vi "mainHRScan.vi"() -> ()   [LabVIEW 2024]
doc: "Main VI for FLS imaging system."
uses:
  <userlib>/_OpenG.lib/file/file.llb/openg_file.lvlib
  <vilib>/event_ctls.llb/usereventprio.ctl
  <instrlib>/niScope/Acquire/Fetch/niScope Multi Fetch Binary 16.vi
  <instrlib>/niScope/Controls/niScope trigger source.ctl
  <userlib>/_OpenG.lib/time/time.llb/openg_time.lvlib
  LaguerreDeconLib/DeconEngineClass/LaguerreDeconEngineClass.lvclass
  SubVI/GlobalVariables.vi
  SubVI/LabJack/LJ Pin Setting.ctl
  <vilib>/Utility/error.llb/DialogType.ctl
  <vilib>/Analysis/NI_AALBase.lvlib
  <vilib>/Utility/miscctls.llb/LVMinMaxIncTypeDef.ctl
  <vilib>/Analysis/baseanly.llb/Mean (DBL).vi
  <vilib>/Utility/miscctls.llb/LVPointTypeDef.ctl
  SubVI/APD/APDClass.lvclass
  ConfigFiles/AimingBeamVideoConfig.ctl
  <instrlib>/niScope/Controls/niScope vertical coupling.ctl
  <vilib>/Instr/_visa.llb/VISA Configure Serial Port (Instr).vi
  <instrlib>/niScope/Configure/Trigger/niScope Configure Trigger Software.vi
  <instrlib>/niScope/Acquire/Fetch/niScope Fetch Binary 8.vi
  SubVI/DigitizerConfiguration/FLImDAQ.ctl
panel:
  out "WF saved":i32
  out "EncoderGraph":dbl[](graph)
  out "error out 3":errorcluster
  out "error out 2":errorcluster
  out "error out":errorcluster
  out "Record Backlog 2":i32
  out "RunStartTime":u32
  out "Dig1 Temp":dbl
  out "Dig2 Temp":dbl
  out "Visualization PC video source":T1
  out "SNR3":dbl format="%#_3g"
  out "SNR2":dbl format="%#_3g"
  out "SNR1":dbl format="%#_3g"
  in  "Show BG removed?":bool=TRUE
  out "IntR3":dbl format="%#_2g"
  out "IntR2":dbl format="%#_2g"
  out "IntR1":dbl format="%#_2g"
  out "Gain3":dbl
  out "Gain2":dbl
  out "Gain1":dbl
  in  "Skip Data Save?":bool=TRUE
  out "Aq Loop?":bool
  out "ML?":bool
  out "aquisition loop Error Out":errorcluster
  out "Record Backlog 1":i32 caption="Record Backlog"
  out "Fetch Record #":i32
  out "Disclamer":picture
  out "Calibration #":i8
  out "BG #":i8
  out "Help":string
  in  "355nm Laser toggle":bool caption="355nm 2500Hz"
  in  "Cali&iRF alignment":bool
  in  "Background":bool
  in  "Aiming beam toggle":bool caption="445nm 15Hz 15mA"
  out "Run #":i8
  in  "StopButton":bool caption="Stop"
  out "Aquisition Status:":bool
  in  "StartButton":bool caption="Start"
  in  "V 3":dbl=1.0 caption="Gain 3" min=0.0 max=4.6494 step=0.1
  in  "V 2":dbl=1.0 caption="Gain 2" min=0.0 max=4.61 step=0.1
  in  "V 1":dbl=1.0 caption="Gain 1" min=0.0 max=4.6492 step=0.1 format="%#_4g"
  out "Case #":string
  out "System Hardware Connection Status":T2
  out "Channel 3":dbl[][](graph)
  out "Channel 2":dbl[][](graph)
  out "Channel 1":dbl[][](graph)
  in  "Tab Control":T3(tab)
  out "display loop timing(ms)":u32
  out "Aquisition loop timing(ms)":u32 format="%.2f"
  out "DisplayLoopIdx":i32 caption="DisplayLoop"
  out "laser EM lamp V":dbl format="%0.6f"
  out "Auisition Loop idx":i32
  out "DataTransferTime":u32
  in  "EncoderDAQ name":refnum<k15>="PXI1Slot2"
  in  "channels":string="0"
  in  "input impedance":u32(ring) items=["1 mega ohm"=0, "50 ohms"=2]
  in  "vertical range":dbl=10.0 format="%.2f"
  in  "min sample rate":dbl=50000.0 format="%^.2e"
  in  "EncoderSampleInterval(s)":dbl=1.0
  out "EncoderDataLength":u32
  in  "Show BG":bool
  out "iRF length":i32
  out "BG length":i32
  out "data length":i32
  out "SysConfigCluster":T4
  out "LJ Pinout":T5={"Ch1 Bias"="DAC0", "Ch2 Bias"="DAC1", "Ch3 Bias"="DAC2", "Ch4 Bias"="DAC0", "355 PWM"="FIO0", "AimingBeam PWM"="FIO2", "Laser Ready"="FIO3", "Interlock"="FIO1", "Laser Start/Stop"="FIO1", "Red LED"="FIO1", "Green LED"="DIO3", "Foot Pedal"="DIO15"}
  out "FLImDAQ":T6={"Digitizer 1"="", "Digitizer 2"="", "Channel"=enum."Channel 0", "trigger source"="VAL_EXTERNAL", "trigger level"=0.5, "trigger delay"=1.35e-07, "min sample rate"=12500000000.0, "min record length"=2500, "vertical range"=1.0, "vertical offset"=-0.25, "Waveform to Avg"=2000} caption="FLIm DAQ Configuration" {"trigger delay" format="%^#.4e"; "trigger level" min=0.0 max=3.5 step=0.5 format="%.2f"; "vertical offset" format="%.4f"; "vertical range" format="%.2f"; "min sample rate" format="%#.2p"}
  in  "Sys Reconfig":bool
  out "Vertical Range 1":dbl
  out "Vertical Offset 1":dbl
  out "Vertical Range 2":dbl
  out "Vertical Offset 2":dbl
  out "Laser Rep Rate":dbl
  in  "Data Class":enum16{"Data", "BG", "Cali"}(ring)
  out "V1 Size":i32
  out "V2 Size":i32
  out "V3 Size":i32
  out "data Size":i32[](array[numeric])
  out "State log":string
  in  "Quit":bool
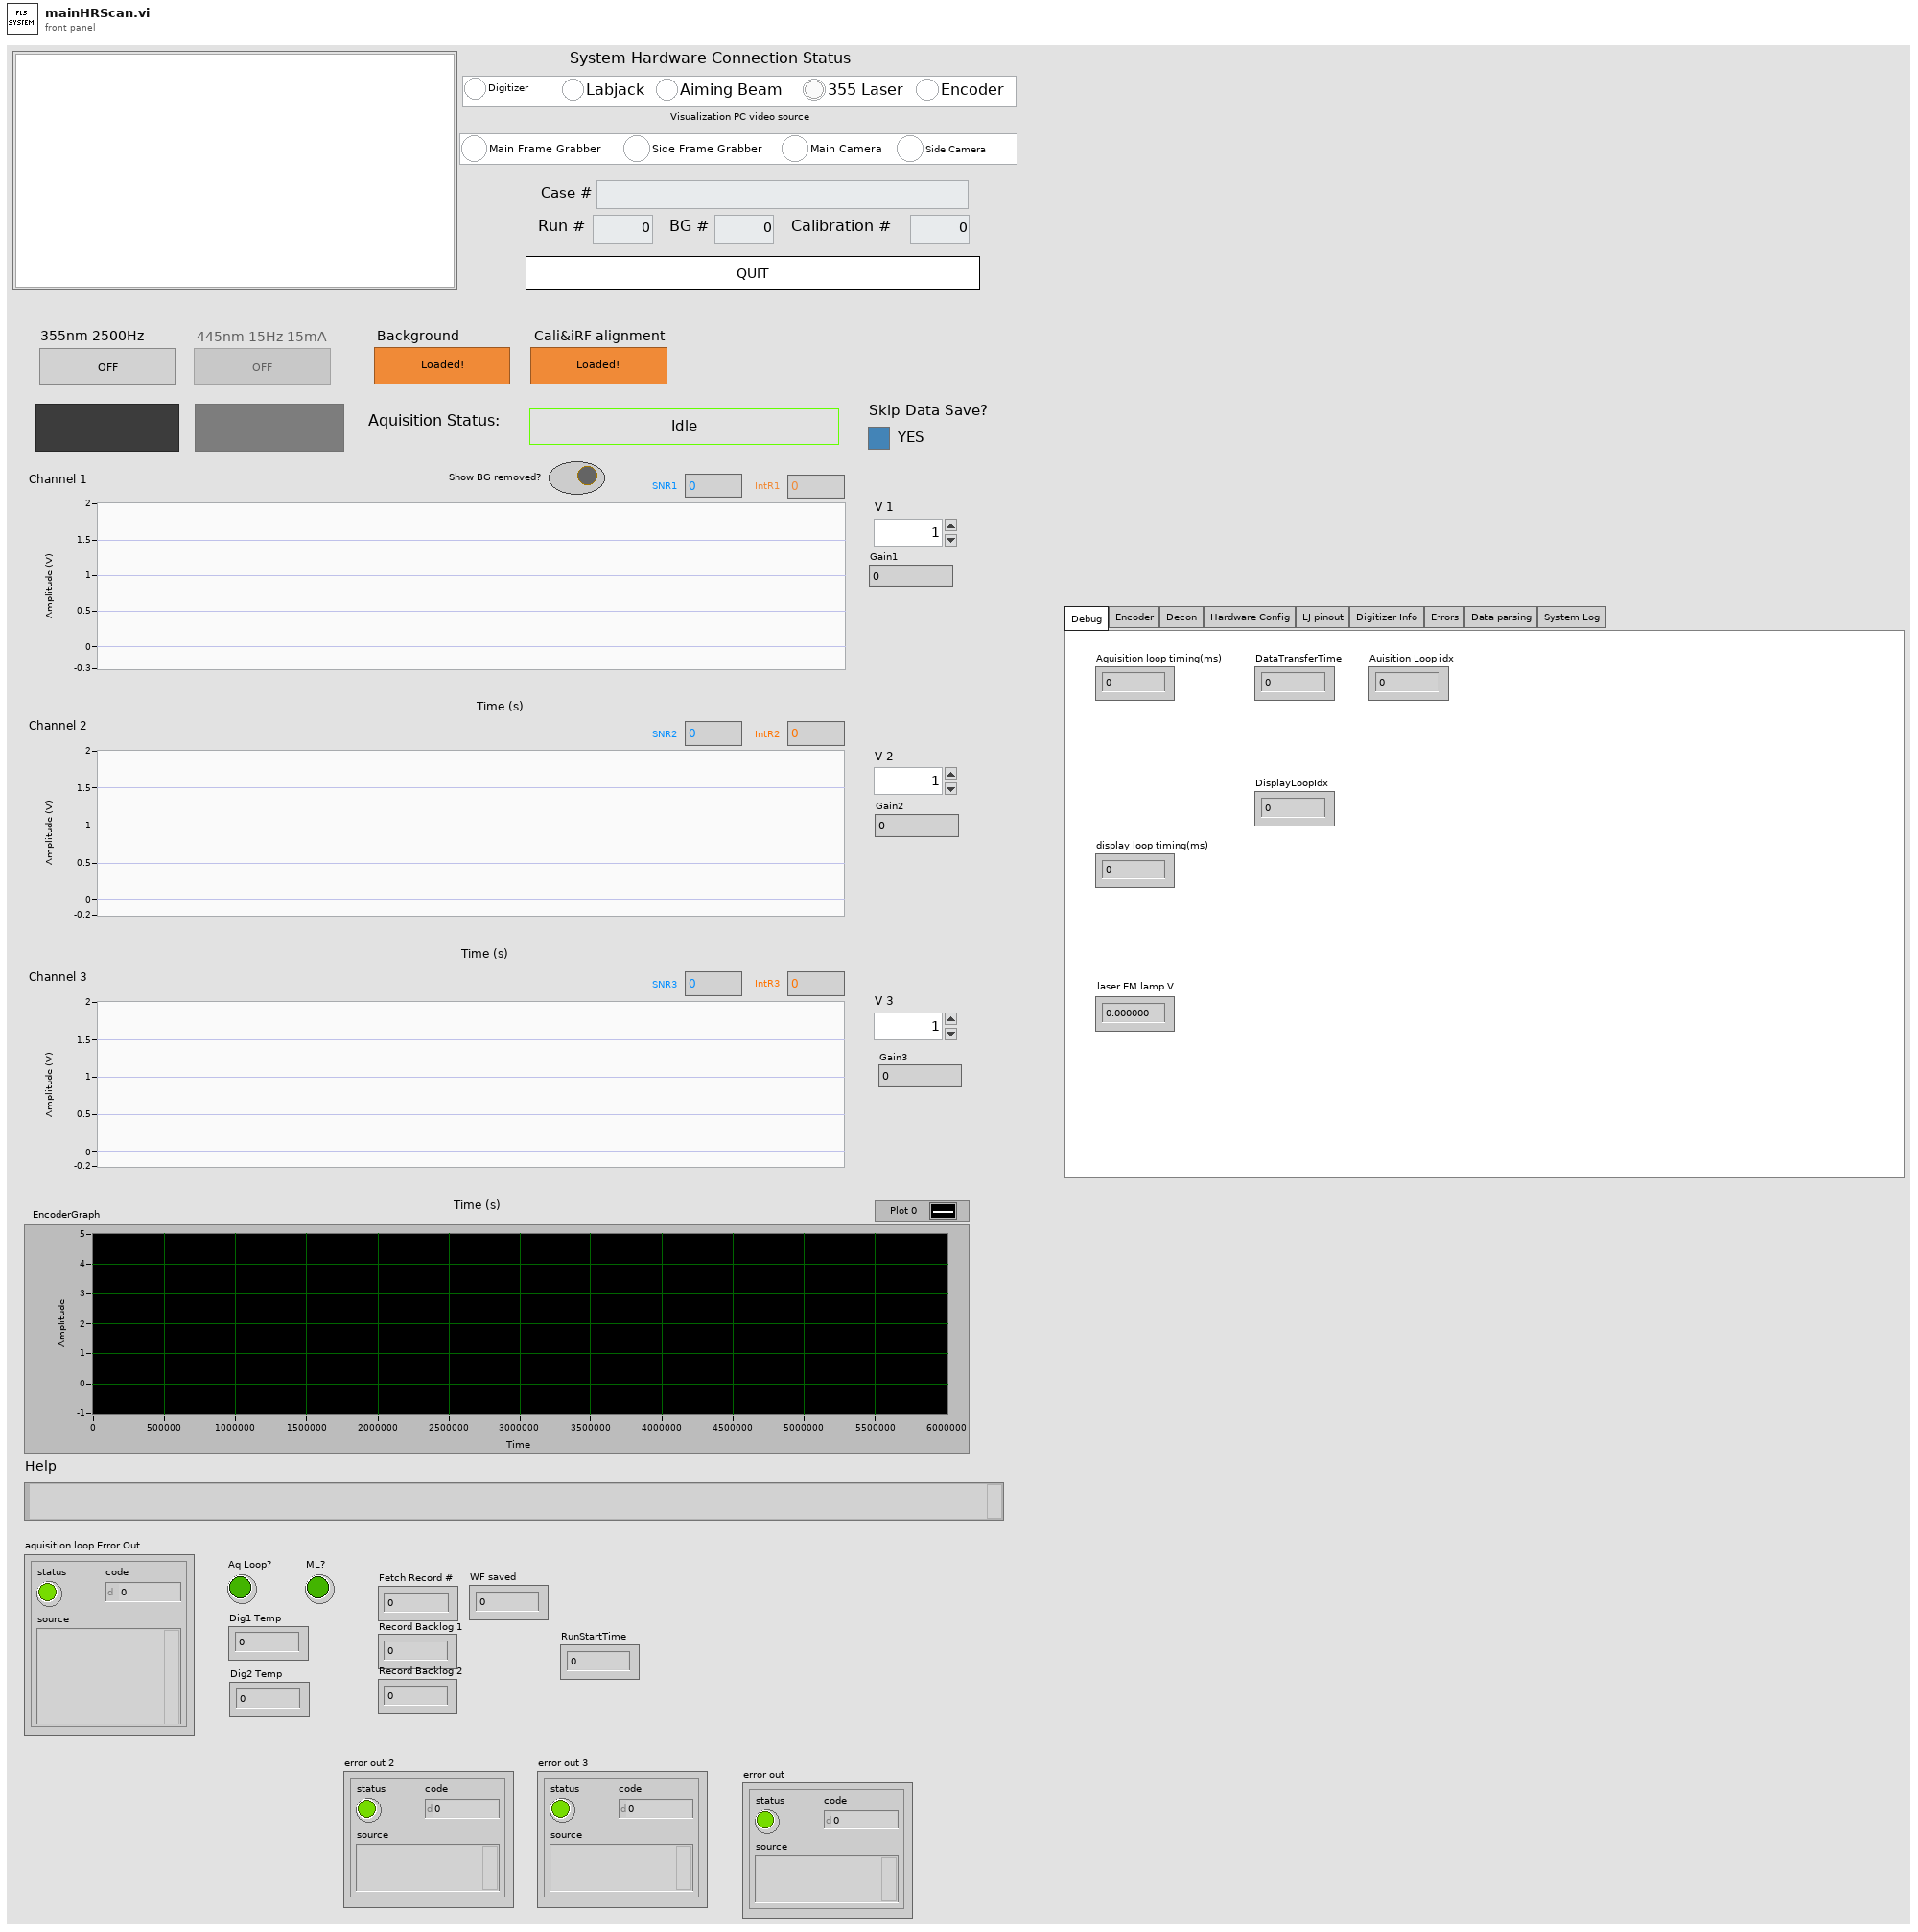
[diagram p1: front panel]
types:
  T1 = cluster{"Main Frame Grabber":bool, "Side Frame Grabber":bool, "Main Camera":bool, "Side Camera":bool}
  T2 = cluster{"Digitizer":bool, "Labjack":bool, "Aiming Beam":bool, "355 Laser":bool, "Encoder":bool}
  T3 = enum32{"Debug", "Encoder", "Decon", "Hardware Config", "LJ pinout", "Digitizer Info", "Errors", "Data parsing", "System Log"}
  T4 = cluster{"Ch1Enable?":bool, "Ch2Enable?":bool, "Ch3Enable?":bool, "Ch1AutoGain?":bool, "Ch2AutoGain?":bool, "Ch3AutoGain?":bool, "AimingBeamEnable?":bool}
  T5 = typedef "LJ Pin Setting.ctl" = cluster{"Ch1 Bias":string, "Ch2 Bias":string, "Ch3 Bias":string, "Ch4 Bias":string, "355 PWM":string, "AimingBeam PWM":string, "Laser Ready":string, "Interlock":string, "Laser Start/Stop":string, "Red LED":string, "Green LED":string, "Foot Pedal":string}
  T6 = typedef "FLImDAQ.ctl" = cluster{"Digitizer 1":refnum<k15>, "Digitizer 2":refnum<k15>, "Channel":enum16{"Channel 0", "Channel 1", "Channel 0&1"}, "trigger source":T7, "trigger level":dbl, "trigger delay":dbl, "min sample rate":dbl, "min record length":i32, "vertical range":dbl, "vertical offset":dbl, "Waveform to Avg":i16}
  T7 = typedef "niScope trigger source.ctl" = string
  T8 = cluster{"remote start event":refnum<user-event>, "remote stop  event":refnum<user-event>}
  T9 = enum16{"open", "replace", "create", "open or create", "replace or create", "replace or create with confirmation"}
  T10 = cluster{"idx":i32, "CH1&2":i16[][], "CH3":i16[][], "V cluster":cluster{"V1":dbl, "V2":dbl, "V3":dbl}}
  T11 = cluster{"Ch1 WF":dbl[], "Ch2 WF":dbl[], "Ch3 WF":dbl[], "V1":dbl, "V2":dbl, "V3":dbl}
  T12 = enum16{"open", "open or create", "create or replace", "create", "open (read-only)"}
  T13 = enum32{"Invalid", "Standard", "Closed", "Hidden", "Minimized", "Maximized"}
  T14 = enum32{"invalid app kind", "Development System", "Run Time System", "Student Edition", "Embedded LabVIEW", "Evaluation", "Custom"}
  T15 = typedef "usereventprio.ctl" = enum32{"high priority", "normal priority"}
  T16 = enum32{"Bad", "Idle", "Run top level", "Running"}
  T17 = enum8{"Enabled", "Disabled", "Disabled and Grayed Out"}
  T18 = typedef "AimingBeamVideoConfig.ctl" = cluster{"DeCon Channel":enum16{"1", "2", "3"}, "Scale Bar":bool, "Scale Low":dbl, "Scale High":dbl, "ANSI":dbl, "Radius":dbl, "3D?":bool, "Firefly?":bool, "Pentero?":bool}
  T19 = cluster{"Core":cluster{"Current VI Reference":refnum<vi>, "Close Panel on Exit?":bool}, "SysConfigCluster":cluster{"Ch1Enable?":bool, "Ch2Enable?":bool, "Ch3Enable?":bool, "Ch1AutoGain?":bool, "Ch2AutoGain?":bool, "Ch3AutoGain?":bool, "AimingBeamEnable?":bool}, "System Status":cluster{"Digitizer":bool, "Labjack":bool, "Aiming Beam":bool, "355 Laser":bool, "Encoder":bool}, "IDs":cluster{"RunID":i8, "BG ID":i8, "Cali ID":i8}, "CaseID":string, "DefaultPath":path, "Pathes":cluster{"DataPath":path, "BG Path":path, "iRFPath":path, "CaliPath":path}, "FLImDAQ":cluster{"resource name":refnum<k15>, "resource name 2":refnum<k15>, "Channel":enum16{"Channel 0", "Channel 1", "Channel 0&1"}, "trigger source":T7, "trigger level":dbl, "trigger delay":dbl, "min sample rate":dbl, "min record length":i32, "vertical range":dbl, "vertical offset":dbl, "Waveform to Avg":i32}, "SysRunning?":bool, "AB Cluster":cluster{"Aiming Beam COM Port":refnum<visa-resource-name>, "Min Current":dbl, "Max Current":dbl, "Default Current":dbl, "Freq":i32}, "LJ Pinout":T5, "355 PWM setting":cluster{"DIO_EF_CLOCK1_DIVISOR":i16, "DIO_EF_CLOCK1_ROLL_VALUE":i32, "DIO#_EF_INDEX":i16, "DIO#_EF_OPTIONS":i16, "DIO#_EF_CONFIG_A":i32}, "AB PWM setting":cluster{"DIO_EF_CLOCK1_DIVISOR":i16, "DIO_EF_CLOCK1_ROLL_VALUE":i32, "DIO#_EF_INDEX":i16, "DIO#_EF_OPTIONS":i16, "DIO#_EF_CONFIG_A":i32}, "Last Trigger":u32, "niTClk sessions":refnum<k20>[], "Laser start tic":u32, "TCP attempt count":i32, "Ch1Data":dbl[][], "Ch2Data":dbl[][], "Ch3Data":dbl[][], "V1":dbl[], "V2":dbl[], "V3":dbl[], "SlowTimer":u32, "FastTimer":u32, "listener ID":refnum<k5>, "TempPath":path, "LED vi reference":refnum<vi>, "Aquisition Timer":u32, "APDSerialNum":cluster{"Ch1APDSerial#":string, "Ch2APDSerial#":string, "Ch3APDSerial#":string}, "VideoConfig":T18, "CaliPath":path, "LED vi ref open?":bool, "video source":cluster{"Main Frame Grabber":bool, "Side Frame Grabber":bool, "Main Camera":bool, "Side Camera":bool}, "bothVidSourceAvail":bool, "EncoderDAQ":refnum<k15>, "TDMS group name":string}
  T20 = typedef "LVCursorListTypeDef.ctl" = cluster{"Name":string, "Color":u32, "Style":u8, "Point Style":u8, "Name Visible":bool, "Allow Drag":bool, "Cursor Mode":u32, "Plot":i32, "Index":i32, "Position":cluster{"X":dbl, "Y":dbl}, "X Scale":u32, "Y Scale":u32, "Watch Plots":i32[], "Watch All Plots":bool, "Plot Area":i32, "Label Offset":cluster{"X":dbl, "Y":dbl}}[]
  T21 = cluster{"Name":string, "Color":u32, "Style":u8, "Point Style":u8, "Name Visible":bool, "Allow Drag":bool, "Cursor Mode":u32, "Plot":i32, "Index":i32, "Position":cluster{"X":dbl, "Y":dbl}, "X Scale":u32, "Y Scale":u32, "Watch Plots":i32[], "Watch All Plots":bool, "Plot Area":i32, "Label Offset":cluster{"X":dbl, "Y":dbl}}
  T22 = cluster{"Ch1APDSerial#":string, "Ch2APDSerial#":string, "Ch3APDSerial#":string}
  T23 = cluster{"DataPath":path, "BG Path":path, "iRFPath":path, "CaliPath":path}
  T24 = cluster{"DIO_EF_CLOCK1_DIVISOR":i16, "DIO_EF_CLOCK1_ROLL_VALUE":i32, "DIO#_EF_INDEX":i16, "DIO#_EF_OPTIONS":i16, "DIO#_EF_CONFIG_A":i32}
  T25 = cluster{"Aiming Beam COM Port":refnum<visa-resource-name>, "Min Current":dbl, "Max Current":dbl, "Default Current":dbl, "Freq":i32}
  T26 = cluster{"resource name":refnum<k15>, "resource name 2":refnum<k15>, "Channel":enum16{"Channel 0", "Channel 1", "Channel 0&1"}, "trigger source":T7, "trigger level":dbl, "trigger delay":dbl, "min sample rate":dbl, "min record length":i32, "vertical range":dbl, "vertical offset":dbl, "Waveform to Avg":i32}
  T27 = cluster{"Current VI Reference":refnum<vi>, "Close Panel on Exit?":bool}
  T28 = typedef "iRFData.ctl" = cluster{"dt":dbl, "NumOfWFs":i32, "WFLength":i32, "iRFCtrlV":dbl[], "iRFWFsAvg":dbl[][], "iRFRaw":dbl[][]}
  T29 = cluster{"iRFWFsAvg":dbl[], "iRFWFsAvg":dbl[], "iRFWFsAvg":dbl[]}
  T30 = cluster{"V 1":dbl[], "V 2":dbl[], "V 3":dbl[], "V 4":dbl[]}
  T31 = cluster{"Channel 1":dbl[], "Channel 2":dbl[], "Channel 3":dbl[], "Channel 4":dbl[]}
  T32 = cluster{"DataPath":path, "CaseID":string, "RunID":i8, "Ch1Data":dbl[][], "Ch2Data":dbl[][], "Ch3Data":dbl[][], "V1":dbl[], "V2":dbl[], "V3":dbl[], "LaserRepRate":u32, "WFAverage":i16, "RunStartTime":u32}
  T33 = typedef "DialogType.ctl" = u16
  T34 = cluster{"Ch1 iRF":dbl[], "Ch2 iRF":dbl[], "Ch3 iRF":dbl[], "Ch4 iRF":dbl[]}
  T35 = cluster{"Ch1APDSerial#":string, "Ch2APDSerial#":string, "Ch3APDSerial#":string, "Ch4APDSerial#":string}
  T36 = typedef "LJ PWM Setting.ctl" = cluster{"DIO_EF_CLOCK1_DIVISOR":i16, "DIO_EF_CLOCK1_ROLL_VALUE":i32, "DIO#_EF_INDEX":i16, "DIO#_EF_OPTIONS":i16, "DIO#_EF_CONFIG_A":i32}
  T37 = typedef "AimingBeam.ctl" = cluster{"Aiming Beam COM Port":refnum<visa-resource-name>, "Min Current":dbl, "Max Current":dbl, "Default Current":dbl, "Frequency(Hz)":u32}
  T38 = cluster{"DC1":i32, "DC2":i32, "BG1":i32, "BG2":i32}
  T39 = typedef "LVMinMaxIncTypeDef.ctl" = cluster{"Minimum":dbl, "Maximum":dbl, "Increment":dbl}
  T40 = typedef "LVBoundsTypeDef.ctl" = cluster{"Width":u32, "Height":u32}
  T41 = typedef "imagedata.ctl" = cluster{"image type":i32, "image depth":i32, "image":u8[], "mask":u8[], "colors":u32[], "Rectangle":cluster{"left":i16, "top":i16, "right":i16, "bottom":i16}}
  T42 = cluster{"DC Idx1":i32, "DC Idx2":i32, "BG Idx1":i32, "BG Idx2":i32}
  T43 = typedef "niScope vertical coupling.ctl" = i32
  T44 = cluster{"actualSamples":i32, "absoluteInitialX":dbl, "relativeInitialX":dbl, "xIncrement":dbl, "offset":dbl, "gain":dbl, "reserved1":dbl, "reserved2":dbl}
  T45 = typedef "LVPointTypeDef.ctl" = cluster{"Horizontal":i16, "Vertical":i16}
  T46 = cluster{"V1 out":dbl, "V2 out":dbl, "V3 out":dbl}
  T47 = cluster{i32, i16[][], i16[][], cluster{"V1 out":dbl, "V2 out":dbl, "V3 out":dbl}}
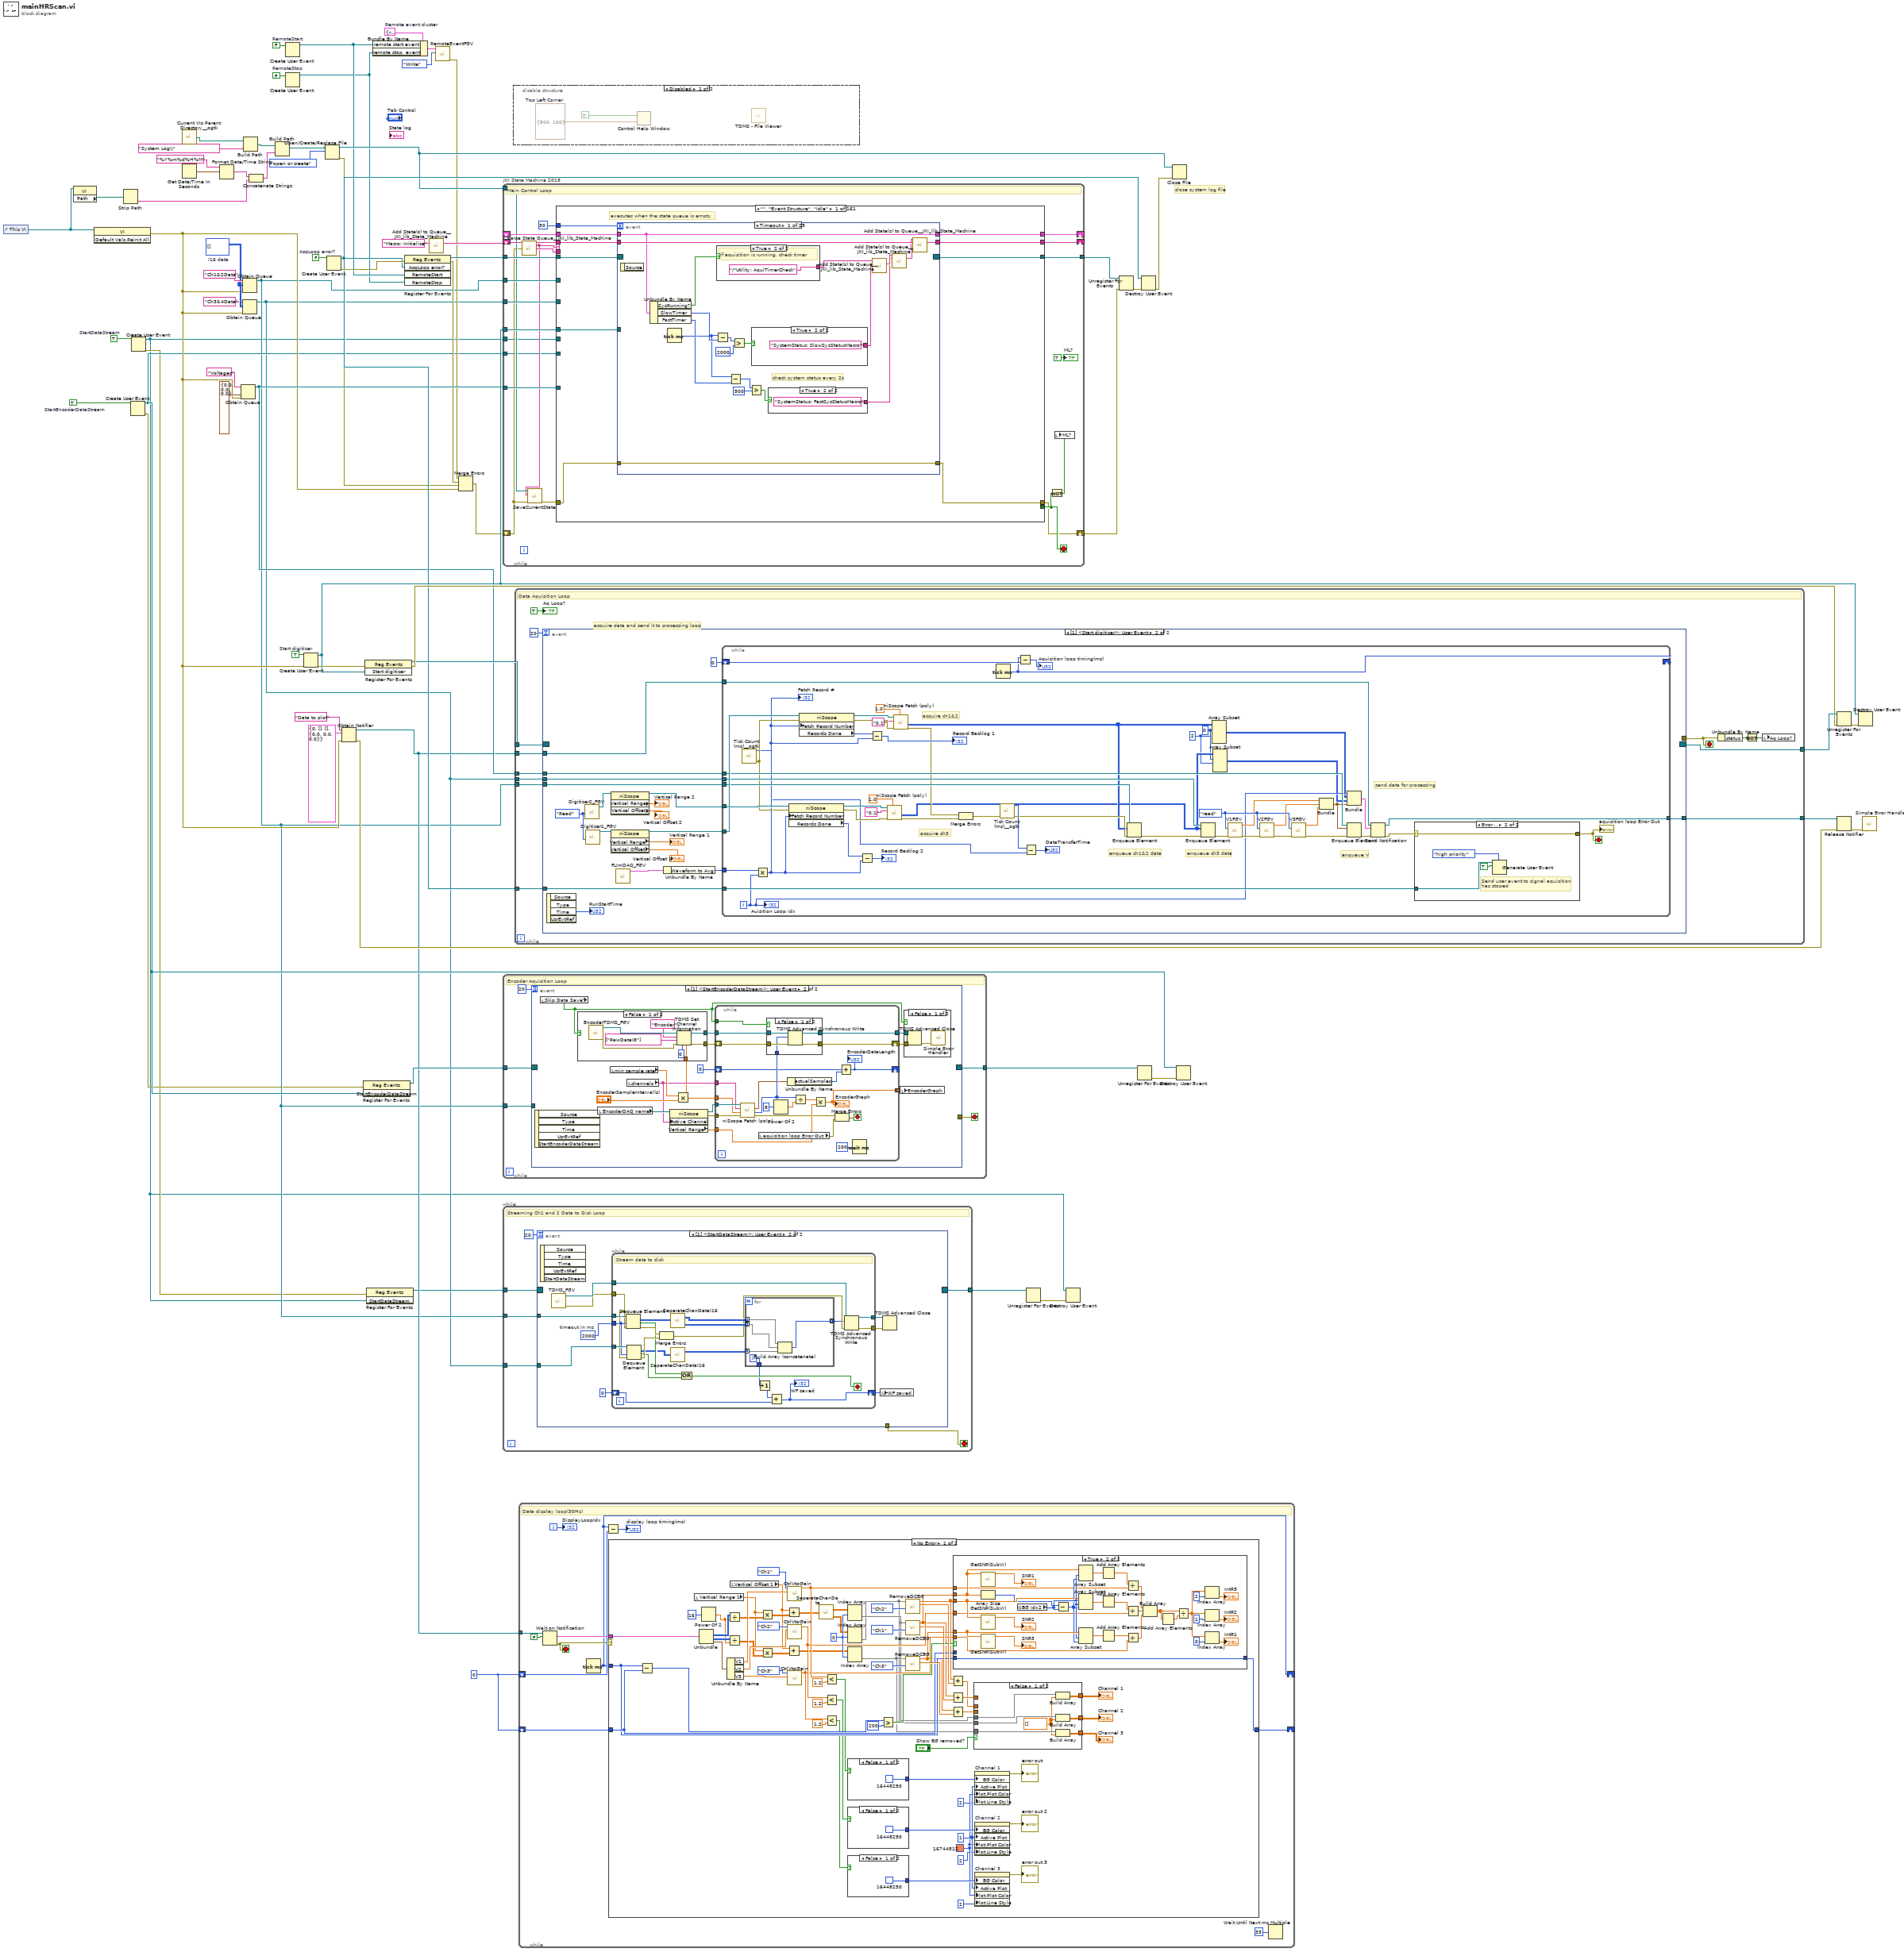
[diagram p0: block diagram]
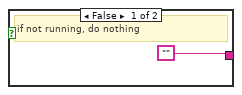
[diagram p2: hidden frame]
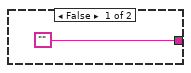
[diagram p3: hidden frame]
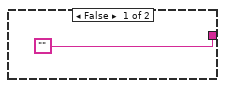
[diagram p4: hidden frame]
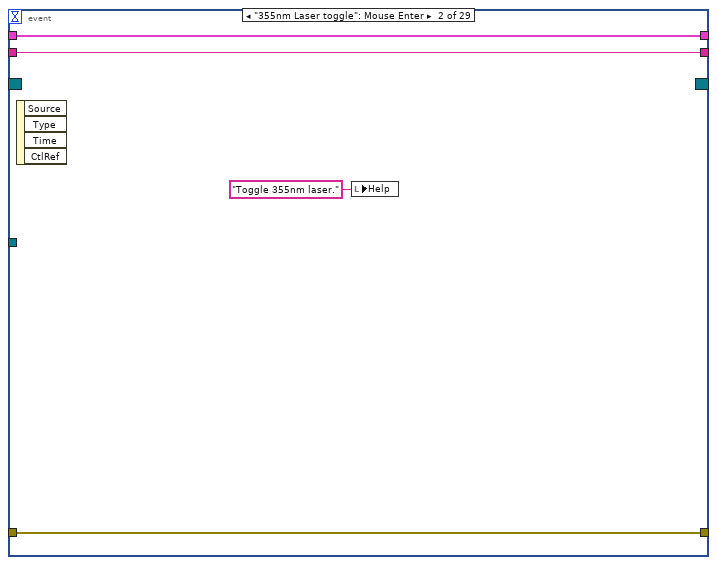
[diagram p5: hidden frame]
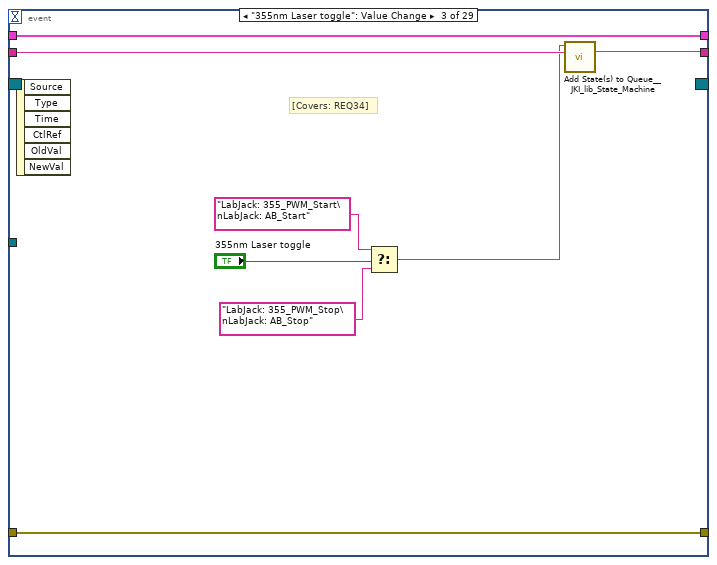
[diagram p6: hidden frame]
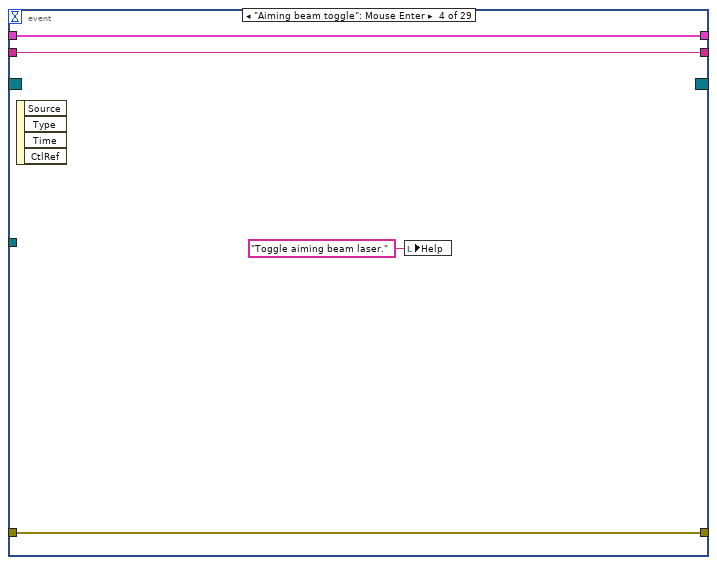
[diagram p7: hidden frame]
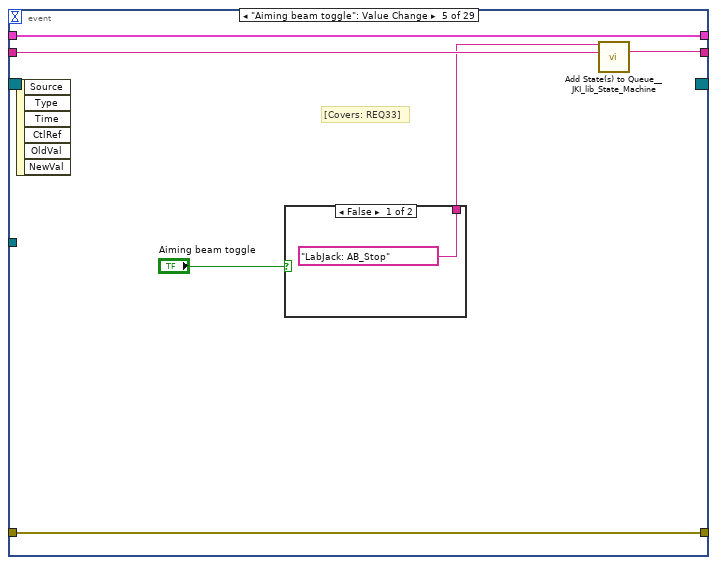
[diagram p8: hidden frame]
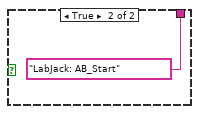
[diagram p9: hidden frame]
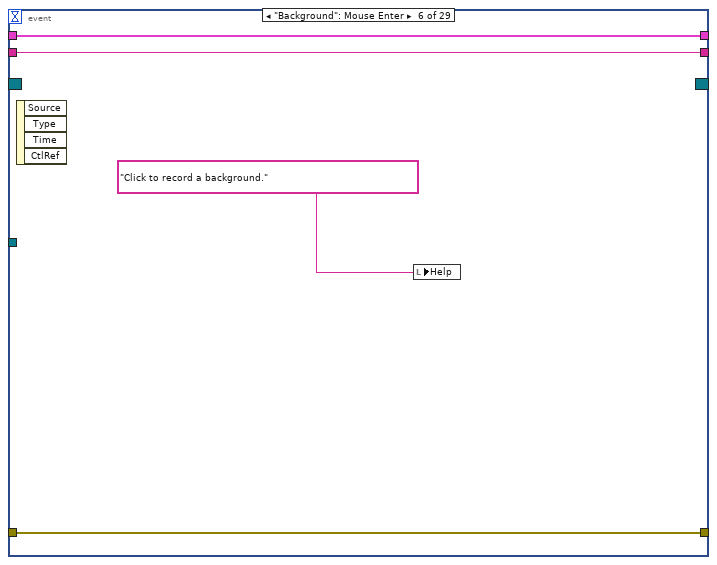
[diagram p10: hidden frame]
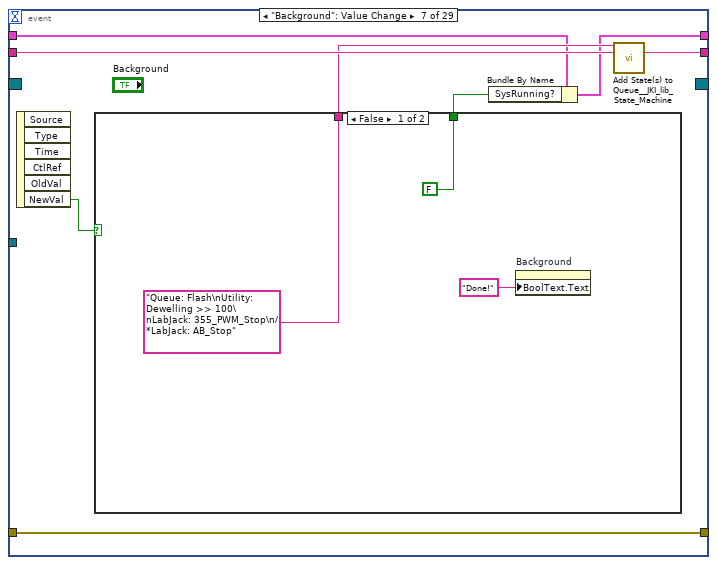
[diagram p11: hidden frame]
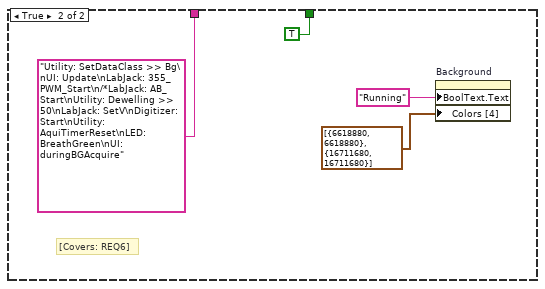
[diagram p12: hidden frame]
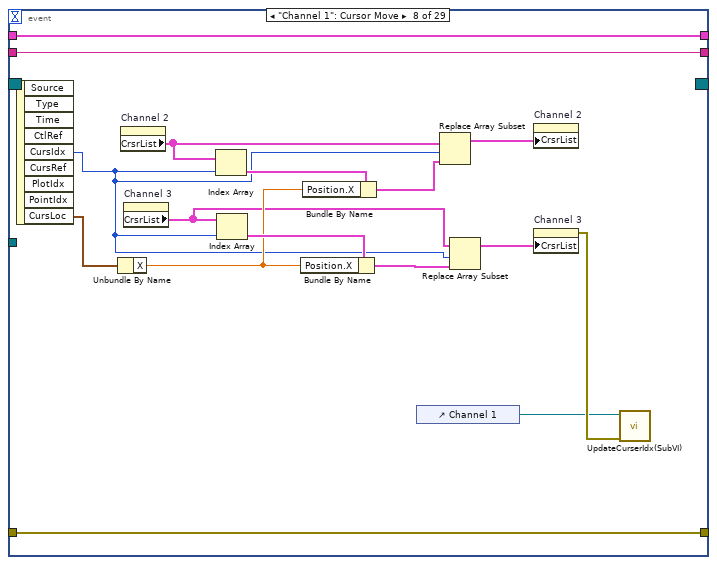
[diagram p13: hidden frame]
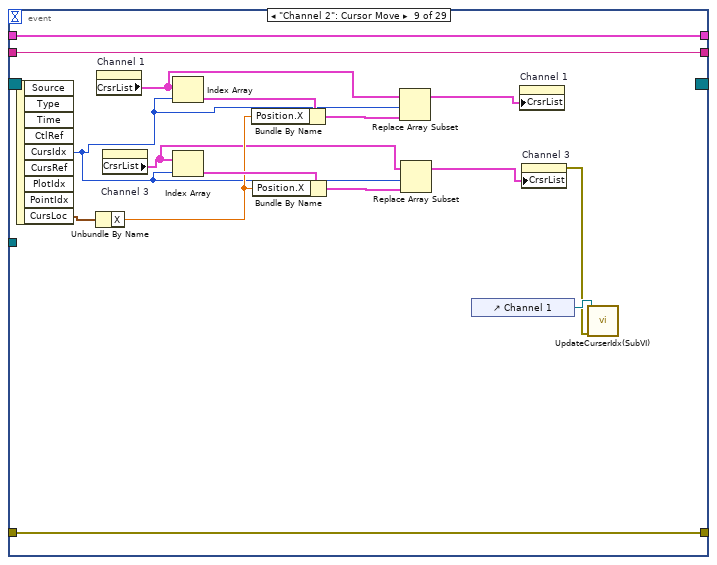
[diagram p14: hidden frame]
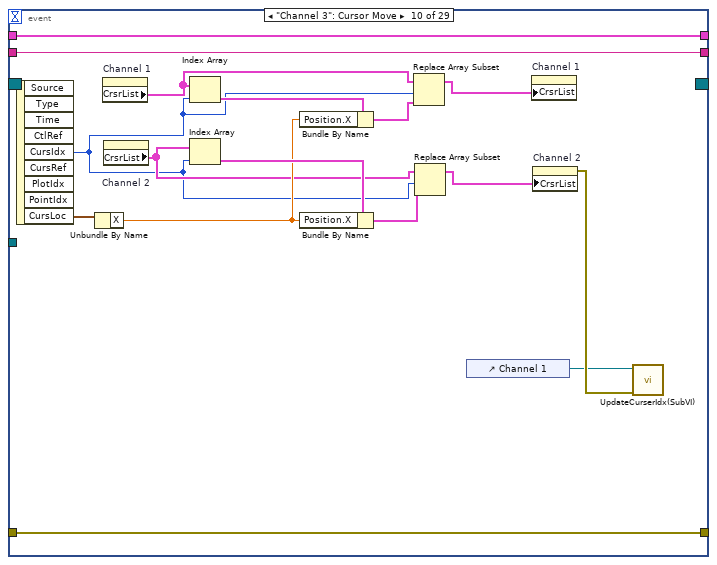
[diagram p15: hidden frame]
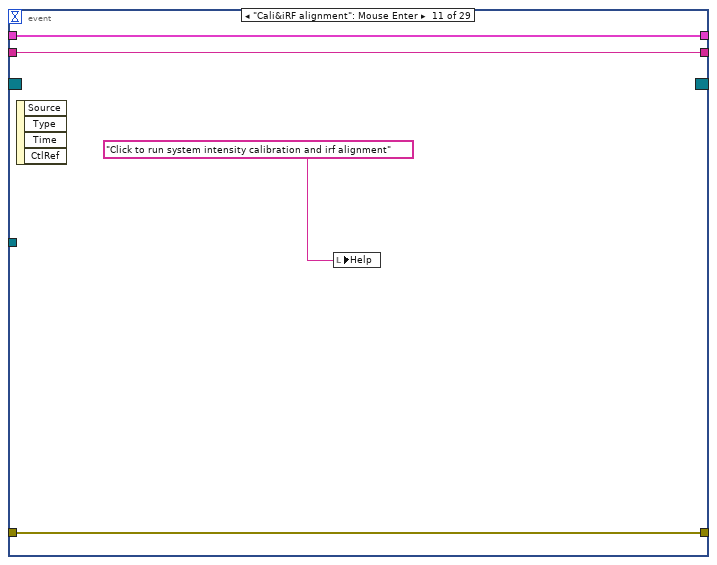
[diagram p16: hidden frame]
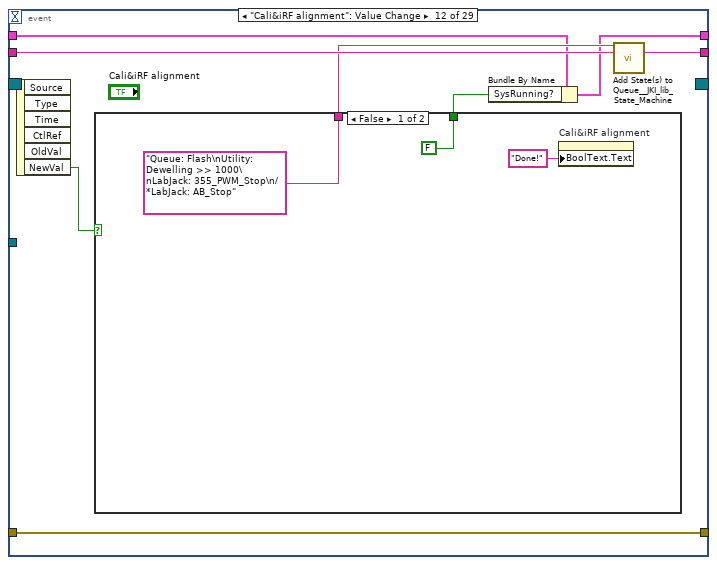
[diagram p17: hidden frame]
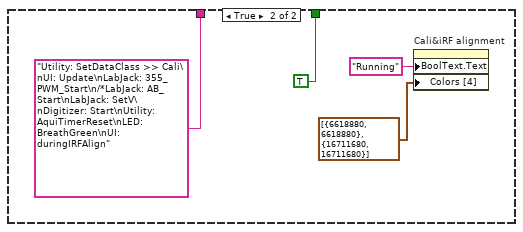
[diagram p18: hidden frame]
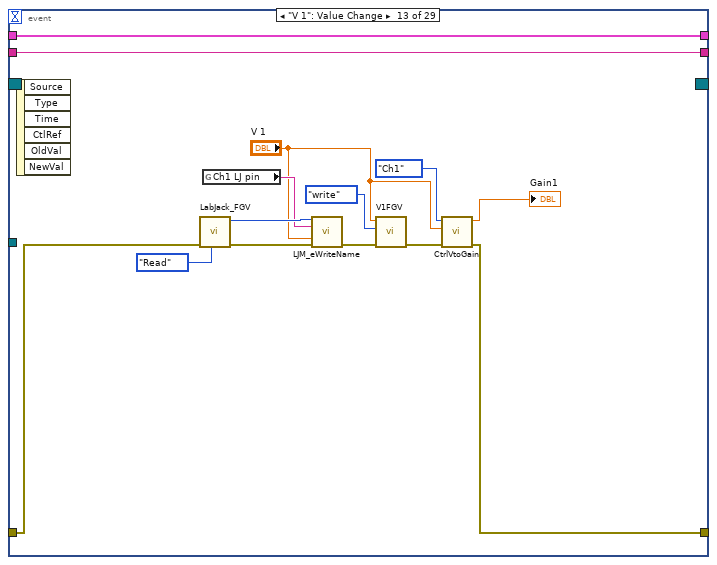
[diagram p19: hidden frame]
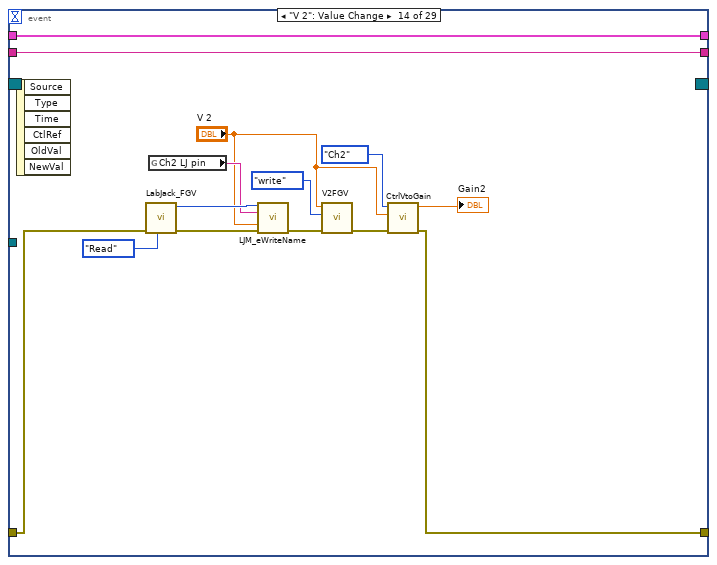
[diagram p20: hidden frame]
diagram:
  w11 = TRUE  # StartDataStream
  w18 = TRUE  # StartEncoderDataStream
  w25 = T8 {"remote start event"=refnum, "remote stop  event"=refnum}  # Remote event cluster
  w28 = FALSE  # RemoteStop
  w29 = FALSE  # RemoteStart
  w30 = u32 0 ("millisecond timer value")
  w54 = FALSE  # AcqLoop error?
  w64 = TRUE  # Start digitizer
  w66 = i16[][] []  # I16 data
  # "close system log file"
  n1 = control-ref of="This VI"() -> (w3:refnum<vi>)
  n2 = property class="VI"(reference=w3) -> ("Path"=w2:path)  [unwired: 1 in, 2 out]
  n3 = invoke on="Invoke Node" class="VI" method="Default Vals.Reinit All"(reference=w3) -> (error out=w33:errorcluster)  [unwired: 2 in, 2 out]
  n4 = Strip Path(path=w2) -> (name=w1:string)  [unwired: 1 out]
  n5 = Create User Event(user event datatype=w18) -> (user event=w14:refnum<user-event>, error out=w10:errorcluster)  [unwired: 1 in]
  n6 = Create User Event(user event datatype=w11) -> (user event=w4:refnum<user-event>, error out=w9:errorcluster)  [unwired: 1 in]
  n7 = call <userlib>:"Current VIs Parent Directory__ogtk.vi"() -> ("Parent Directory (+ Relative)"=w43:path)  [unwired: 5 in]
  n8 = Get Date/Time In Seconds() -> (seconds since 1Jan1904=w41:timestamp)
  n9 = Format Date/Time String(time format string (%c)="%Y%m%d%H%M", seconds (now)=w41) -> (date/time string=w38:string)  [unwired: 1 in]
  n10 = Obtain Queue(name (unnamed)="Voltages", element data type=cluster{"V1":dbl, "V2":dbl, "V3":dbl} {"V1"=0.0, "V2"=0.0, "V3"=0.0}, error in (no error)=w33) -> (queue out=w44:refnum<queue>)  [unwired: 2 in, 2 out]
  n11 = Obtain Queue(name (unnamed)="Ch3&4Data", element data type=w66, error in (no error)=w33) -> (queue out=w5:refnum<queue>)  [unwired: 2 in, 2 out]
  n12 = Obtain Queue(name (unnamed)="Ch1&2Data", element data type=w66, error in (no error)=w33) -> (queue out=w12:refnum<queue>)  [unwired: 2 in, 2 out]
  n13 = Build Path(base path=w43, name or relative path="System Log\\") -> (appended path=w35:path)
  n14 = Concatenate Strings(w38, w1) -> (w37:string)
  n15 = Build Path(base path=w35, name or relative path=w37) -> (appended path=w39:path)
  n16 = Create User Event(user event datatype=w29) -> (user event=w27:refnum<user-event>)  [unwired: 1 in, 1 out]
  n17 = Create User Event(user event datatype=w28) -> (user event=w26:refnum<user-event>)  [unwired: 1 in, 1 out]
  n18 = Create User Event(user event datatype=w64, error in=w33) -> (user event=w53:refnum<user-event>, error out=w48:errorcluster)
  n19 = Open/Create/Replace File(file path (use dialog)=w39, operation (0:open)=T9."open or create") -> (refnum out=w31:refnum<file>, error out=w32:errorcluster)  [unwired: 4 in, 1 out]
  n20 = Create User Event(user event datatype=w54) -> (user event=w47:refnum<user-event>, error out=w49:errorcluster)  [unwired: 1 in]
  n21 = Obtain Notifier(name (unnamed)="Data to plot", notification data type=T10 {"idx"=0, "CH1&2"=[], "CH3"=[], "V cluster"={"V1"=0.0, "V2"=0.0, "V3"=0.0}}, error in (no error)=w33) -> (notifier out=w13:refnum<notifier>, error out=w58:errorcluster)  [unwired: 1 in, 1 out]
  n22 = register-events(error in=w10, w14) -> (reference out=w17:refnum<event-registration>)  [unwired: 1 in, 1 out]
  n23 = register-events(error in=w48, w53) -> (reference out=w55:refnum<event-registration>, error out=w61:errorcluster)  [unwired: 1 in]
  n24 = register-events(error in=w9, w4) -> (reference out=w8:refnum<event-registration>)  [unwired: 1 in, 1 out]
  n25 = Bundle By Name(cluster=w25, "remote start event"=w27, "remote stop  event"=w26) -> (w23:T8)
  n26 = register-events(error in=w49, w47, w27, w26) -> (reference out=w51:refnum<event-registration>, error out=w22:errorcluster)  [unwired: 1 in]
  n27 = call <vilib>:"Add State(s) to Queue__JKI_lib_State_Machine.vi"("State(s) in (\"\")"="Macro: Initialize") -> ("States Out"=w69:string)  [unwired: 14 in]
  n28 = call "RemoteEventFGV.vi"("Operation (Read)"=enum16{"Read", "Write"}."Write", "Remote Event in"=w23) -> ("Error Out"=w19:errorcluster)  [unwired: 8 in, 1 out]
  n29 = Merge Errors(w19, w22, w32, w33) -> (w34:errorcluster)
  n30 = while "JKI State Machine 2018" {
    shift-right: [w88] -> _
    shift-left: _ -> [w87]
    shift-right: [w72] -> w21
    shift-left: w34 -> [w74]
    shift-right: [w89] -> _
    shift-left: w69 -> [w90]
    tunnel: w12 -> [w85]
    tunnel: w5 -> [w84]
    tunnel: w53 -> [w83]
    tunnel: w51 -> [w82]
    tunnel: [w81] -> w50
    tunnel: w44 -> [w77]
    tunnel: w31 -> [w76]
    tunnel: w14 -> [w71]
    tunnel: w4 -> [w70]
    stop <- w80 stop-if-true
    # "Main Control Loop"
    n31 = call <vilib>:"Parse State Queue__JKI_lib_State_Machine.vi"("State Queue"=w90, "Error In (no error)"=w74) -> ("Remaining States"=w92:string, "Current State"=w75:string, "Arguments"=w91:string)  [unwired: 11 in]
    n32 = call "SaveCurrentState.vi"("error in (no error)"=w74, "Current State"=w75, "Byte Stream File in"=w76) -> ("error out"=w73:errorcluster)  [unwired: 8 in]
    n33 = case shown="\"\", \"Event Structure\", \"Idle\"" w75 {
      selector: w75 -> [_ _ _ _ _ _ _ _ _ _ _ _ _ _ _ _ _ _ _ _ _ _ _ _ _ w900 _ _ _ _ _ _ _ _ _ _ _ _ _ _ _ _ _ _ _ _ _ _ _ _ _ _ _ _ _ _ _ _ _ _ _ _ _ _ _ _ _ _ _ _ _ _ _ _ _ _ _ _ _ _ _ _ _ _ _ _ _ _ _ _ _ _ _ _ _ _ _ _ _ _ _ _ _ _ _ _ _ _ _ _ _ _ _ _ _ _ _ _ _ _ _ _ _ _ _ _ _ _ _ _ _ _ _ _ _ _ _ _ _ _ _ _ _ _ _ _ _ _ _ _ _ _ _ _ _ _ _ _ _ _ _]
      tunnel: w92 -> [w102 w374 w382 w401 w410 w416 w422 w445 w460 w502 w536 w551 w580 w618 w630 w654 w682 w694 w720 w733 w799 w837 w880 w893 w898 w904 w931 w939 w962 w967 w980 w999 w1027 w1055 w1093 w1098 w1104 w1130 w1156 w1182 w1187 w1204 w1251 w1274 w1290 w1305 w1315 w1331 w1336 w1348 w1377 w1401 w1413 w1451 w1462 w1468 w1479 w1491 w1522 w1535 w1549 w1564 w1583 w1618 w1623 w1637 w1647 w1663 w1675 w1687 w1715 w1730 w1735 w1746 w1758 w1763 w1771 w1779 w1788 w1797 w1802 w1810 w1819 w1837 w1853 w1873 w1884 w1906 w1920 w1937 w1942 w1950 w1958 w1963 w1971 w1978 w1986 w1993 w2003 w2031 w2039 w2046 w2054 w2059 w2067 w2074 w2080 w2087 w2101 w2106 w2113 w2125 w2195 w2207 w2216 w2233 w2242 w2265 w2282 w2293 w2306 w2331 w2354 w2360 w2376 w2398 w2406 w2412 w2417 w2424 w2434 w2446 w2455 w2460 w2474 w2479 w2484 w2489 w2499 w2521 w2540 w2545 w2556 w2577 w2599 w2618 w2623 w2653 w2665 w2672 w2681 w2686 w2704 w2719 w2747 w2775 w2784 w2789 w2812 w2829 w2834]
      tunnel: w91 -> [_ _ _ _ _ _ _ _ _ _ _ _ _ _ _ _ _ _ _ _ _ _ _ _ _ _ _ _ _ _ _ _ _ _ _ _ _ _ _ _ _ _ _ _ _ _ _ _ _ _ _ _ _ _ _ _ _ w1489 _ _ _ _ _ _ _ _ _ _ _ _ _ _ _ _ _ _ _ _ _ _ _ _ _ _ _ _ _ _ _ _ _ _ _ _ _ _ _ _ w1994 _ _ _ _ _ _ _ _ _ _ _ w2108 w2119 _ _ _ _ w2239 _ _ _ _ _ w2350 _ _ _ _ _ _ w2419 _ _ _ _ w2470 _ _ _ _ _ _ _ _ _ _ _ _ _ _ _ _ _ _ _ _ _ _ _ _ _ _]
      tunnel: w87 -> [w100 w371 w376 w390 w406 w413 w419 w442 w457 _ w533 w541 w576 w614 w626 w646 w672 w691 w717 w730 w758 w829 w867 w888 w895 w902 w924 w936 w960 w964 w968 w989 w1019 w1047 w1089 w1095 w1101 w1108 w1135 w1161 w1184 w1197 w1241 w1271 w1275 w1302 w1312 w1328 w1333 w1337 w1366 w1391 w1406 w1430 w1460 w1465 w1472 w1487 w1505 w1530 w1541 w1559 w1576 w1601 w1620 w1633 w1641 w1660 w1672 w1684 w1703 w1719 w1732 w1744 w1756 w1760 w1765 w1772 w1784 w1793 w1799 w1806 w1816 w1824 w1840 w1868 w1874 w1903 w1913 w1935 w1939 w1943 w1951 w1960 w1969 w1975 w1983 w1990 w2000 w2028 w2036 w2043 w2051 w2056 w2062 w2072 w2077 w2082 w2098 w2103 w2111 w2121 w2192 w2197 w2210 w2231 w2240 w2255 w2279 w2290 w2300 w2324 w2351 w2357 w2369 w2394 w2403 w2409 w2414 w2421 w2428 w2442 w2452 w2457 w2467 w2476 w2481 w2486 w2496 w2519 w2538 w2542 w2554 w2575 w2597 w2616 w2620 w2628 w2662 w2667 w2673 w2683 w2699 w2706 w2742 w2769 w2782 w2786 w2802 w2826 w2831]
      tunnel: [w99 w372 w380 w399 w408 w414 w420 w443 w458 w500 w531 w549 w572 w610 w628 w634 w659 w683 w708 w731 w793 w826 w866 w889 w896 w906 w928 errorcluster {"status"=FALSE, "code"=0, "source"=""} ("error out") w959 w965 w978 w997 w1011 w1034 w1091 w1096 w1102 w1109 w1136 w1162 w1185 w1188 w1233 w1265 w1279 w1303 w1313 w1319 w1334 w1340 w1364 w1387 w1405 w1418 w1454 w1466 w1477 w1481 w1496 w1525 w1537 w1555 w1575 w1592 w1621 w1625 w1643 w1658 w1670 w1682 w1705 w1720 w1733 w1736 w1753 w1761 w1769 w1777 w1781 w1790 w1800 w1803 w1812 w1827 w1848 w1867 w1878 w1896 w1917 w1933 w1940 w1948 w1956 w1961 w1968 w1976 w1984 w1991 w2001 w2029 w2037 w2044 w2052 w2057 w2065 w2071 w2078 w2084 w2099 w2104 w2109 w2122 w2193 w2201 w2213 w2223 w2236 w2256 w2280 w2289 w2302 w2326 w2352 w2358 w2366 w2388 w2404 w2410 w2415 w2422 w2432 w2444 w2453 w2458 w2472 w2477 w2482 w2487 w2497 w2509 w2531 w2543 w2547 w2561 w2587 w2608 w2621 w2627 w2655 w2669 w2676 w2684 w2690 w2708 w2721 w2748 w2778 w2787 w2790 w2820 w2832] -> w72
      tunnel: w73 -> [w98 w372 w380 w399 w408 w414 w420 w443 w458 w500 w531 w549 w570 w611 w628 w635 w668 w683 w698 w731 w793 w827 w869 w890 w896 w905 w928 w932 w959 w965 w978 w997 w1010 w1046 w1091 w1096 w1102 w1113 w1140 w1166 w1185 w1195 w1236 w1264 w1278 w1303 w1313 w1321 w1334 w1339 w1365 w1390 w1411 w1423 w1453 w1466 w1474 w1484 w1495 w1524 w1540 w1554 w1574 w1591 w1621 w1631 w1644 w1657 w1669 w1681 w1704 w1721 w1733 w1740 w1748 w1761 w1769 w1777 w1780 w1789 w1800 w1804 w1813 w1832 w1847 w1866 w1877 w1902 w1916 w1932 w1940 w1948 w1956 w1961 w1968 w1976 w1984 w1991 w2001 w2029 w2037 w2044 w2052 w2057 w2065 w2071 w2078 w2084 w2099 w2104 w2110 w2123 w2193 w2202 w2212 w2219 w2235 w2257 w2280 w2289 w2297 w2329 w2352 w2358 w2371 w2387 w2404 w2410 w2415 w2422 w2432 w2444 w2453 w2458 w2472 w2477 w2482 w2487 w2497 w2508 w2530 w2543 w2546 w2560 w2592 w2613 w2621 w2630 w2658 w2668 w2677 w2684 w2689 w2707 w2720 w2751 w2777 w2787 w2799 w2819 w2832]
      tunnel: [w101 w373 w381 w400 w409 w415 w421 w444 w459 w501 w535 w550 w579 w617 w629 w653 w681 w693 w719 w732 w798 w836 w879 w892 w897 w903 w930 w938 w961 w966 w979 w998 w1026 w1054 w1092 w1097 w1103 w1129 w1155 w1181 w1186 w1203 w1250 w1273 w1289 w1304 w1314 w1330 w1335 w1347 w1376 w1400 w1412 w1450 w1461 w1467 w1478 w1490 w1521 w1534 w1548 w1563 w1582 w1617 w1622 w1636 w1646 w1662 w1674 w1686 w1714 w1729 w1734 w1745 w1757 w1762 w1770 w1778 w1787 w1796 w1801 w1809 w1818 w1836 w1852 w1872 w1883 w1905 w1919 w1936 w1941 w1949 w1957 w1962 w1970 w1977 w1985 w1992 w2002 w2030 w2038 w2045 w2053 w2058 w2066 w2073 w2079 w2086 w2100 w2105 w2112 w2124 w2194 w2206 w2215 w2232 w2241 w2264 w2281 w2292 w2305 w2330 w2353 w2359 w2375 w2397 w2405 w2411 w2416 w2423 w2433 w2445 w2454 w2459 w2473 w2478 w2483 w2488 w2498 w2520 w2539 w2544 w2555 w2576 w2598 w2617 w2622 w2652 w2664 w2671 w2680 w2685 w2703 w2718 w2746 w2774 w2783 w2788 w2811 w2828 w2833] -> w89
      tunnel: [_ _ _ _ _ _ _ _ _ _ _ _ _ _ _ _ _ _ _ _ _ _ _ _ _ _ _ _ TRUE _ _ _ _ _ _ _ _ _ _ _ _ _ _ _ _ _ _ _ _ _ _ _ _ _ _ _ _ _ _ _ _ _ _ _ _ _ _ _ _ _ _ _ _ _ _ _ _ _ _ _ _ _ _ _ _ _ _ _ _ _ _ _ _ _ _ _ _ _ _ _ _ _ _ _ _ _ _ _ _ _ _ _ _ _ _ _ _ _ _ _ _ _ _ _ _ _ _ _ _ _ _ _ _ _ _ _ _ _ _ _ _ _ _ _ _ _ _ _ _ _ _ _ _ _ _ _ _ _ _ _ _] -> w80
      tunnel: [w97 w371 w377 w391 w406 w413 w419 w442 w457 w475 w533 w541 w576 w614 w626 w646 w672 w691 w717 w730 w758 w830 w868 w888 w895 w902 w929 w936 w960 w964 w969 w990 w1020 w1048 w1090 w1095 w1101 w1108 w1135 w1161 w1184 w1197 w1242 w1271 w1276 w1302 w1312 w1329 w1333 w1338 w1366 w1391 w1410 w1430 w1460 w1465 w1475 w1487 w1505 w1530 w1541 w1559 w1576 w1601 w1620 w1634 w1641 w1660 w1672 w1684 w1703 w1719 w1732 w1744 w1756 w1760 w1766 w1773 w1785 w1794 w1799 w1807 w1817 w1825 w1846 w1855 w1879 w1904 w1914 w1935 w1939 w1944 w1952 w1960 w1969 w1975 w1983 w1990 w2000 w2028 w2036 w2043 w2051 w2056 w2062 w2072 w2077 w2082 w2098 w2103 w2111 w2121 w2192 w2198 w2211 w2231 w2240 w2255 w2279 w2290 w2301 w2325 w2351 w2357 w2370 w2394 w2403 w2409 w2414 w2421 w2429 w2442 w2452 w2457 w2467 w2476 w2481 w2486 w2496 w2519 w2538 w2542 w2554 w2575 w2597 w2616 w2620 w2629 w2662 w2667 w2674 w2683 w2699 w2706 w2742 w2769 w2782 w2786 w2802 w2826 w2831] -> w88
      tunnel: 30 ("Timeout") -> [w96 _ _ _ _ _ _ _ _ _ _ _ _ _ _ _ _ _ _ _ _ _ _ _ _ _ _ _ _ _ _ _ _ _ _ _ _ _ _ _ _ _ _ _ _ _ _ _ _ _ _ _ _ _ _ _ _ _ _ _ _ _ _ _ _ _ _ _ _ _ _ _ _ _ _ _ _ _ _ _ _ _ _ _ _ _ _ _ _ _ _ _ _ _ _ _ _ _ _ _ _ _ _ _ _ _ _ _ _ _ _ _ _ _ _ _ _ _ _ _ _ _ _ _ _ _ _ _ _ _ _ _ _ _ _ _ _ _ _ _ _ _ _ _ _ _ _ _ _ _ _ _ _ _ _ _ _ _ _ _ _]
      tunnel: w85 -> [_ _ _ _ _ _ _ _ _ _ _ _ _ _ _ _ _ _ _ _ _ w834 _ _ _ _ _ _ _ _ _ _ _ _ _ _ _ _ _ _ _ _ _ _ _ _ _ _ _ _ _ _ _ _ _ _ _ _ _ _ _ _ _ _ _ _ _ _ _ _ _ _ _ w1741 w1752 _ _ _ _ _ _ _ _ _ _ _ _ _ _ _ _ _ _ _ _ _ _ _ _ _ _ _ _ _ _ _ _ _ _ _ _ _ _ _ _ _ _ _ _ _ _ _ _ _ _ _ _ _ _ _ _ _ _ _ _ _ _ _ _ _ _ _ _ _ _ _ _ _ _ _ _ _ _ _ _ _ _ _ _ _ _]
      tunnel: w84 -> [_ _ _ _ _ _ _ _ _ _ _ _ _ _ _ _ _ _ _ _ _ w833 _ _ _ _ _ _ _ _ _ _ _ _ _ _ _ _ _ _ _ _ _ _ _ _ _ _ _ _ _ _ _ _ _ _ _ _ _ _ _ _ _ _ _ _ _ _ _ _ _ _ _ w1742 w1751 _ _ _ _ _ _ _ _ _ _ _ _ _ _ _ _ _ _ _ _ _ _ _ _ _ _ _ _ _ _ _ _ _ _ _ _ _ _ _ _ _ _ _ _ _ _ _ _ _ _ _ _ _ _ _ _ _ _ _ _ _ _ _ _ _ _ _ _ _ _ _ _ _ _ _ _ _ _ _ _ _ _ _ _ _ _]
      tunnel: w83 -> [w95 _ _ _ _ _ _ _ _ _ _ _ _ _ _ _ _ _ _ _ _ _ _ _ _ _ _ _ _ _ _ _ _ _ _ _ _ _ _ _ _ _ _ w1267 _ _ _ _ _ _ _ _ _ _ _ _ _ _ _ _ _ _ _ _ _ _ _ _ _ _ _ _ _ _ _ _ _ _ _ _ _ _ _ _ _ _ _ _ _ _ _ _ _ _ _ _ _ _ _ _ _ _ _ _ _ _ _ _ _ _ _ _ _ _ _ _ _ _ _ _ _ _ _ _ _ _ _ _ _ _ _ _ _ _ _ _ _ _ _ _ _ _ _ _ _ _ _ _ _ _ _ _ _ _ _ _ _ _ _ _ _]
      tunnel: w82 -> [w94 w370 w379 w398 w407 w412 w418 w434 w456 w485 w534 w548 w578 w616 w627 w652 w680 w692 w718 w729 w797 w835 w878 w887 w894 w899 w916 w935 w958 w963 w977 w996 w1025 w1045 w1088 w1094 w1100 w1107 w1134 w1160 w1183 w1192 w1216 w1272 w1288 w1301 w1311 w1316 w1332 w1346 w1375 w1399 w1404 w1449 w1452 w1464 w1471 w1480 w1492 w1523 w1539 w1553 w1573 w1588 w1619 w1635 w1645 w1661 w1673 w1685 w1713 w1716 w1731 w1743 w1750 w1759 w1768 w1776 w1783 w1792 w1798 w1808 w1811 w1823 w1841 w1856 w1875 w1901 w1918 w1934 w1938 w1946 w1954 w1959 w1967 w1974 w1982 w1989 w1999 w2027 w2035 w2042 w2047 w2055 w2064 w2070 w2076 w2083 w2093 w2102 w2107 w2118 w2191 w2196 w2208 w2218 w2234 w2263 w2278 w2291 w2303 w2327 w2347 w2355 w2368 w2396 w2401 w2407 w2413 w2420 w2431 w2443 w2451 w2456 w2471 w2475 w2480 w2485 w2495 w2518 w2537 w2541 w2553 w2574 w2596 w2615 w2619 w2651 w2663 w2670 w2679 w2682 w2702 w2717 w2745 w2773 w2781 w2785 w2810 w2827 w2830]
      tunnel: [w93 w370 w379 w398 w407 w412 w418 w434 w456 w485 w534 w548 w578 w616 w627 w652 w680 w692 w718 w729 w797 w835 w878 w887 w894 w899 w916 w935 w958 w963 w977 w996 w1025 w1045 w1088 w1094 w1100 w1107 w1134 w1160 w1183 w1192 w1216 w1272 w1288 w1301 w1311 w1316 w1332 w1346 w1375 w1399 w1404 w1449 w1452 w1464 w1471 w1480 w1492 w1523 w1539 w1553 w1573 w1588 w1619 w1635 w1645 w1661 w1673 w1685 w1713 w1716 w1731 w1743 w1750 w1759 w1768 w1776 w1783 w1792 w1798 w1808 w1811 w1823 w1841 w1856 w1875 w1901 w1918 w1934 w1938 w1946 w1954 w1959 w1967 w1974 w1982 w1989 w1999 w2027 w2035 w2042 w2047 w2055 w2064 w2070 w2076 w2083 w2093 w2102 w2107 w2118 w2191 w2196 w2208 w2218 w2234 w2263 w2278 w2291 w2303 w2327 w2347 w2355 w2368 w2396 w2401 w2407 w2413 w2420 w2431 w2443 w2451 w2456 w2471 w2475 w2480 w2485 w2495 w2518 w2537 w2541 w2553 w2574 w2596 w2615 w2619 w2651 w2663 w2670 w2679 w2682 w2702 w2717 w2745 w2773 w2781 w2785 w2810 w2827 w2830] -> w81
      tunnel: w77 -> [_ _ _ _ _ _ _ _ _ _ _ _ _ _ _ _ _ _ _ _ _ w828 _ _ _ _ _ _ _ _ _ _ _ _ _ _ _ _ _ _ _ _ _ _ _ _ _ _ _ _ _ _ _ _ _ _ _ _ _ _ _ _ _ _ _ _ _ _ _ _ _ _ _ w1738 w1749 _ _ _ _ _ _ _ _ _ _ _ _ _ _ _ _ _ _ _ _ _ _ _ _ _ _ _ _ _ _ _ _ _ _ _ _ _ _ _ _ _ _ _ _ _ _ _ _ _ _ _ _ _ _ _ _ _ _ _ _ _ _ _ _ _ _ _ _ _ _ _ _ _ _ _ _ _ _ _ _ _ _ _ _ _ _]
      tunnel: w71 -> [_ _ _ _ _ _ _ _ _ _ _ _ _ _ _ _ _ _ _ _ _ _ _ _ _ _ _ _ _ _ _ _ _ _ _ _ _ _ _ _ _ _ _ _ _ _ _ _ _ _ _ _ _ _ _ _ _ _ _ _ _ _ _ _ _ _ _ _ _ _ _ _ _ _ _ _ _ _ _ _ _ _ _ _ _ _ _ _ _ _ _ _ _ _ _ _ _ _ _ _ _ _ _ _ _ _ _ _ _ _ _ _ _ _ _ _ _ _ _ _ _ _ _ _ _ _ _ _ _ _ _ _ _ _ _ _ _ _ _ _ _ _ _ _ _ _ _ _ w2660 _ _ _ _ _ _ _ _ _ _ _ _]
      tunnel: w70 -> [_ _ _ _ _ _ _ _ _ _ _ _ _ _ _ _ _ _ _ _ _ _ _ _ _ _ _ _ _ _ _ _ _ _ _ _ _ _ _ _ _ _ _ _ _ _ _ _ _ _ _ _ _ _ _ _ _ _ _ _ _ _ _ _ _ _ _ _ _ _ _ _ _ _ _ _ _ _ _ _ _ _ _ _ _ _ _ _ _ _ _ _ _ _ _ _ _ _ _ _ _ _ _ _ _ _ _ _ _ _ _ _ _ _ _ _ _ _ _ _ _ _ _ _ _ _ _ _ _ _ _ _ _ _ _ _ _ _ _ _ _ _ _ _ _ _ _ _ _ _ _ _ _ _ _ _ w2780 _ _ _ _]
      frame "", "Event Structure", "Idle" {
        # "executes when the state queue is empty"
        n34 = event shown="[0] Timeout" {
          selector: w94 -> [_ _ _ _ _ _ _ _ _ _ _ _ _ _ _ _ _ _ _ _ _ _ _ _ _ _ _ _ _]
          dyn-events: [_ _ _ _ _ _ _ _ _ _ _ _ _ _ _ _ _ _ _ _ _ _ _ _ _ _ _ _ _] -> w93
          timeout: w96 -> [_ _ _ _ _ _ _ _ _ _ _ _ _ _ _ _ _ _ _ _ _ _ _ _ _ _ _ _ _]
          tunnel: w102 -> [w120 w131 w139 w143 w147 w155 w162 w186 w202 w218 w222 w229 w251 w265 w279 w284 w287 w293 w298 w303 w308 w313 w318 w323 w335 w342 w346 w358 w369]
          tunnel: [w121 w131 w138 w143 w146 w155 w161 w186 w202 w218 w222 w228 w251 w265 w279 w283 w286 w293 w299 w303 w309 w314 w319 w323 w336 w342 w346 w359 w368] -> w101
          tunnel: w100 -> [w105 w129 w133 w141 w148 w153 w157 w184 w200 w216 w220 w224 w250 w264 w278 w280 w288 w291 w295 w301 w305 w311 w316 w321 w331 w340 w344 w356 w366]
          tunnel: [w119 w130 w134 w142 w149 w154 w163 w185 w201 w217 w221 w230 w248 w253 w275 w282 w289 w292 w297 w302 w307 w312 w317 w322 w332 w341 w345 w360 w367] -> w99
          tunnel: w98 -> [w119 w130 w134 w142 w149 w154 w163 w185 w201 w217 w221 w230 w246 w254 w267 w282 w289 w292 w297 w302 w307 w312 w317 w322 w334 w341 w345 w360 w367]
          tunnel: [w105 w129 w133 w141 w148 w153 w158 w184 w200 w216 w220 w225 w250 w264 w278 w280 w288 w291 w295 w301 w305 w311 w316 w321 w337 w340 w344 w357 w366] -> w97
          tunnel: w95 -> [_ _ _ _ _ _ _ _ _ _ _ _ _ _ _ _ _ _ _ _ _ _ _ _ _ _ _ _ _]
          event Timeout {
            # "check system status every 2s"
            n35 = event-data() -> ()  [unwired: 1 in, 1 out]
            n36 = Unbundle By Name(w105) -> ("SysRunning?"=w103:bool, "SlowTimer"=w118:u32, "FastTimer"=w112:u32)
            n37 = Tick Count (ms)() -> (millisecond timer value=w106:u32)
            n38 = Subtract(x=w106, y=w118) -> (x-y=w115:u32)
            n39 = case shown="True" w103 {
              tunnel: ["" "/*Utility: AquiTimerCheck" ("State(s) in Front (\"\")")] -> w110
              frame False {
                # "if not running, do nothing"
              }
              frame True {
                # "if aquisition is running, check timer"
              }
            }
            n40 = Subtract(x=w106, y=w112) -> (x-y=w113:u32)
            n41 = Greater?(x=w115, y=u32 2000) -> (0:w116:bool)
            n42 = Greater?(x=w113, y=u32 500) -> (0:w104:bool)
            n43 = case shown="True" w116 {
              tunnel: ["" ("Empty String Constant") "SystemStatus: SlowSysStatusMacro" ("State(s) in Front (\"\")")] -> w109
              frame False {
              }
              frame True {
              }
            }
            n44 = case shown="True" w104 {
              tunnel: ["" ("Empty String Constant") "SystemStatus: FastSysStatusMacro" ("State(s) in Front (\"\")")] -> w107
              frame False {
              }
              frame True {
              }
            }
            n45 = call <vilib>:"Add State(s) to Queue__JKI_lib_State_Machine.vi"("State(s) in Front (\"\")"=w110, "State(s) at Back (\"\")"=w109) -> ("States Out"=w108:string)  [unwired: 13 in]
            n46 = call <vilib>:"Add State(s) to Queue__JKI_lib_State_Machine.vi"("State(s) in Front (\"\")"=w108, "State(s) in (\"\")"=w107) -> ("States Out"=w111:string)  [unwired: 13 in]
            n47 = call <vilib>:"Add State(s) to Queue__JKI_lib_State_Machine.vi"("State(s) in Front (\"\")"=w111, "State(s) in (\"\")"=w120) -> ("States Out"=w121:string)  [unwired: 13 in]
          }
          event "355nm Laser toggle": Mouse Enter {
            n48 = event-data() -> ()  [unwired: 1 in, 4 out]
            n49 = local write "Help"("Toggle 355nm laser." ("Help")) -> ()
          }
          event "355nm Laser toggle": Value Change {
            # "[Covers: REQ34]"
            n50 = event-data() -> ()  [unwired: 1 in, 6 out]
            n51 = Select(t="LabJack: 355_PWM_Start\nLabJack: AB_Start", s="355nm Laser toggle", f="LabJack: 355_PWM_Stop\nLabJack: AB_Stop") -> (s? t:f=w136:string)
            n52 = call <vilib>:"Add State(s) to Queue__JKI_lib_State_Machine.vi"("State(s) in Front (\"\")"=w136, "State(s) in (\"\")"=w139) -> ("States Out"=w138:string)  [unwired: 13 in]
          }
          event "Aiming beam toggle": Mouse Enter {
            n53 = event-data() -> ()  [unwired: 1 in, 4 out]
            n54 = local write "Help"("Toggle aiming beam laser." ("Help")) -> ()
          }
          event "Aiming beam toggle": Value Change {
            # "[Covers: REQ33]"
            n55 = event-data() -> ()  [unwired: 1 in, 6 out]
            n56 = case shown="False" "Aiming beam toggle" {
              tunnel: ["LabJack: AB_Stop" ("State(s) in Front (\"\")") "LabJack: AB_Start" ("State(s) in Front (\"\")")] -> w145
              frame False {
              }
              frame True {
              }
            }
            n57 = call <vilib>:"Add State(s) to Queue__JKI_lib_State_Machine.vi"("State(s) in Front (\"\")"=w145, "State(s) in (\"\")"=w147) -> ("States Out"=w146:string)  [unwired: 13 in]
          }
          event "Background": Mouse Enter {
            n58 = event-data() -> ()  [unwired: 1 in, 4 out]
            n59 = local write "Help"("Click to record a background." ("Help")) -> ()
          }
          event "Background": Value Change {
            n60 = event-data() -> ("NewVal"=w159:bool)  [unwired: 1 in, 5 out]
            n61 = case shown="False" w159 {
              tunnel: ["Queue: Flash\nUtility: Dewelling >> 100\nLabJack: 355_PWM_Stop\n/*LabJack: AB_Stop" "Utility: SetDataClass >> Bg\nUI: Update\nLabJack: 355_PWM_Start\n/*LabJack: AB_Start\nUtility: Dewelling >> 50\nLabJack: SetV\nDigitizer: Start\nUtility: AquiTimerReset\nLED: BreathGreen\nUI: duringBGAcquire"] -> w160
              tunnel: [FALSE TRUE] -> w156
              frame False {
                n62 = property on="Background" class="Bool (strict)"("BoolText.Text"="Done!" ("Boolean Text.Text")) -> ()  [unwired: 2 in, 2 out]
              }
              frame True {
                # "[Covers: REQ6]"
                n63 = property on="Background" class="Bool (strict)"("BoolText.Text"="Running" ("Boolean Text.Text"), "Colors [4]"=cluster{u32, u32}[] [{6618880, 6618880}, {16711680, 16711680}]) -> ()  [unwired: 2 in, 2 out]
              }
            }
            n64 = Bundle By Name(cluster=w157, "SysRunning?"=w156) -> (w158:T19)
            n65 = call <vilib>:"Add State(s) to Queue__JKI_lib_State_Machine.vi"("State(s) in Front (\"\")"=w160, "State(s) in (\"\")"=w162) -> ("States Out"=w161:string)  [unwired: 13 in]
          }
          event "Channel 1": Cursor Move {
            n66 = event-data() -> ("CursIdx"=w175:i32, "CursLoc"=w182:cluster{"X":dbl, "Y":dbl})  [unwired: 1 in, 7 out]
            n67 = Unbundle By Name(w182) -> ("X"=w180:dbl)
            n68 = property on="Channel 2" class="WFGraph (strict)"() -> ("CrsrList"=w179:T20)  [unwired: 2 in, 2 out]
            n69 = property on="Channel 3" class="WFGraph (strict)"() -> ("CrsrList"=w176:T20)  [unwired: 2 in, 2 out]
            n70 = Index Array(array=w179, index=w175) -> (element=w183:T21)
            n71 = Index Array(array=w176, index=w175) -> (element=w181:T21)
            n72 = Bundle By Name(cluster=w181, "Position.X"=w180) -> (w174:T21)
            n73 = Bundle By Name(cluster=w183, "Position.X"=w180) -> (w178:T21)
            n74 = control-ref of="Channel 1"() -> (w171:refnum<vi>)
            n75 = Replace Array Subset(array=w179, new element=w178, index=w175) -> (w177:T20)
            n76 = Replace Array Subset(array=w176, new element=w174, index=w175) -> (w173:T20)
            n77 = property on="Channel 2" class="WFGraph (strict)"("CrsrList"=w177) -> ()  [unwired: 2 in, 2 out]
            n78 = property on="Channel 3" class="WFGraph (strict)"("CrsrList"=w173) -> (error out=w172:errorcluster)  [unwired: 2 in, 1 out]
            n79 = call "UpdateCurserIdx(SubVI).vi"("error in (no error)"=w172, "WaveformGraph in"=w171) -> ()  [unwired: 9 in, 1 out]
          }
          event "Channel 2": Cursor Move {
            n80 = event-data() -> ("CursIdx"=w193:i32, "CursLoc"=w199:cluster{"X":dbl, "Y":dbl})  [unwired: 1 in, 7 out]
            n81 = Unbundle By Name(w199) -> ("X"=w196:dbl)
            n82 = property on="Channel 1" class="WFGraph (strict)"() -> ("CrsrList"=w191:T20)  [unwired: 2 in, 2 out]
            n83 = property on="Channel 3" class="WFGraph (strict)"() -> ("CrsrList"=w194:T20)  [unwired: 2 in, 2 out]
            n84 = Index Array(array=w191, index=w193) -> (element=w198:T21)
            n85 = Index Array(array=w194, index=w193) -> (element=w197:T21)
            n86 = Bundle By Name(cluster=w198, "Position.X"=w196) -> (w195:T21)
            n87 = Bundle By Name(cluster=w197, "Position.X"=w196) -> (w192:T21)
            n88 = Replace Array Subset(array=w191, new element=w195, index=w193) -> (w190:T20)
            n89 = Replace Array Subset(array=w194, new element=w192, index=w193) -> (w189:T20)
            n90 = control-ref of="Channel 1"() -> (w188:refnum<vi>)
            n91 = property on="Channel 1" class="WFGraph (strict)"("CrsrList"=w190) -> ()  [unwired: 2 in, 2 out]
            n92 = property on="Channel 3" class="WFGraph (strict)"("CrsrList"=w189) -> (error out=w187:errorcluster)  [unwired: 2 in, 1 out]
            n93 = call "UpdateCurserIdx(SubVI).vi"("error in (no error)"=w187, "WaveformGraph in"=w188) -> ()  [unwired: 9 in, 1 out]
          }
          event "Channel 3": Cursor Move {
            n94 = event-data() -> ("CursIdx"=w208:i32, "CursLoc"=w215:cluster{"X":dbl, "Y":dbl})  [unwired: 1 in, 7 out]
            n95 = Unbundle By Name(w215) -> ("X"=w212:dbl)
            n96 = property on="Channel 1" class="WFGraph (strict)"() -> ("CrsrList"=w211:T20)  [unwired: 2 in, 2 out]
            n97 = property on="Channel 2" class="WFGraph (strict)"() -> ("CrsrList"=w209:T20)  [unwired: 2 in, 2 out]
            n98 = Index Array(array=w211, index=w208) -> (element=w214:T21)
            n99 = Index Array(array=w209, index=w208) -> (element=w213:T21)
            n100 = Bundle By Name(cluster=w214, "Position.X"=w212) -> (w210:T21)
            n101 = Bundle By Name(cluster=w213, "Position.X"=w212) -> (w207:T21)
            n102 = Replace Array Subset(array=w211, new element=w210, index=w208) -> (w206:T20)
            n103 = Replace Array Subset(array=w209, new element=w207, index=w208) -> (w205:T20)
            n104 = control-ref of="Channel 1"() -> (w203:refnum<vi>)
            n105 = property on="Channel 1" class="WFGraph (strict)"("CrsrList"=w206) -> ()  [unwired: 2 in, 2 out]
            n106 = property on="Channel 2" class="WFGraph (strict)"("CrsrList"=w205) -> (error out=w204:errorcluster)  [unwired: 2 in, 1 out]
            n107 = call "UpdateCurserIdx(SubVI).vi"("error in (no error)"=w204, "WaveformGraph in"=w203) -> ()  [unwired: 9 in, 1 out]
          }
          event "Cali&iRF alignment": Mouse Enter {
            n108 = event-data() -> ()  [unwired: 1 in, 4 out]
            n109 = local write "Help"("Click to run system intensity calibration and irf alignment" ("Help")) -> ()
          }
          event "Cali&iRF alignment": Value Change {
            n110 = event-data() -> ("NewVal"=w226:bool)  [unwired: 1 in, 5 out]
            n111 = case shown="False" w226 {
              tunnel: ["Queue: Flash\nUtility: Dewelling >> 1000\nLabJack: 355_PWM_Stop\n/*LabJack: AB_Stop" "Utility: SetDataClass >> Cali\nUI: Update\nLabJack: 355_PWM_Start\n/*LabJack: AB_Start\nLabJack: SetV\nDigitizer: Start\nUtility: AquiTimerReset\nLED: BreathGreen\nUI: duringIRFAlign"] -> w227
              tunnel: [FALSE TRUE] -> w223
              frame False {
                n112 = property on="Cali&iRF alignment" class="Bool (strict)"("BoolText.Text"="Done!" ("Boolean Text.Text")) -> ()  [unwired: 2 in, 2 out]
              }
              frame True {
                n113 = property on="Cali&iRF alignment" class="Bool (strict)"("BoolText.Text"="Running" ("Boolean Text.Text"), "Colors [4]"=cluster{u32, u32}[] [{6618880, 6618880}, {16711680, 16711680}]) -> ()  [unwired: 2 in, 2 out]
              }
            }
            n114 = Bundle By Name(cluster=w224, "SysRunning?"=w223) -> (w225:T19)
            n115 = call <vilib>:"Add State(s) to Queue__JKI_lib_State_Machine.vi"("State(s) in Front (\"\")"=w227, "State(s) in (\"\")"=w229) -> ("States Out"=w228:string)  [unwired: 13 in]
          }
          event "V 1": Value Change {
            n116 = event-data() -> ()  [unwired: 1 in, 6 out]
            n117 = call "LabJack_FGV.vi"("Operation(Read)"=enum16{"Write", "Read"}."Read" ("Operation"), "error in (no error)"=w246) -> ("error out"=w243:errorcluster, "Read data"=w244:i32)  [unwired: 8 in]
            n118 = global read "GlobalVariables.vi" "Ch1 LJ pin"() -> (w242:string)
            n119 = call "LJM_eWriteName.vi"("Handle In"=w244, "Name"=w242, "Value"="V 1", "error in"=w243) -> ("error out"=w240:errorcluster)  [unwired: 10 in, 1 out]
            n120 = call "V1FGV.vi"("Error In"=w240, "action (write)"=enum16{"write", "read"}."write" ("action"), "V1 in"="V 1") -> ("Error Out"=w239:errorcluster)  [unwired: 7 in, 1 out]
            n121 = call "CtrlVtoGain.vi"("error in (no error)"=w239, "CtrlV(V)"="V 1", "Channel"=enum16{"Ch1", "Ch2", "Ch3"}."Ch1" ("Enum")) -> ("error out"=w248:errorcluster, "Gain"=→"Gain1":dbl)  [unwired: 7 in]
          }
          event "V 2": Value Change {
            n122 = event-data() -> ()  [unwired: 1 in, 6 out]
            n123 = call "LabJack_FGV.vi"("Operation(Read)"=enum16{"Write", "Read"}."Read" ("Operation"), "error in (no error)"=w254) -> ("error out"=w259:errorcluster, "Read data"=w260:i32)  [unwired: 8 in]
            n124 = global read "GlobalVariables.vi" "Ch2 LJ pin"() -> (w258:string)
            n125 = call "LJM_eWriteName.vi"("Handle In"=w260, "Name"=w258, "Value"="V 2", "error in"=w259) -> ("error out"=w257:errorcluster)  [unwired: 10 in, 1 out]
            n126 = call "V2FGV.vi"("Error In"=w257, "action(write)"=enum16{"write", "read"}."write" ("action"), "V2 in"="V 2") -> ("Error Out"=w256:errorcluster)  [unwired: 7 in, 1 out]
            n127 = call "CtrlVtoGain.vi"("error in (no error)"=w256, "CtrlV(V)"="V 2", "Channel"=enum16{"Ch1", "Ch2", "Ch3"}."Ch2" ("Enum")) -> ("error out"=w253:errorcluster, "Gain"=→"Gain2":dbl)  [unwired: 7 in]
          }
          event "V 3": Value Change {
            n128 = event-data() -> ()  [unwired: 1 in, 6 out]
            n129 = call "LabJack_FGV.vi"("Operation(Read)"=enum16{"Write", "Read"}."Read" ("Operation"), "error in (no error)"=w267) -> ("error out"=w272:errorcluster, "Read data"=w273:i32)  [unwired: 8 in]
            n130 = global read "GlobalVariables.vi" "Ch3 LJ pin"() -> (w271:string)
            n131 = call "LJM_eWriteName.vi"("Handle In"=w273, "Name"=w271, "Value"="V 3", "error in"=w272) -> ("error out"=w269:errorcluster)  [unwired: 10 in, 1 out]
            n132 = call "V3FGV.vi"("Error In"=w269, "action(write)"=enum16{"write", "read"}."write" ("action"), "V3 in"="V 3") -> ("Error Out"=w268:errorcluster)  [unwired: 7 in, 1 out]
            n133 = call "CtrlVtoGain.vi"("error in (no error)"=w268, "CtrlV(V)"="V 3", "Channel"=enum16{"Ch1", "Ch2", "Ch3"}."Ch3" ("Enum")) -> ("error out"=w275:errorcluster, "Gain"=→"Gain3":dbl)  [unwired: 7 in]
          }
          event "Quit": Value Change {
            # "Exit Button Value Change (pressed) Event\n(when pressed.  quite)"
            n134 = event-data() -> ()  [unwired: 1 in, 1 out]
            n135 = call <vilib>:"Add State(s) to Queue__JKI_lib_State_Machine.vi"("State(s) in Front (\"\")"="LED: Off\nMacro: Exit", "State(s) in (\"\")"=w284) -> ("States Out"=w283:string)  [unwired: 13 in]
          }
          event "Show BG": Value Change {
            n136 = event-data() -> ()  [unwired: 1 in, 6 out]
            n137 = call <vilib>:"Add State(s) to Queue__JKI_lib_State_Machine.vi"("State(s) in Front (\"\")"="Data: showBG" ("State(s) in Front (\"\")"), "State(s) in (\"\")"=w287) -> ("States Out"=w286:string)  [unwired: 13 in]
          }
          event "StartButton": Mouse Enter {
            n138 = event-data() -> ()  [unwired: 1 in, 4 out]
            n139 = local write "Help"("Press to start aquisition." ("Help")) -> ()
          }
          event "StartButton": Value Change {
            n140 = event-data() -> ()  [unwired: 1 in, 6 out]
            n141 = local write "StartButton"(FALSE ("StartButton")) -> ()
            n142 = call <vilib>:"Add State(s) to Queue__JKI_lib_State_Machine.vi"("State(s) in Front (\"\")"="Macro: startAquisition", "State(s) in (\"\")"=w298) -> ("States Out"=w299:string)  [unwired: 13 in]
          }
          event "StopButton": Mouse Enter {
            n143 = event-data() -> ()  [unwired: 1 in, 4 out]
            n144 = local write "Help"("Press to stop data aquisition." ("Help")) -> ()
          }
          event "StopButton": Value Change {
            n145 = event-data() -> ()  [unwired: 1 in, 6 out]
            n146 = local write "StopButton"(FALSE ("StopButton")) -> ()
            n147 = call <vilib>:"Add State(s) to Queue__JKI_lib_State_Machine.vi"("State(s) in Front (\"\")"="Macro: stopAquisition" ("State(s) in Front (\"\")"), "State(s) in (\"\")"=w308) -> ("States Out"=w309:string)  [unwired: 13 in]
          }
          event User Event {
            n148 = event-data() -> ()  [unwired: 1 in, 5 out]
            n149 = call <vilib>:"Add State(s) to Queue__JKI_lib_State_Machine.vi"("State(s) in Front (\"\")"="Macro: startAquisition" ("State(s) in Front (\"\")"), "State(s) in (\"\")"=w313) -> ("States Out"=w314:string)  [unwired: 13 in]
          }
          event User Event {
            n150 = event-data() -> ()  [unwired: 1 in, 5 out]
            n151 = call <vilib>:"Add State(s) to Queue__JKI_lib_State_Machine.vi"("State(s) in Front (\"\")"="Macro: stopAquisition" ("State(s) in Front (\"\")"), "State(s) in (\"\")"=w318) -> ("States Out"=w319:string)  [unwired: 13 in]
          }
          event "Sys Reconfig": Mouse Enter {
            n152 = event-data() -> ()  [unwired: 1 in, 4 out]
            n153 = local write "Help"("Click to reconfig digitizer settings." ("Help")) -> ()
          }
          event "Sys Reconfig": Value Change {
            # "everytime the user change data aquisition setting, need to reinitilize decon engine and realign iRF.\ncheck whether data length has changed, if changed, reinitialize Decon engine\nreset BG ready, need a new BG"
            # "update DAQ FGV"
            n154 = event-data() -> ()  [unwired: 1 in, 6 out]
            n155 = call "SystemConfigEditorV6.vi"("error in"=w334) -> ("error out"=w333:errorcluster, "FLImDAQ out"=w328:T6)  [unwired: 1 in]
            n156 = Unbundle By Name(w331) -> ("FLImDAQ.min record length"=w330:i32)
            n157 = Unbundle By Name(w328) -> ("min record length"=w329:i32)
            n158 = call "FLImDAQ_FGV.vi"("error in (no error)"=w333, "Operation (Read)"=enum16{"Write", "Read"}."Write" ("Operation"), "Write data"=w328) -> ("error out"=w332:errorcluster, "Read data"=w327:T6)  [unwired: 7 in]
            n159 = Equal?(x=w330, y=w329) -> (x = y?=w326:bool)
            n160 = case shown="False" w326 {
              tunnel: ["UI: Cursor Set >> Busy\nDigitizer: Config\nUI: CaliAndiRFNotReady\n/*UI iRF not ready\nUI: Update\nUI: Cursor Set >> Idle" "UI: Cursor Set >> Busy\nDigitizer: Config\nUI: Update\nUI: Cursor Set >> Idle"] -> w325
              frame False {
              }
              frame True {
              }
            }
            n161 = Bundle By Name(cluster=w331, "FLImDAQ"=w327) -> (w337:T19)
            n162 = call <vilib>:"Add State(s) to Queue__JKI_lib_State_Machine.vi"("State(s) in Front (\"\")"=w325, "State(s) in (\"\")"=w335) -> ("States Out"=w336:string)  [unwired: 13 in]
          }
          event "System Hardware Connection Status", "StartButton", "StopButton", "355nm Laser toggle", "Aiming beam toggle", "Cali&iRF alignment", "Background", "Sys Reconfig": Mouse Leave {
            n163 = event-data() -> ()  [unwired: 1 in, 4 out]
            n164 = invoke on="Help" class="Str" method="Reinit To Default"() -> ()  [unwired: 3 in, 3 out]
          }
          event "System Hardware Connection Status.Digitizer": Mouse Enter {
            n165 = event-data() -> ()  [unwired: 1 in, 4 out]
            n166 = local write "Help"("Status of hardware connections. TCP/IP is optional." ("Help")) -> ()
          }
          event User Event {
            # "if aquisition loop is error out. Stop digitizer, update front panel indicator, stop both laser and \nOption 1: parse and save data\nOption 2: Flash queue if scout run. [Covers: REQ23]"
            n167 = event-data() -> ()  [unwired: 1 in, 5 out]
            n168 = case shown="\"Data\", Default" "Data Class" {
              tunnel: ["UI: Cursor Set >> Busy\n/*Data: parseRunData\n/*Data: saveRunData\nRun: Increment\nUI: Update\nUI: Cursor Set>>Idle" ("State(s) in Front (\"\")") "UI: Cursor Set >> Busy\nUI: Cursor Set >> Idle\nData: parseRunData\nData: irfAlignment" "UI: Cursor Set >> Busy\nUI: Cursor Set >> Idle\nData: parseRunData\nData: saveBGtoFGV\nData: saveBGtoFile\nData: showBG\nRun: BGIncrement"] -> w354
              frame "Data", Default {
              }
              frame "Cali" {
              }
              frame "BG" {
              }
            }
            n169 = Bundle By Name(cluster=w356, "SysRunning?"=FALSE) -> (w357:T19)
            n170 = Select(t="" ("State(s) in Front (\"\")"), s="Skip Data Save?", f=w354) -> (s? t:f=w351:string)
            n171 = call <vilib>:"Add State(s) to Queue__JKI_lib_State_Machine.vi"("State(s) in Front (\"\")"="UI: Update\n/*LabJack: AB_Stop\nLabJack: 355_PWM_Stop\nDigitizer: Abort\nEncoderDAQ: Abort\nLabJack: ZeroV\nUtility: EndBeep\nLED: BreathOff" ("State(s) in Front (\"\")"), "State(s) in (\"\")"=w351, "State(s) at Back (\"\")"="Macro: SysReadyForAq\nUI: Update" ("State(s) in Front (\"\")")) -> ("States Out"=w349:string)  [unwired: 12 in]
            n172 = call <vilib>:"Add State(s) to Queue__JKI_lib_State_Machine.vi"("State(s) in Front (\"\")"=w349, "State(s) in (\"\")"=w358) -> ("States Out"=w359:string)  [unwired: 13 in]
          }
          event Panel Close? {
            # "Discard the event because we'll close the front panel ourselves in Macro: Exit"
            # "Close Panel button (pressed) Event\n(this executes Macro: Exit to terminate the VI)"
            n173 = event-data() -> ()  [unwired: 1 in, 1 out]
            n174 = event-data ("Event Filter Node")("Discard?"=TRUE) -> ()  [unwired: 1 in, 1 out]
            n175 = call <vilib>:"Add State(s) to Queue__JKI_lib_State_Machine.vi"("State(s) in Front (\"\")"="Macro: Exit", "State(s) in (\"\")"=w369) -> ("States Out"=w368:string)  [unwired: 13 in]
          }
        }
      }
      frame "---------- Macro ----------" {
        # "Do not put any code in this frame.\n(It is a separator no-op. You can make a copy of this frame to create a new Macro frame)"
        n176 = call <vilib>:"Add State(s) to Queue__JKI_lib_State_Machine.vi"("State(s) in (\"\")"=w374) -> ("States Out"=w373:string)  [unwired: 14 in]
      }
      frame "Macro: stopAquisition" {
        # "if system is running, send stop command, if not do nothing."
        # "stop aquisition\nupdate UI"
        # "Stop Aquisition Macro, used by both local and remote start.\n(It is a separator no-op. You can make a copy of this frame to create a new Macro frame)"
        n177 = Unbundle By Name(w376) -> ("SysRunning?"=w378:bool)
        n178 = case shown="True" w378 {
          tunnel: ["" ("Empty String Constant") "LabJack: 355_PWM_Stop"] -> w375
          tunnel: w376 -> [w383 w387]
          tunnel: [w383 w386] -> w377
          frame False {
          }
          frame True {
            n179 = Bundle By Name(cluster=w387, "SysRunning?"=FALSE) -> (w386:T19)
          }
        }
        n180 = call <vilib>:"Add State(s) to Queue__JKI_lib_State_Machine.vi"("State(s) in Front (\"\")"=w375, "State(s) in (\"\")"=w382) -> ("States Out"=w381:string)  [unwired: 13 in]
      }
      frame "Macro: startAquisition" {
        # "start PWM before acquisition"
        # "Initialize both digitizer aquisition and\n send user event to trigger aquisition loop"
        # "[Covers: REQ32]"
        # "Start Aquisition Macro, used by both local and remote start.\n(It is a separator no-op. You can make a copy of this frame to create a new Macro frame)"
        n181 = local read "Skip Data Save?"() -> (w396:bool)
        n182 = Select(t="", s=w396, f="TDMS: OpenFile\nTDMS: Config\nTDMS: SaveMetaData\nTDMS: saveCtrlV\nEncoderFile: Open\nEncoderFile: SaveMetaData\nTDMS: StartStreaming") -> (s? t:f=w393:string)
        n183 = Bundle By Name(cluster=w390, "SysRunning?"=TRUE) -> (w391:T19)
        n184 = call <vilib>:"Add State(s) to Queue__JKI_lib_State_Machine.vi"("State(s) in Front (\"\")"=w393, "State(s) in (\"\")"="Utility: SetDataClass >> Data\nQueue: Flash\nUI: Update\nUtility: StartBeep\nDigitizer: ClearError\nEncoderDAQ: Start\n/*LabJack: AB_Start\nLabJack: SetV\nDigitizer: Start\nLabJack: 355_PWM_Start\nUtility: AquiTimerReset\nUI: DuringAquisition\nLED: BreathGreen") -> ("States Out"=w389:string)  [unwired: 13 in]
        n185 = call <vilib>:"Add State(s) to Queue__JKI_lib_State_Machine.vi"("State(s) in Front (\"\")"=w389, "State(s) in (\"\")"=w401) -> ("States Out"=w400:string)  [unwired: 13 in]
      }
      frame "Macro: Initialize" {
        # "load Labjack setting 1st as it contaisn laser pin infortmation"
        # "start laser 1st, need 7.5s for laser to get ready"
        # "Initialization Macro\n(This is called once, when the VI starts)"
        n186 = call <vilib>:"Add State(s) to Queue__JKI_lib_State_Machine.vi"("State(s) in Front (\"\")"="UI: showDisclaimer\nUI: Cursor Set >> Busy\nData: Initialize\nInitialize Core Data\nUI: Initialize\nUI: Front Panel State >> Open\nMacro: LoadSysConfig\nUI: Update\nLabJack: Open\nLabJack: SetDefaultSub\nLED: OpenVIRef\nLED: BreathOrange\nUI: Update\n355 Laser: CheckControllerStatus\n355 Laser: Laser enable\n355 Laser: Dewelling>>500\n355 Laser: CheckControllerStatus\nUI: Update\nLabJack: 355_PWM_Config\nLabJack: AB_PWM_Config\nUI: Update\n", "State(s) in (\"\")"="Digitizer: Initialize\nDigitizer: Config\nUI: Update\nEncoderDAQ: Initialize\nUI: Update\n/*AimingBeam: Initialize\n/*AimingBeam: Set Status>>Enable\n/*AimingBeam: Set Current\nUI: Update\n355 Laser: Check Dewelling\nUI: Cursor Set >> Idle\nCase: GetID\nUI: Update\nCase: CreatFileStruct\nUI: Update\nData: loadLastUseMacro\n/*DeconEngine: InitilizeMacro\nGraph: SetXMultiplier\nGraph: AddCursors\nAPD: Initialize\nAPD: LoadFromSerial\nAPD: UpdateCtrlVLimit\nAPD: GetGainLimits\nLED: BreathOff\nMacro: SysReadyForAq") -> ("States Out"=w402:string)  [unwired: 13 in]
        n187 = call <vilib>:"Add State(s) to Queue__JKI_lib_State_Machine.vi"("State(s) in Front (\"\")"=w402, "State(s) in (\"\")"=w410) -> ("States Out"=w409:string)  [unwired: 13 in]
        "Help" <- "Hover over controls to see help!" ("Help")
      }
      frame "Macro: LoadSysConfig" {
        # "System configuration Macro. [Covers: REQ15]\n(Load configurations for different component of the system)"
        n188 = call <vilib>:"Add State(s) to Queue__JKI_lib_State_Machine.vi"("State(s) in Front (\"\")"="SysConfig: Load Sys Config\nSysConfig: Load Digitizer Setting\nSysConfig: Load AB setting\nSysConfig: Load LJ Pinout\nSysConfig: Load 355 PWM\nSysConfig: LoadAPDSerialNumber\nSysConfig: LoadABVideoSetting\nSysConfig: LoadCursorLocation", "State(s) in (\"\")"=w416) -> ("States Out"=w415:string)  [unwired: 13 in]
      }
      frame "Macro: SysReadyForAq" {
        # "Macro for system ready\n(It is a separator no-op. You can make a copy of this frame to create a new Macro frame)"
        n189 = call <vilib>:"Add State(s) to Queue__JKI_lib_State_Machine.vi"("State(s) in Front (\"\")"="UI: ReadyForAquisition\nLED: Green" ("State(s) in Front (\"\")"), "State(s) in (\"\")"=w422) -> ("States Out"=w421:string)  [unwired: 13 in]
      }
      frame "Macro: Exit" {
        # "close LJ last"
        # "check whether hardware is initilized, if so close, if not do nothing"
        # "Exit Macro, close all hardware\n(This is called once, when the VI exits)"
        n190 = Unbundle By Name(w442) -> ("System Status.Encoder"=w423:bool, "System Status.Digitizer"=w438:bool, "System Status.Aiming Beam"=w437:bool, "System Status.355 Laser"=w436:bool, "System Status.Labjack"=w428:bool, "Core.Close Panel on Exit?"=w432:bool)
        n191 = case shown="True" w438 {
          tunnel: ["" ("Empty String Constant") "Digitizer: Close"] -> w433
          frame False {
          }
          frame True {
          }
        }
        n192 = case shown="True" w428 {
          tunnel: ["" ("Empty String Constant") "LabJack: SetDefaultAndClose"] -> w425
          frame False {
          }
          frame True {
          }
        }
        n193 = case shown="True" w437 {
          tunnel: ["" ("Empty String Constant") "AimingBeam: Set Status >> Disable\nAimingBeam: Close"] -> w427
          frame False {
          }
          frame True {
          }
        }
        n194 = case shown="True" w436 {
          tunnel: ["" ("Empty String Constant") "355 Laser: Close\n355 Laser: CheckControllerStatus"] -> w426
          frame False {
          }
          frame True {
          }
        }
        n195 = case shown="True" w423 {
          tunnel: ["" ("State(s) in Front (\"\")") "EncoderDAQ: Close" ("State(s) in Front (\"\")")] -> w424
          frame False {
          }
          frame True {
          }
        }
        n196 = Select(t="UI: Front Panel State >> Close", s=w432, f="" ("Empty String Constant")) -> (s? t:f=w429:string)
        n197 = call <vilib>:"Add State(s) to Queue__JKI_lib_State_Machine.vi"("State(s) in Front (\"\")"=w424, "State(s) in (\"\")"=w433, "State(s) at Back (\"\")"=w427) -> ("States Out"=w435:string)  [unwired: 12 in]
        n198 = call <vilib>:"Add State(s) to Queue__JKI_lib_State_Machine.vi"("State(s) in Front (\"\")"=w435, "State(s) in (\"\")"=w426, "State(s) at Back (\"\")"=w425) -> ("States Out"=w431:string)  [unwired: 12 in]
        n199 = call <vilib>:"Add State(s) to Queue__JKI_lib_State_Machine.vi"("State(s) in Front (\"\")"=w431, "State(s) in (\"\")"="UI: Update\nUI: Reset\nGraph: SaveCursorLoc\nLED: CloseVIRef\nQueue: Destory\nData: Cleanup\nExit", "State(s) at Back (\"\")"=w429) -> ("States Out"=w439:string)  [unwired: 12 in]
        n200 = call <vilib>:"Add State(s) to Queue__JKI_lib_State_Machine.vi"("State(s) in Front (\"\")"=w439, "State(s) in (\"\")"=w445) -> ("States Out"=w444:string)  [unwired: 13 in]
      }
      frame "---------- Data ----------" {
        # "Do not put any code in this frame.\n(It is a separator no-op. You can make a copy of this frame to create a new Data frame)"
        n201 = call <vilib>:"Add State(s) to Queue__JKI_lib_State_Machine.vi"("State(s) in (\"\")"=w460) -> ("States Out"=w459:string)  [unwired: 14 in]
      }
      frame "Data: Initialize" {
        w461 = "FLImData"  # TDMS group name
        w463 = FALSE  # bothVidSourceAvail
        w464 = T1 {"Main Frame Grabber"=FALSE, "Side Frame Grabber"=FALSE, "Main Camera"=FALSE, "Side Camera"=FALSE}  # video source
        w465 = FALSE  # LED vi ref open?
        w467 = path ""  # CaliPath
        w468 = T18 {"DeCon Channel"=enum."1", "Scale Bar"=FALSE, "Scale Low"=3.0, "Scale High"=8.0, "ANSI"=20.0, "Radius"=1.0, "3D?"=FALSE, "Firefly?"=FALSE, "Pentero?"=FALSE}  # VideoConfig
        w469 = T22 {"Ch1APDSerial#"="", "Ch2APDSerial#"="", "Ch3APDSerial#"=""}  # APDSerialNum
        w470 = u32 0  # Aquisition Timer
        w471 = cluster{"RunID":i8, "BG ID":i8, "Cali ID":i8} {"RunID"=1, "BG ID"=1, "Cali ID"=1}  # IDs
        w472 = refnum<vi> refnum  # LED vi reference
        w473 = path ""  # TempPath
        w474 = T23 {"DataPath"=path "", "BG Path"=path "", "iRFPath"=path "", "CaliPath"=path ""}  # Pathes
        w476 = dbl[] []  # V3
        w477 = dbl[] []  # V2
        w478 = dbl[] []  # V1
        w480 = u32 0  # FastTimer
        w481 = u32 0  # SlowTimer
        w482 = dbl[][] []  # Ch3Data
        w483 = dbl[][] []  # Ch2Data
        w466 = dbl[][] []  # Ch1Data
        w486 = T2 {"Digitizer"=FALSE, "Labjack"=FALSE, "Aiming Beam"=FALSE, "355 Laser"=FALSE, "Encoder"=FALSE}  # System Status
        w487 = T24 {"DIO_EF_CLOCK1_DIVISOR"=16, "DIO_EF_CLOCK1_ROLL_VALUE"=25000, "DIO#_EF_INDEX"=0, "DIO#_EF_OPTIONS"=1, "DIO#_EF_CONFIG_A"=6250}  # AB PWM setting
        w488 = T5 {"Ch1 Bias"="TDA11", "Ch2 Bias"="DAC10", "Ch3 Bias"="DAC0", "Ch4 Bias"="DAC0", "355 PWM"="FIO0", "AimingBeam PWM"="FIO2", "Laser Ready"="FIO3", "Interlock"="FIO1", "Laser Start/Stop"="FIO1", "Red LED"="FIO1", "Green LED"="FIO1", "Foot Pedal"="DIO15"}  # LJ Pinout
        w489 = 0  # TCP attempt count
        w490 = u32 0  # Laser start tic
        w491 = refnum<k20>[] []  # niTClk sessions
        w492 = u32 0  # Last Trigger
        w493 = T24 {"DIO_EF_CLOCK1_DIVISOR"=16, "DIO_EF_CLOCK1_ROLL_VALUE"=25000, "DIO#_EF_INDEX"=0, "DIO#_EF_OPTIONS"=1, "DIO#_EF_CONFIG_A"=6250}  # 355 PWM setting
        w494 = T25 {"Aiming Beam COM Port"="COM3", "Min Current"=0.0, "Max Current"=63.0, "Default Current"=20.0, "Freq"=0}  # AB Cluster
        w495 = T26 {"resource name"="", "resource name 2"="", "Channel"=enum."Channel 0", "trigger source"="VAL_EXTERNAL", "trigger level"=0.5, "trigger delay"=1.35e-07, "min sample rate"=12500000000.0, "min record length"=2500, "vertical range"=1.0, "vertical offset"=-0.25, "Waveform to Avg"=2000}  # FLImDAQ
        w496 = FALSE  # SysRunning?
        w484 = path ""  # DefaultPath
        w497 = ""  # CaseID
        w498 = T4 {"Ch1Enable?"=FALSE, "Ch2Enable?"=FALSE, "Ch3Enable?"=FALSE, "Ch1AutoGain?"=FALSE, "Ch2AutoGain?"=FALSE, "Ch3AutoGain?"=FALSE, "AimingBeamEnable?"=FALSE}  # SysConfigCluster
        w499 = T27 {"Current VI Reference"=refnum, "Close Panel on Exit?"=FALSE}  # Core
        # "Initialize the shift-register data, here.\n(data names are defined by what you wire into the bundle function)"
        n202 = Bundle("Core"=w499, "SysConfigCluster"=w498, "System Status"=w486, "IDs"=w471, "CaseID"=w497, "DefaultPath"=w484, "Pathes"=w474, "FLImDAQ"=w495, "SysRunning?"=w496, "AB Cluster"=w494, "LJ Pinout"=w488, "355 PWM setting"=w493, "AB PWM setting"=w487, "Last Trigger"=w492, "niTClk sessions"=w491, "Laser start tic"=w490, "TCP attempt count"=w489, "Ch1Data"=w466, "Ch2Data"=w483, "Ch3Data"=w482, "V1"=w478, "V2"=w477, "V3"=w476, "SlowTimer"=w481, "FastTimer"=w480, "listener ID"=refnum<k5> refnum, "TempPath"=w473, "LED vi reference"=w472, "Aquisition Timer"=w470, "APDSerialNum"=w469, "VideoConfig"=w468, "CaliPath"=w467, "LED vi ref open?"=w465, "video source"=w464, "bothVidSourceAvail"=w463, "EncoderDAQ"=refnum<k15> "PXI1Slot2", "TDMS group name"=w461) -> (w475:T19)  [unwired: 1 in]
        n203 = call <vilib>:"Add State(s) to Queue__JKI_lib_State_Machine.vi"("State(s) in (\"\")"=w502) -> ("States Out"=w501:string)  [unwired: 14 in]
      }
      frame "Data: LoadAPDData" {
        # "only load the last iRF for the moment"
        # "Load APD detector data\n(It is a separator no-op. You can make a copy of this frame to create a new Data frame)"
        n204 = Unbundle By Name(w533) -> ("APDSerialNum.Ch1APDSerial#"=w532:string, "APDSerialNum.Ch2APDSerial#"=w504:string, "APDSerialNum.Ch3APDSerial#"=w503:string)
        n205 = call "CreatFromSerialNumNoRaw.vi"("error in (no error)"=w531, "APD Serial #"=w532) -> ("error out"=w529:errorcluster, "APDClass out"=w530:refnum<class "APDClass.lvclass">)  [unwired: 8 in]
        n206 = call "CreatFromSerialNumNoRaw.vi"("error in (no error)"=w531, "APD Serial #"=w504) -> ("error out"=w518:errorcluster, "APDClass out"=w519:refnum<class "APDClass.lvclass">)  [unwired: 8 in]
        n207 = call "CreatFromSerialNumNoRaw.vi"("error in (no error)"=w531, "APD Serial #"=w503) -> ("error out"=w511:errorcluster, "APDClass out"=w512:refnum<class "APDClass.lvclass">)  [unwired: 8 in]
        n208 = call-dynamic "Read iRFData.vi"("error in (no error)"=w529, "APDClass in"=w530) -> ("iRFData"=w528:T28)  [unwired: 7 in, 2 out]
        n209 = call-dynamic "Read iRFData.vi"("error in (no error)"=w518, "APDClass in"=w519) -> ("iRFData"=w523:T28)  [unwired: 7 in, 2 out]
        n210 = call-dynamic "Read iRFData.vi"("error in (no error)"=w511, "APDClass in"=w512) -> ("iRFData"=w516:T28)  [unwired: 7 in, 2 out]
        n211 = Unbundle By Name(w528) -> ("iRFWFsAvg"=w527:dbl[][])
        n212 = Unbundle By Name(w523) -> ("iRFWFsAvg"=w522:dbl[][])
        n213 = Unbundle By Name(w516) -> ("iRFWFsAvg"=w515:dbl[][])
        n214 = Array Size(array=w527) -> (size(s)=w526:i32[])
        n215 = Array Size(array=w522) -> (size(s)=w517:i32[])
        n216 = Array Size(array=w515) -> (size(s)=w510:i32[])
        n217 = Index Array(array=w526, index=1) -> (element=w524:i32)
        n218 = Index Array(array=w517, index=1) -> (element=w520:i32)
        n219 = Index Array(array=w510, index=1) -> (element=w513:i32)
        n220 = Index Array(array=w527, index (row)=w524) -> (element=w509:dbl[])  [unwired: 1 in]
        n221 = Index Array(array=w522, index (row)=w520) -> (element=w508:dbl[])  [unwired: 1 in]
        n222 = Index Array(array=w515, index (row)=w513) -> (element=w507:dbl[])  [unwired: 1 in]
        n223 = Bundle("iRFWFsAvg"=w509, "iRFWFsAvg"=w508, "iRFWFsAvg"=w507) -> (w506:T29)  [unwired: 1 in]
        n224 = global write "GlobalVariables.vi" "LastUseiRF"(w506) -> ()
        n225 = call <vilib>:"Add State(s) to Queue__JKI_lib_State_Machine.vi"("State(s) in Front (\"\")"="UI: CaliAndiRFLoaded" ("State(s) in Front (\"\")"), "State(s) in (\"\")"=w536) -> ("States Out"=w535:string)  [unwired: 13 in]
      }
      frame "Data: loadLastUseiRF" {
        # "Load last use iRF.\n()"
        n226 = Unbundle By Name(w541) -> ("TempPath"=w540:path)
        n227 = Build Path(base path=w540, name or relative path="iRF.tdms") -> (appended path=w546:path)
        n228 = TDMS Open(11:w546) -> (0:w544:errorcluster, 3:w545:refnum<k34>)  [unwired: 6 in]
        n229 = TDMS Read(0:w545, 11:w544, 12:dbl[][] []) -> (4:w538:refnum<k34>, 10:w542:dbl[][], 15:w537:errorcluster)  [unwired: 5 in, 3 out]
        n230 = TDMS Close(8:w537, 11:w538) -> ()  [unwired: 2 out]
        n231 = case shown="No Error" w537 {
          tunnel: w542 -> [w564 _]
          tunnel: ["UI: CaliAndiRFLoaded" ("State(s) in Front (\"\")") "" ("Empty String Constant")] -> w539
          frame No Error {
            n232 = Index Array(array=w564, index (row)=0) -> (element=w560:dbl[])  [unwired: 1 in]
            n233 = Index Array(array=w564, index (row)=1) -> (element=w557:dbl[])  [unwired: 1 in]
            n234 = Index Array(array=w564, index (row)=2) -> (element=w554:dbl[])  [unwired: 1 in]
            n235 = Add Array Elements(numeric array=w560) -> (sum=w559:dbl)
            n236 = Add Array Elements(numeric array=w557) -> (sum=w556:dbl)
            n237 = Add Array Elements(numeric array=w554) -> (sum=w553:dbl)
            n238 = Divide(x=w560, y=w559) -> (x/y=w558:dbl[])
            n239 = Divide(x=w557, y=w556) -> (x/y=w555:dbl[])
            n240 = Divide(x=w554, y=w553) -> (x/y=w552:dbl[])
            n241 = Bundle(w558, w555, w552) -> (w563:cluster{dbl[], dbl[], dbl[]})  [unwired: 1 in]
            n242 = global write "GlobalVariables.vi" "LastUseiRF"(w563) -> ()
            n243 = Array Size(array=w560) -> (size(s)=→"iRF length":i32)
          }
          frame Error {
          }
        }
        n244 = call <vilib>:"Add State(s) to Queue__JKI_lib_State_Machine.vi"("State(s) in Front (\"\")"=w539, "State(s) in (\"\")"=w551) -> ("States Out"=w550:string)  [unwired: 13 in]
      }
      frame "Data: loadSystemCali" {
        # "Load last use calibration.\n()"
        n245 = Unbundle By Name(w576) -> ("CaliPath"=w575:path)
        n246 = Build Path(base path=w575, name or relative path="Calibration.tdms") -> (appended path=w571:path)
        n247 = call "ReadBGorCali (SubVI).vi"("DataType"=enum16{"BG", "Cali"}."Cali", "error in (no error)"=w570, "file path in"=w571) -> ("error out"=w572:errorcluster, "CtrlVCluster"=w574:T30, "AvgDataCluster"=w573:T31)  [unwired: 6 in]
        n248 = case shown="No Error" w572 {
          tunnel: w574 -> [w591 _]
          tunnel: w573 -> [w590 _]
          frame No Error {
            n249 = Unbundle By Name(w591) -> ("V 1"=w586:dbl[], "V 2"=w585:dbl[], "V 3"=w584:dbl[])
            n250 = Unbundle By Name(w590) -> ("Channel 1"=w589:dbl[], "Channel 2"=w588:dbl[], "Channel 3"=w587:dbl[])
            n251 = Index Array(array=w584) -> (element=w581:dbl)  [unwired: 1 in]
            n252 = Index Array(array=w586) -> (element=w583:dbl)  [unwired: 1 in]
            n253 = Index Array(array=w585) -> (element=w582:dbl)  [unwired: 1 in]
            n254 = Bundle By Name(cluster=T11 {"Ch1 WF"=array[400 elements], "Ch2 WF"=array[400 elements], "Ch3 WF"=array[400 elements], "V1"=0.0, "V2"=0.0, "V3"=0.0} ("LastUseCaliData"), "Ch1 WF"=w589, "Ch2 WF"=w588, "Ch3 WF"=w587, "V1"=w583, "V2"=w582, "V3"=w581) -> (w592:T11)
            n255 = global write "GlobalVariables.vi" "SysCaliData"(w592) -> ()
          }
          frame Error {
          }
        }
        n256 = call <vilib>:"Add State(s) to Queue__JKI_lib_State_Machine.vi"("State(s) in (\"\")"=w580) -> ("States Out"=w579:string)  [unwired: 14 in]
      }
      frame "Data: loadLastUseBG" {
        w600 = enum16{"write", "read"}."write" ("action")
        # "Load last use BG.\n()"
        n257 = Unbundle By Name(w614) -> ("TempPath"=w613:path)
        n258 = Build Path(base path=w613, name or relative path="Background.tdms") -> (appended path=w612:path)
        n259 = call "ReadBGorCali (SubVI).vi"("DataType"=enum16{"BG", "Cali"}."BG", "error in (no error)"=w611, "file path in"=w612) -> ("error out"=w610:errorcluster, "AvgDataCluster"=w605:T31)  [unwired: 6 in, 1 out]
        n260 = Unbundle By Name(w605) -> ("Channel 1"=w596:dbl[], "Channel 2"=w604:dbl[], "Channel 3"=w595:dbl[])
        n261 = call "FLImDAQ_FGV.vi"() -> ("Read data"=w609:T6)  [unwired: 10 in, 1 out]
        n262 = Unbundle By Name(w609) -> ("min record length"=w601:i32)
        n263 = Array Size(array=w595) -> (size(s)=w603:i32)
        "BG length" <- w603
        n264 = Equal?(x=w603, y=w601) -> (x = y?=w602:bool)
        n265 = Select(t="UI: BGLoaded" ("State(s) in Front (\"\")"), s=w602, f="UI: BGSizeError" ("State(s) in Front (\"\")")) -> (s? t:f=w606:string)
        n266 = case shown="True" w602 {
          tunnel: w596 -> [_ w624]
          tunnel: w604 -> [_ w623]
          tunnel: w595 -> [_ w622]
          tunnel: w601 -> [w620 _]
          tunnel: [w619 w624] -> w599
          tunnel: [w619 w623] -> w598
          tunnel: [w619 w622] -> w597
          frame False {
            # "If error set BG all 0, update UI"
            n267 = for {
              N: w620 -> [_]
              tunnel: [0.0] -> w619 mode=indexing
            }
          }
          frame True {
            # "If no error, check size match"
          }
        }
        n268 = call "BG3FGV.vi"("action"=w600, "BG3 in"=w597) -> ()  [unwired: 8 in, 2 out]
        n269 = call "BG1FGV.vi"("action"=w600, "BG1 in"=w599) -> ()  [unwired: 8 in, 2 out]
        n270 = call "BG2FGV.vi"("action"=w600, "BG2 in"=w598) -> ()  [unwired: 8 in, 2 out]
        n271 = call <vilib>:"Add State(s) to Queue__JKI_lib_State_Machine.vi"("State(s) in Front (\"\")"=w606, "State(s) in (\"\")"=w618) -> ("States Out"=w617:string)  [unwired: 13 in]
      }
      frame "Data: loadLastUseMacro" {
        # "Load last use BG and Cali and iRF.\n(It is a separator no-op. You can make a copy of this frame to create a new Data frame)"
        n272 = call <vilib>:"Add State(s) to Queue__JKI_lib_State_Machine.vi"("State(s) in Front (\"\")"="Data: loadLastUseBG\nData: loadSystemCali\nData: loadLastUseiRF\n/*Data: LoadAPDData" ("State(s) in Front (\"\")"), "State(s) in (\"\")"=w630) -> ("States Out"=w629:string)  [unwired: 13 in]
      }
      frame "Data: saveCalibration" {
        # "Average data and save calibration file. [Covers: REQ11]\n(It is a separator no-op. You can make a copy of this frame to create a new Data frame)"
        n273 = Unbundle By Name(w646) -> ("Ch1Data"=w645:dbl[][], "V1"=w644:dbl[], "Ch2Data"=w643:dbl[][], "V2"=w642:dbl[], "Ch3Data"=w641:dbl[][], "V3"=w640:dbl[], "Pathes.CaliPath"=w649:path, "IDs.Cali ID"=w648:i8)
        n274 = Increment(x=w648) -> (x+1=w631:i8)
        n275 = Bundle("Ch1Data"=w645, "V1"=w644) -> (w639:cluster{"Ch1Data":dbl[][], "V1":dbl[]})  [unwired: 1 in]
        n276 = Bundle("Ch2Data"=w643, "V2"=w642) -> (w638:cluster{"Ch2Data":dbl[][], "V2":dbl[]})  [unwired: 1 in]
        n277 = Bundle("Ch3Data"=w641, "V3"=w640) -> (w637:cluster{"Ch3Data":dbl[][], "V3":dbl[]})  [unwired: 1 in]
        n278 = Format Value(string ("")="Calibration" ("default name"), format string="%02d", value (0)=w631) -> (output string=w651:string)
        n279 = Build Path(base path=w649, name or relative path=w651) -> (appended path=w636:path)
        n280 = call "SaveBGorCali (SubVI).vi"("DataType"=enum16{"BG", "Cali"}."Cali", "SytemID"="UCDMC", "BG path"=w636, "error in (no error)"=w635, "Channel 3"=w637, "Channel 2"=w638, "Channel1"=w639) -> ("error out"=w634:errorcluster)  [unwired: 4 in]
        n281 = call <vilib>:"Add State(s) to Queue__JKI_lib_State_Machine.vi"("State(s) in (\"\")"=w654) -> ("States Out"=w653:string)  [unwired: 14 in]
      }
      frame "Data: saveiRF" {
        w679 = enum16{"write", "read"}."read" ("action")
        # "Get iRF from decon stracture and save it on disk.\n(It is a separator no-op. You can make a copy of this frame to create a new Data frame)"
        n282 = Unbundle By Name(w672) -> ("TempPath"=w671:path)
        n283 = call "Ch1DeconEngineFGV.vi"("action(read)"=w679) -> ("Error Out"=w677:errorcluster, "Ch1DeconEngine out"=w678:refnum<class "LaguerreDeconEngineClass.lvclass">)  [unwired: 9 in]
        n284 = call "Ch2DeconEngineFGV.vi"("action(read)"=w679) -> ("Error Out"=w675:errorcluster, "Ch2DeconEngine out"=w676:refnum<class "LaguerreDeconEngineClass.lvclass">)  [unwired: 9 in]
        n285 = call "Ch3DeconEngineFGV.vi"("action(read)"=w679) -> ("Error Out"=w673:errorcluster, "Ch3DeconEngine out"=w674:refnum<class "LaguerreDeconEngineClass.lvclass">)  [unwired: 9 in]
        n286 = Build Path(base path=w671, name or relative path="iRF" ("default name")) -> (appended path=w669:path)
        n287 = call "getIRF.vi"("error in (no error)"=w677, "LaguerreDeconEngineClass in"=w678) -> ("iRF"=w658:dbl[])  [unwired: 7 in, 2 out]
        n288 = call "getIRF.vi"("error in (no error)"=w675, "LaguerreDeconEngineClass in"=w676) -> ("iRF"=w657:dbl[])  [unwired: 7 in, 2 out]
        n289 = call "getIRF.vi"("error in (no error)"=w673, "LaguerreDeconEngineClass in"=w674) -> ("iRF"=w656:dbl[])  [unwired: 7 in, 2 out]
        n290 = Build Array(w658, w657, w656) -> (w664:dbl[][])
        n291 = TDMS Open(8:w668, 10:T12."create or replace" ("operation (0:open)"), 11:w669) -> (0:w665:errorcluster, 3:w666:refnum<k34>)  [unwired: 4 in]
        n292 = Bundle("iRF"=w658, "iRF"=w657, "iRF"=w656) -> (w655:cluster{"iRF":dbl[], "iRF":dbl[], "iRF":dbl[]})  [unwired: 1 in]
        n293 = global write "GlobalVariables.vi" "LastUseiRF"(w655) -> ()
        n294 = TDMS Write(0:w666, 5:"iRF" ("group name in (Untitled)"), 7:string[] ["Ch1", "Ch2", "Ch3"] ("channel name(s) in (Untitled)"), 9:w664, 11:w665) -> (4:w661:refnum<k34>, 15:w660:errorcluster)  [unwired: 1 in, 2 out]
        n295 = TDMS Close(8:w660, 11:w661) -> (0:w659:errorcluster)  [unwired: 1 out]
        n296 = call <vilib>:"Add State(s) to Queue__JKI_lib_State_Machine.vi"("State(s) in (\"\")"=w682) -> ("States Out"=w681:string)  [unwired: 14 in]
      }
      frame "Data: saveBGtoFGV" {
        w688 = enum16{"write", "read"}."write" ("action")
        # "Save BG and pass it to FGV.\n(save BG to disk and set it to FGV)"
        n297 = Unbundle By Name(w691) -> ("Ch1Data"=w690:dbl[][], "Ch2Data"=w689:dbl[][], "Ch3Data"=w687:dbl[][])
        n298 = call "AvgArrayTimeCritical.vi"("2D array"=w690) -> ("1D Avg"=w686:dbl[])  [unwired: 10 in]
        n299 = call "AvgArrayTimeCritical.vi"("2D array"=w689) -> ("1D Avg"=w685:dbl[])  [unwired: 10 in]
        n300 = call "AvgArrayTimeCritical.vi"("2D array"=w687) -> ("1D Avg"=w684:dbl[])  [unwired: 10 in]
        n301 = call "BG1FGV.vi"("action"=w688, "BG1 in"=w686) -> ()  [unwired: 8 in, 2 out]
        n302 = call "BG2FGV.vi"("action"=w688, "BG2 in"=w685) -> ()  [unwired: 8 in, 2 out]
        n303 = call "BG3FGV.vi"("action"=w688, "BG3 in"=w684) -> ()  [unwired: 8 in, 2 out]
        n304 = call <vilib>:"Add State(s) to Queue__JKI_lib_State_Machine.vi"("State(s) in (\"\")"=w694) -> ("States Out"=w693:string)  [unwired: 14 in]
      }
      frame "Data: saveBGtoFile" {
        w713 = "Background" ("name or relative path")
        # "Save BG to file.\n(save BG to disk both data folder and temp folder)"
        n305 = Unbundle By Name(w717) -> ("Pathes.BG Path"=w710:path, "IDs.BG ID"=w709:i8, "Ch1Data"=w707:dbl[][], "V1"=w706:dbl[], "Ch2Data"=w705:dbl[][], "V2"=w704:dbl[], "Ch3Data"=w703:dbl[][], "V3"=w702:dbl[], "TempPath"=w715:path)
        n306 = Increment(x=w709) -> (x+1=w714:i8)
        n307 = Format Value(string ("")=w713, format string="%02d", value (0)=w714) -> (output string=w712:string)
        n308 = Build Path(base path=w715, name or relative path=w713) -> (appended path=w696:path)
        n309 = call "File Dialog2"("start path"=w710, "prompt"="Please select BG name, DO NOT CANCEL!", "default name"=w712) -> ("selected path"=w697:path)  [unwired: 9 in, 3 out]
        n310 = Bundle("Ch1Data"=w707, "V1"=w706) -> (w701:cluster{"Ch1Data":dbl[][], "V1":dbl[]})  [unwired: 1 in]
        n311 = Bundle("Ch2Data"=w705, "V2"=w704) -> (w700:cluster{"Ch2Data":dbl[][], "V2":dbl[]})  [unwired: 1 in]
        n312 = Bundle("Ch3Data"=w703, "V3"=w702) -> (w699:cluster{"Ch3Data":dbl[][], "V3":dbl[]})  [unwired: 1 in]
        n313 = Build Array(w697, w696) -> (w695:path[])
        n314 = for {
          tunnel: w701 -> [w727]
          tunnel: w700 -> [w726]
          tunnel: w699 -> [w725]
          shift-right: [w728] -> w708
          shift-left: w698 -> [w724]
          tunnel: w695 -> [w723] mode=indexing
          n315 = call "SaveBGorCali (SubVI).vi"("DataType"=enum16{"BG", "Cali"}."BG", "SytemID"="UCDMC", "BG path"=w723, "error in (no error)"=w724, "Channel 3"=w725, "Channel 2"=w726, "Channel1"=w727) -> ("error out"=w728:errorcluster)  [unwired: 4 in]
        }
        n316 = call <vilib>:"Add State(s) to Queue__JKI_lib_State_Machine.vi"("State(s) in (\"\")"=w720) -> ("States Out"=w719:string)  [unwired: 14 in]
      }
      frame "Data: showBG" {
        # "Show BG in seperate window.\n()"
        n317 = call "showBG.vi"() -> ()  [unwired: 12 in]
        n318 = call <vilib>:"Add State(s) to Queue__JKI_lib_State_Machine.vi"("State(s) in (\"\")"=w733) -> ("States Out"=w732:string)  [unwired: 14 in]
      }
      frame "Data: irfAlignment" {
        w780 = enum16{"write", "read"}."write" ("action")
        # "do iRF alignment in this state\n(It is a separator no-op. You can make a copy of this frame to create a new Data frame)"
        n319 = Unbundle By Name(w758) -> ("Ch1Data"=w796:dbl[][], "Ch2Data"=w795:dbl[][], "Ch3Data"=w794:dbl[][])
        n320 = call "Ch1DeconEngineFGV.vi"("Error In"=w793) -> ("Error Out"=w791:errorcluster, "Ch1DeconEngine out"=w792:refnum<class "LaguerreDeconEngineClass.lvclass">)  [unwired: 9 in]
        n321 = call "Ch2DeconEngineFGV.vi"("Error In"=w793) -> ("Error Out"=w789:errorcluster, "Ch2DeconEngine out"=w790:refnum<class "LaguerreDeconEngineClass.lvclass">)  [unwired: 9 in]
        n322 = call "Ch3DeconEngineFGV.vi"("Error In"=w793) -> ("Error Out"=w787:errorcluster, "Ch3DeconEngine out"=w788:refnum<class "LaguerreDeconEngineClass.lvclass">)  [unwired: 9 in]
        n323 = call "AvgArray.vi"("2D array in"=w795) -> ("1D Avg out"=w739:dbl[])  [unwired: 10 in]
        n324 = call "AvgArray.vi"("2D array in"=w794) -> ("1D Avg out"=w738:dbl[])  [unwired: 10 in]
        n325 = call "AvgArray.vi"("2D array in"=w796) -> ("1D Avg out"=w740:dbl[])  [unwired: 10 in]
        n326 = call "RemoveDCBG.vi"("WF in"=w740) -> ("DC"=w747:dbl, "WF out"=w737:dbl[])  [unwired: 8 in, 1 out]
        n327 = call "RemoveDCBG.vi"("WF in"=w739) -> ("DC"=w744:dbl, "WF out"=w750:dbl[])  [unwired: 8 in, 1 out]
        n328 = call "RemoveDCBG.vi"("WF in"=w738) -> ("DC"=w742:dbl, "WF out"=w749:dbl[])  [unwired: 8 in, 1 out]
        n329 = call "computeIRFAlignment.vi"("error in (no error)"=w791, "fIRF temp"=w737, "LaguerreDeconEngineClass in"=w792) -> ("error out"=w783:errorcluster, "LaguerreDeconEngineClass out"=w784:refnum<class "LaguerreDeconEngineClass.lvclass">)  [unwired: 6 in, 1 out]
        n330 = call "computeIRFAlignment.vi"("error in (no error)"=w789, "fIRF temp"=w750, "LaguerreDeconEngineClass in"=w790) -> ("error out"=w781:errorcluster, "LaguerreDeconEngineClass out"=w782:refnum<class "LaguerreDeconEngineClass.lvclass">)  [unwired: 6 in, 1 out]
        n331 = call "computeIRFAlignment.vi"("error in (no error)"=w787, "fIRF temp"=w749, "LaguerreDeconEngineClass in"=w788) -> ("error out"=w785:errorcluster, "LaguerreDeconEngineClass out"=w786:refnum<class "LaguerreDeconEngineClass.lvclass">)  [unwired: 6 in, 1 out]
        n332 = call "Ch1DeconEngineFGV.vi"("Error In"=w783, "action(read)"=w780, "Ch1DeconEngine in"=w784) -> ("Error Out"=w778:errorcluster, "Ch1DeconEngine out"=w779:refnum<class "LaguerreDeconEngineClass.lvclass">)  [unwired: 7 in]
        n333 = call "Ch2DeconEngineFGV.vi"("Error In"=w781, "action(read)"=w780, "Ch2DeconEngine in"=w782) -> ("Error Out"=w768:errorcluster, "Ch2DeconEngine out"=w769:refnum<class "LaguerreDeconEngineClass.lvclass">)  [unwired: 7 in]
        n334 = call "Ch3DeconEngineFGV.vi"("Error In"=w785, "action(read)"=w780, "Ch3DeconEngine in"=w786) -> ("Error Out"=w762:errorcluster, "Ch3DeconEngine out"=w763:refnum<class "LaguerreDeconEngineClass.lvclass">)  [unwired: 7 in]
        n335 = call "setfIRF.vi"("error in (no error)"=w762, "fIRF"=w749, "LaguerreDeconEngineClass in"=w763) -> ("error out"=w766:errorcluster, "LaguerreDeconEngineClass out"=w767:refnum<class "LaguerreDeconEngineClass.lvclass">)  [unwired: 7 in]
        n336 = call "setfIRF.vi"("error in (no error)"=w768, "fIRF"=w750, "LaguerreDeconEngineClass in"=w769) -> ("error out"=w772:errorcluster, "LaguerreDeconEngineClass out"=w773:refnum<class "LaguerreDeconEngineClass.lvclass">)  [unwired: 7 in]
        n337 = call "setfIRF.vi"("error in (no error)"=w778, "fIRF"=w737, "LaguerreDeconEngineClass in"=w779) -> ("error out"=w776:errorcluster, "LaguerreDeconEngineClass out"=w777:refnum<class "LaguerreDeconEngineClass.lvclass">)  [unwired: 7 in]
        n338 = Unbundle By Name(w758) -> ("V1"=w735:dbl[], "V2"=w757:dbl[], "V3"=w756:dbl[])
        n339 = call "computeLCs.vi"("error in (no error)"=w776, "LaguerreDeconClass in"=w777) -> ("error out"=w774:errorcluster, "LaguerreDeconClass out"=w775:refnum<class "LaguerreDeconEngineClass.lvclass">)  [unwired: 8 in]
        n340 = call "computeLCs.vi"("error in (no error)"=w772, "LaguerreDeconClass in"=w773) -> ("error out"=w770:errorcluster, "LaguerreDeconClass out"=w771:refnum<class "LaguerreDeconEngineClass.lvclass">)  [unwired: 8 in]
        n341 = call "computeLCs.vi"("error in (no error)"=w766, "LaguerreDeconClass in"=w767) -> ("error out"=w764:errorcluster, "LaguerreDeconClass out"=w765:refnum<class "LaguerreDeconEngineClass.lvclass">)  [unwired: 8 in]
        n342 = call-poly <vilib>:"Mean.vi"("X"=w735) -> ("mean"=w734:dbl)  [unwired: 1 out]
        n343 = call "getFitting.vi"("error in (no error)"=w774, "LaguerreDeconEngineClass in"=w775) -> ("Fitting"=w746:dbl[])  [unwired: 7 in, 2 out]
        n344 = call "getFitting.vi"("error in (no error)"=w770, "LaguerreDeconEngineClass in"=w771) -> ("Fitting"=w743:dbl[])  [unwired: 7 in, 2 out]
        n345 = call "getFitting.vi"("error in (no error)"=w764, "LaguerreDeconEngineClass in"=w765) -> ("Fitting"=w736:dbl[])  [unwired: 7 in, 2 out]
        n346 = call-poly <vilib>:"Mean.vi"("X"=w757) -> ("mean"=w755:dbl)  [unwired: 1 out]
        n347 = Add(x=w747, y=w746) -> (x+y=w748:dbl[])
        n348 = Add(x=w744, y=w743) -> (x+y=w745:dbl[])
        n349 = call-poly <vilib>:"Mean.vi"("X"=w756) -> ("mean"=w754:dbl)  [unwired: 1 out]
        n350 = Add(x=w742, y=w736) -> (x+y=w741:dbl[])
        n351 = Build Array(w740, w748) -> (w761:dbl[][])
        n352 = Build Array(w739, w745) -> (w760:dbl[][])
        n353 = Build Array(w738, w741) -> (w759:dbl[][])
        n354 = Bundle("mean"=w734, "mean"=w755, "mean"=w754) -> (w753:cluster{"mean":dbl, "mean":dbl, "mean":dbl})  [unwired: 1 in]
        n355 = call "Calib_and_iRFAlign_confirm.vi"("Ch4 Data"=w753, "Ch3 Data"=w759, "Ch2 Data"=w760, "Ch1 Data"=w761) -> ("Save?"=w752:bool)  [unwired: 7 in]
        n356 = case shown="True" w752 {
          tunnel: ["" ("Empty String Constant") "Data: saveCalibration\nData: saveiRF\nRun: CaliIncrement"] -> w751
          frame False {
          }
          frame True {
            # "[Covers: REQ2]"
          }
        }
        n357 = call <vilib>:"Add State(s) to Queue__JKI_lib_State_Machine.vi"("State(s) in Front (\"\")"=w751, "State(s) in (\"\")"=w799) -> ("States Out"=w798:string)  [unwired: 13 in]
      }
      frame "Data: parseRunData" {
        # "All APD bias"
        # "flash queue"
        # "Ch3&4"
        # "Ch1&2"
        # "Flash data from queue and save it in structure\n()"
        n358 = local read "Vertical Offset 1"() -> (w803:dbl)
        n359 = local read "Vertical Range 1"() -> (w806:dbl)
        n360 = Power Of 2(x=16.0) -> (2^x=w805:dbl)
        n361 = Divide(x=w806, y=w805) -> (x/y=w804:dbl)
        n362 = Flush Queue(queue=w828, error in (no error)=w827) -> (remaining elements=w822:cluster{"V1":dbl, "V2":dbl, "V3":dbl}[], error out=w823:errorcluster)  [unwired: 1 out]
        n363 = Flush Queue(queue=w834, error in (no error)=w827) -> (remaining elements=w832:cluster{"I16 data":i16[][]}[], error out=w825:errorcluster)  [unwired: 1 out]
        n364 = Flush Queue(queue=w833, error in (no error)=w827) -> (remaining elements=w831:cluster{"I16 data":i16[][]}[], error out=w824:errorcluster)  [unwired: 1 out]
        n365 = for {
          tunnel: w832 -> [w856] mode=indexing
          tunnel: [w855] -> w816 mode=concatenating
          tunnel: [w854] -> w818 mode=concatenating
          tunnel: w804 -> [w852]
          tunnel: w803 -> [w850]
          n366 = Unbundle By Name(w856) -> ("I16 data"=w853:i16[][])
          n367 = Multiply(x=w853, y=w852) -> (x*y=w851:dbl[][])
          n368 = Add(x=w851, y=w850) -> (x+y=w849:dbl[][])
          n369 = call "SeperateChanData.vi"("Input (Ch1&2)"=w849) -> ("Ch1"=w855:dbl[][], "Ch2"=w854:dbl[][])
        }
        n370 = for {
          tunnel: w831 -> [w848] mode=indexing
          tunnel: [w847] -> w817 mode=concatenating
          tunnel: w804 -> [w845]
          tunnel: w803 -> [w843]
          n371 = Unbundle By Name(w848) -> ("I16 data"=w846:i16[][])
          n372 = Multiply(x=w846, y=w845) -> (x*y=w844:dbl[][])
          n373 = Add(x=w844, y=w843) -> (x+y=w842:dbl[][])
          n374 = call "SeperateChanData.vi"("Input (Ch1&2)"=w842) -> ("Ch1"=w847:dbl[][])  [unwired: 1 out]
        }
        n375 = for {
          tunnel: w822 -> [w841] mode=indexing
          tunnel: [w840] -> w813 mode=indexing
          tunnel: [w839] -> w802 mode=indexing
          tunnel: [w838] -> w810 mode=indexing
          n376 = Unbundle By Name(w841) -> ("V1"=w840:dbl, "V2"=w839:dbl, "V3"=w838:dbl)
        }
        n377 = call "FLImDAQ_FGV.vi"() -> ("Read data"=w814:T6)  [unwired: 10 in, 1 out]
        n378 = Unbundle By Name(w814) -> ("Waveform to Avg"=w808:i16)
        n379 = call "DuplicateV(SubVI).vi"("Averaging"=w808, "V in"=w813) -> ("V out"=w812:dbl[])  [unwired: 9 in]
        n380 = call "DuplicateV(SubVI).vi"("Averaging"=w808, "V in"=w802) -> ("V out"=w811:dbl[])  [unwired: 9 in]
        n381 = call "DuplicateV(SubVI).vi"("Averaging"=w808, "V in"=w810) -> ("V out"=w809:dbl[])  [unwired: 9 in]
        n382 = Array Size(array=w817) -> (size(s)=→"data Size":i32[])
        n383 = Array Size(array=w812) -> (size(s)=→"V1 Size":i32)
        n384 = Array Size(array=w811) -> (size(s)=→"V2 Size":i32)
        n385 = Array Size(array=w809) -> (size(s)=→"V3 Size":i32)
        n386 = Bundle By Name(cluster=w829, "Ch1Data"=w816, "Ch2Data"=w818, "Ch3Data"=w817, "V1"=w812, "V2"=w811, "V3"=w809) -> (w830:T19)
        n387 = Merge Errors(w825, w824, w823) -> (w826:errorcluster)
        n388 = call <vilib>:"Add State(s) to Queue__JKI_lib_State_Machine.vi"("State(s) in (\"\")"=w837) -> ("States Out"=w836:string)  [unwired: 14 in]
      }
      frame "Data: saveRunData" {
        w863 = T32 {"DataPath"=path "", "CaseID"="", "RunID"=0, "Ch1Data"=[], "Ch2Data"=[], "Ch3Data"=[], "V1"=[], "V2"=[], "V3"=[], "LaserRepRate"=0, "WFAverage"=0, "RunStartTime"=0}  # Data cluster
        # "Save FLIm data to disk.\n(Save to LV tdms file format)"
        n389 = Unbundle By Name(w867) -> ("Pathes.DataPath"=w862:path, "CaseID"=w876:string, "IDs.RunID"=w865:i8, "Ch1Data"=w875:dbl[][], "Ch2Data"=w874:dbl[][], "Ch3Data"=w861:dbl[][], "V1"=w873:dbl[], "V2"=w872:dbl[], "V3"=w871:dbl[])
        n390 = call "FLImDAQ_FGV.vi"() -> ("Read data"=w859:T6)  [unwired: 10 in, 1 out]
        n391 = Unbundle By Name(w859) -> ("Waveform to Avg"=w858:i16)
        n392 = local read "Laser Rep Rate"() -> (w860:dbl)
        n393 = Increment(x=w865) -> (x+1=w864:i8)
        n394 = local read "RunStartTime"() -> (w857:u32)
        n395 = Bundle By Name(cluster=w863, "DataPath"=w862, "CaseID"=w876, "RunID"=w864, "Ch1Data"=w875, "Ch2Data"=w874, "Ch3Data"=w861, "V1"=w873, "V2"=w872, "V3"=w871, "LaserRepRate"=w860, "WFAverage"=w858, "RunStartTime"=w857) -> (w870:T32)
        n396 = call "SaveRunData(SubVI).vi"("Data cluster"=w870, "error in (no error)"=w869) -> ("error out"=w866:errorcluster)  [unwired: 13 in]
        n397 = flat-sequence {
          tunnel: w867 -> [w884]
          tunnel: [w881] -> w868
          tunnel: w866 -> [_]
          frame #0 {
            w882 = dbl[][] [] ("Ch1Data")
            w883 = dbl[] [] ("V1")
            n398 = Bundle By Name(cluster=w884, "Ch1Data"=w882, "Ch2Data"=w882, "Ch3Data"=w882, "V1"=w883, "V2"=w883, "V3"=w883) -> (w881:T19)
          }
        }
        n399 = case shown="No Error" w866 {
          tunnel: ["Run: Increment" "" ("Empty String Constant")] -> w877
          frame No Error {
          }
          frame Error {
          }
        }
        n400 = call <vilib>:"Add State(s) to Queue__JKI_lib_State_Machine.vi"("State(s) in Front (\"\")"=w877, "State(s) in (\"\")"=w880) -> ("States Out"=w879:string)  [unwired: 13 in]
      }
      frame "Data: Cleanup" {
        # "Cleanup any data and references, here.\n(this is called automatically, by the Macro: Exit)"
        n401 = Unbundle By Name(w888) -> ("Core.Current VI Reference"=w891:refnum<vi>)
        n402 = Close Reference(reference=w891, error in (no error)=w890) -> (error out=w889:errorcluster)
        n403 = call <vilib>:"Add State(s) to Queue__JKI_lib_State_Machine.vi"("State(s) in (\"\")"=w893) -> ("States Out"=w892:string)  [unwired: 14 in]
      }
      frame "---------- Core ----------" {
        # "Do not put any code in this frame.\n(it is a separator no-op)"
        n404 = call <vilib>:"Add State(s) to Queue__JKI_lib_State_Machine.vi"("State(s) in (\"\")"=w898) -> ("States Out"=w897:string)  [unwired: 14 in]
      }
      frame Default {
        w909 = 42 items=["No error", "Argument error", "Memory is full", "Out of zone", "End of file", "File already open", "Generic file I/O error", "File not found", "File permission error", "Disk is full", "Duplicate path", "Too many files open", "System feature not enabled", "Resource file not found", "Cannot add resource", "Resource not found", "Image not found", "Image memory error", "Pen does not exist", "Config type invalid", "Config token not found", "Config parse error", "Config memory error", "Bad external code format", "Bad external code offset", "External code not present", "Null window", "Destroy window error", "Null menu", "Print aborted", "Bad print record", "Print driver error", "Windows error during printing", "Memory error during printing", "Print dialog error", "Generic print error", "Invalid device refnum", "Device not found", "Device parameter error", "Device unit error", "Cannot open device", "Device call aborted", "Generic error", "Cancelled by user", "Object ID too low", "Object ID too high", "Object not in heap", "Unknown heap", "Unknown object (invalid DefProc)", "Unknown object (DefProc not in table)", "Message out of range", "Invalid (null) method", "Unknown message", "Manager call not supported", "Bad address", "Network operation in progress", "Network operation timed out", "Connection is busy", "Network attribute not supported", "Network error", "Address in use", "System out of memory", "Connection aborted", "Connection refused", "Not connected", "Already connected", "Connection closed", "Initialization error (interapplication manager)", "Bad occurrence", "Wait on unbound occurrence handler", "Occurrence queue overflow", "Datalog type conflict", "Unused", "Unrecognized type (interapplication manager)", "Memory corrupt", "Failed to make temporary DLL", "Old CIN version", "Drag socket not found", "Failed to load drop-object", "Failed to register OLE object", "Failed to release OLE object", "Format specifier type mismatch", "Unknown format specifier", "Too few format specifiers", "Too many format specifiers", "Scan failed", "Newer CIN version", "Error converting to variant", "Runtime menu error", "Password tampered", "Variant attribute not found", "Incompatible variant data type", "Event data is not available", "Event Store is not present", "Occurrence is not found", "Event Queue is not created", "Event info is not available", "Refnum passed is NULL", "Error retrieving Class GUID", "Error retrieving CoClass GUID", "Error retrieving TypeLib GUID.", "Bad built application magic bytes.", "Specific driver is different from the specific driver associated with the Logical Name.", "There is no session opened to the class driver.", "Max Error", "MAX - Error with config objects", "MAX - Error loading configuration", "MAX - Group not supported"]
        # "Current State"
        # "Do not delete, rename, or modify this frame.\n(this is used to capture unhandled states and typos)"
        # "Handle mistyped state name (developer tool)"
        n405 = Format Into String(format string="Software Exception: Unhandled State \"%s\"." ("message"), error in=w905, w900) -> (resulting string=w908:string, error out=w907:errorcluster)  [unwired: 1 in]
        n406 = call <vilib>:"Error Cluster From Error Code.vi"("show call chain? (False)"=TRUE, "error in (no error)"=w907, "error message (\"\")"=w908, "error code (0)"=w909) -> ("error out"=w906:errorcluster)  [unwired: 5 in]
        n407 = call <vilib>:"Add State(s) to Queue__JKI_lib_State_Machine.vi"("State(s) in (\"\")"=w904) -> ("States Out"=w903:string)  [unwired: 14 in]
      }
      frame "Initialize Core Data" {
        # "Build default path based on the location of project"
        # "Do not delete, rename, or modify this frame.\n(this is used to determine panel behavior on exit)"
        # "originally closed?"
        # "exe?"
        # "If panel starts closed or is an EXE, then close it when we exit"
        n408 = call <vilib>:"Application Directory.vi"() -> ("Application Directory"=w913:path)
        n409 = property on="Property Node" class="App"() -> ("App.Kind"=w927:T14)  [unwired: 2 in, 2 out]
        n410 = property on="Property Node" class="VI"() -> ("FP.State"=w921:T13)  [unwired: 2 in, 2 out]
        n411 = control-ref of="Current VI Reference"() -> (w922:refnum<vi>)
        n412 = Equal?(x=w921, y=T13."Closed" ("Front Panel Window:State")) -> (x = y?=w919:bool)
        n413 = Equal?(x=w927, y=T14."Run Time System" ("Application:Kind")) -> (x = y?=w925:bool)
        n414 = Build Path(base path=w913, name or relative path="Data") -> (appended path=w917:path)
        n415 = Build Path(base path=w913, name or relative path="SystemTemp") -> (appended path=w914:path)
        n416 = Build Path(base path=w913, name or relative path="SystemCalibrationFile") -> (appended path=w911:path)
        n417 = Or(x=w919, y=w925) -> (x .or. y?=w923:bool)
        n418 = Bundle By Name(cluster=w924, "Core.Current VI Reference"=w922, "Core.Close Panel on Exit?"=w923, "DefaultPath"=w917, "TempPath"=w914, "CaliPath"=w911) -> (w929:T19)
        n419 = call <vilib>:"Add State(s) to Queue__JKI_lib_State_Machine.vi"("State(s) in (\"\")"=w931) -> ("States Out"=w930:string)  [unwired: 14 in]
      }
      frame "Error Handler" {
        # "Unhandled Error -- Display it"
        # "Handle any errors here.\nYou can also output any states to clean-up after errors occur"
        # "Clear error"
        n420 = Unbundle By Name(w932) -> ("code"=w934:i32)
        n421 = case shown="5001" w934 {
          tunnel: ["Macro: Exit" w944 w950] -> w933
          tunnel: w932 -> [w940 _ _]
          frame Default {
            w942 = T33 1 items=["no dialog", "OK message", "continue or stop message", "OK message + warnings", "continue/stop + warnings"] ("type of dialog (OK msg:1)")
            n422 = call <vilib>:"General Error Handler.vi"("type of dialog (OK msg:1)"=w942, "error in (no error)"=w940) -> ()  [unwired: 9 in, 5 out]
          }
          frame 5002 {
            n423 = Two Button Dialog(message="Laser interlock open! Please close interlock and try again! ", 1:"Safely Shutdown" ("F button name (\"Cancel\")"), 2:"OK" ("T button name (\"OK\")")) -> (T button?=w945:bool)
            n424 = case shown="True" w945 {
              tunnel: ["Macro: Exit" "355 Laser: CheckControllerStatus"] -> w944
              frame False {
              }
              frame True {
              }
            }
          }
          frame 5001 {
            n425 = Two Button Dialog(message="Unable to connect to imaging computer, do you want to run data aquisiton alone? ", 1:"No" ("F button name (\"Cancel\")"), 2:"Yes" ("T button name (\"OK\")")) -> (T button?=w951:bool)
            n426 = case shown="False" w951 {
              tunnel: ["Macro: Exit" "" ("Empty String Constant")] -> w950
              frame False {
              }
              frame True {
              }
            }
          }
        }
        n427 = call <vilib>:"Add State(s) to Queue__JKI_lib_State_Machine.vi"("State(s) in Front (\"\")"=w933, "State(s) in (\"\")"=w939) -> ("States Out"=w938:string)  [unwired: 13 in]
      }
      frame "Exit" {
        # "Do not put any code in this frame.\n(No errors that occur here will be handled.)"
        n428 = call <vilib>:"Add State(s) to Queue__JKI_lib_State_Machine.vi"("State(s) in (\"\")"=w962) -> ("States Out"=w961:string)  [unwired: 14 in]
      }
      frame "---------- Case ----------" {
        # "Template Separator\n(You can make a copy of, or modify, this frame)"
        n429 = call <vilib>:"Add State(s) to Queue__JKI_lib_State_Machine.vi"("State(s) in (\"\")"=w967) -> ("States Out"=w966:string)  [unwired: 14 in]
      }
      frame "Case: getCaliID" {
        # "Get Calibration file #\n(You can make a copy of, or modify, this frame)"
        n430 = Unbundle By Name(w968) -> ("Pathes.CaliPath"=w971:path)
        n431 = call <vilib>:"Recursive File List.vi"("pattern"="*.tdms", "Treat LLBs as Folders?"=FALSE, "Folder Path"=w971) -> ("All Files in Dir"=w976:path[])  [unwired: 4 in, 4 out]
        n432 = for {
          tunnel: w976 -> [w986] mode=indexing
          tunnel: [w985] -> w975 mode=indexing
          tunnel: "Calibration" -> [w982]
          n433 = Strip Path(path=w986) -> (name=w983:string)  [unwired: 1 out]
          n434 = Search and Replace String(input string=w983, search string=w982) -> (result string=w981:string)  [unwired: 6 in, 3 out]
          n435 = Scan From String(format string="%d" ("string"), input string=w981) -> (output 1=w985:i32)  [unwired: 3 in, 3 out]
        }
        n436 = Array Max & Min(array=w975) -> (max value=w974:i32)  [unwired: 3 out]
        n437 = Bundle By Name(cluster=w968, "IDs.Cali ID"=w974) -> (w969:T19)
        n438 = call <vilib>:"Add State(s) to Queue__JKI_lib_State_Machine.vi"("State(s) in (\"\")"=w980) -> ("States Out"=w979:string)  [unwired: 14 in]
      }
      frame "Case: getBGID" {
        # "Get background #\n(You can make a copy of, or modify, this frame)"
        n439 = Unbundle By Name(w989) -> ("Pathes.BG Path"=w994:path)
        n440 = call <vilib>:"Recursive File List.vi"("pattern"="*.tdms", "Treat LLBs as Folders?"=FALSE, "Folder Path"=w994) -> ("All Files in Dir"=w992:path[])  [unwired: 4 in, 4 out]
        n441 = for {
          tunnel: w992 -> [w1009] mode=indexing
          tunnel: "Background" ("name or relative path") -> [w1007]
          shift-right: [w1000] -> w987
          shift-left: 0 -> [w1004]
          n442 = Strip Path(path=w1009) -> (name=w1008:string)  [unwired: 1 out]
          n443 = Search and Replace String(input string=w1008, search string=w1007) -> (number of replacements=w1006:i32)  [unwired: 6 in, 3 out]
          n444 = Greater Than 0?(x=w1006) -> (x > 0?=w1005:bool)
          n445 = Select(t=1, s=w1005, f=0) -> (s? t:f=w1003:i32)
          n446 = Add(x=w1003, y=w1004) -> (x+y=w1000:i32)
        }
        n447 = Bundle By Name(cluster=w989, "IDs.BG ID"=w987) -> (w990:T19)
        n448 = call <vilib>:"Add State(s) to Queue__JKI_lib_State_Machine.vi"("State(s) in (\"\")"=w999) -> ("States Out"=w998:string)  [unwired: 14 in]
      }
      frame "Case: getRunID" {
        # "Check folder for run ID\n(You can make a copy of, or modify, this frame)"
        n449 = Unbundle By Name(w1019) -> ("Pathes.DataPath"=w1018:path, "CaseID"=w1014:string)
        n450 = Build Array("Background" ("name or relative path"), "Calibration", "3DScanData" ("element")) -> (w1024:string[])
        n451 = call <vilib>:"Recursive File List.vi"("Folders to Exclude"=w1024, "pattern"="*.tdms", "Treat LLBs as Folders?"=FALSE, "Folder Path"=w1018) -> ("All Files in Dir"=w1015:path[])  [unwired: 3 in, 4 out]
        n452 = for {
          tunnel: w1015 -> [w1033] mode=indexing
          tunnel: [w1032] -> w1021 mode=indexing
          tunnel: w1014 -> [w1029]
          n453 = Strip Path(path=w1033) -> (name=w1030:string)  [unwired: 1 out]
          n454 = Search and Replace String(input string=w1030, search string=w1029) -> (result string=w1028:string)  [unwired: 6 in, 3 out]
          n455 = Scan From String(format string="_%d" ("string"), input string=w1028) -> (output 1=w1032:i32)  [unwired: 3 in, 3 out]
        }
        n456 = Array Max & Min(array=w1021) -> (max value=w1012:i32)  [unwired: 3 out]
        n457 = Bundle By Name(cluster=w1019, "IDs.RunID"=w1012) -> (w1020:T19)
        n458 = call "RunIDFGV.vi"("Error In"=w1010, "RunID in"=w1012) -> ("Error Out"=w1011:errorcluster)  [unwired: 8 in, 1 out]
        n459 = call <vilib>:"Add State(s) to Queue__JKI_lib_State_Machine.vi"("State(s) in (\"\")"=w1027) -> ("States Out"=w1026:string)  [unwired: 14 in]
      }
      frame "Case: CreatFileStruct" {
        # "Creat case file structure"
        n460 = Unbundle By Name(w1047) -> ("DefaultPath"=w1053:path, "CaseID"=w1040:string)
        n461 = Build Path(base path=w1053, name or relative path=w1040) -> (appended path=w1052:path)
        n462 = call <vilib>:"Check if File or Folder Exists.vi"("error in (no error)"=w1046, "path"=w1052) -> ("error out"=w1049:errorcluster, "file or folder exists?"=w1051:bool, "dup path"=w1050:path)  [unwired: 7 in]
        n463 = case shown="True" w1051 {
          tunnel: w1050 -> [w1070 w1078]
          tunnel: w1049 -> [w1068 w1073]
          tunnel: [w1062 w1078] -> w1038
          tunnel: [w1066 w1080] -> w1037
          tunnel: [u32 0 u32 0] -> w1036
          tunnel: [w1064 w1083] -> w1044
          tunnel: "Background" ("name or relative path") -> [w1063 w1075]
          tunnel: "Calibration" -> [w1061 w1074]
          tunnel: [w1057 w1076] -> w1041
          tunnel: w1040 -> [_ _]
          tunnel: ["" ("Empty String Constant") "Case: getRunID\nCase: getBGID\nCase: getCaliID\nUI: Update"] -> w1039
          frame False {
            # "Folder not exist. Creat folders."
            n464 = Create Folder(path (use dialog)=w1070, error in=w1068) -> (created path=w1062:path, error out=w1059:errorcluster)  [unwired: 1 in, 1 out]
            n465 = Build Path(base path=w1062, name or relative path=w1061) -> (appended path=w1060:path)
            n466 = Build Path(base path=w1062, name or relative path=w1063) -> (appended path=w1069:path)
            n467 = Create Folder(path (use dialog)=w1069, error in=w1059) -> (created path=w1064:path, error out=w1065:errorcluster)  [unwired: 1 in, 1 out]
            n468 = Create Folder(path (use dialog)=w1060, error in=w1059) -> (created path=w1057:path, error out=w1058:errorcluster)  [unwired: 1 in, 1 out]
            n469 = Merge Errors(w1065, w1058) -> (w1066:errorcluster)
          }
          frame True {
            # "Folder exsit, check file #"
            n470 = Build Path(base path=w1078, name or relative path=w1074) -> (appended path=w1079:path)
            n471 = Build Path(base path=w1078, name or relative path=w1075) -> (appended path=w1084:path)
            n472 = call <vilib>:"Check if File or Folder Exists.vi"("path"=w1079) -> ("file or folder exists?"=w1077:bool, "dup path"=w1076:path)  [unwired: 8 in, 1 out]
            n473 = call <vilib>:"Check if File or Folder Exists.vi"("path"=w1084) -> ("file or folder exists?"=w1082:bool, "dup path"=w1083:path)  [unwired: 8 in, 1 out]
            n474 = And(x=w1082, y=w1077) -> (x .and. y?=w1081:bool)
            n475 = case shown="False" w1081 {
              tunnel: w1073 -> [_ w1086]
              tunnel: [errorcluster {"status"=TRUE, "code"=5003, "source"="File structure error."} ("error out") w1086] -> w1080
              frame False {
              }
              frame True {
              }
            }
          }
        }
        n476 = Bundle By Name(cluster=w1047, "Pathes.DataPath"=w1038, "Pathes.BG Path"=w1044, "Pathes.CaliPath"=w1041, "IDs.RunID"=w1036, "IDs.BG ID"=w1036, "IDs.Cali ID"=w1036) -> (w1048:T19)
        n477 = call "DataRootPathFGV.vi"("Error In"=w1037, "PathIn"=w1038) -> ("Error Out"=w1035:errorcluster)  [unwired: 8 in, 1 out]
        n478 = call "RunIDFGV.vi"("Error In"=w1035, "RunID in"=w1036) -> ("Error Out"=w1034:errorcluster)  [unwired: 8 in, 1 out]
        n479 = call <vilib>:"Add State(s) to Queue__JKI_lib_State_Machine.vi"("State(s) in Front (\"\")"=w1039, "State(s) in (\"\")"=w1055) -> ("States Out"=w1054:string)  [unwired: 13 in]
      }
      frame "Case: GetID" {
        # "Template Separator\n(You can make a copy of, or modify, this frame)"
        n480 = call "set_subjectID.vi"() -> ("subject_id"=w1087:string)  [unwired: 10 in]
        n481 = Bundle By Name(cluster=w1089, "CaseID"=w1087) -> (w1090:T19)
        n482 = call <vilib>:"Add State(s) to Queue__JKI_lib_State_Machine.vi"("State(s) in (\"\")"=w1093) -> ("States Out"=w1092:string)  [unwired: 14 in]
      }
      frame "---------- DeconEngine ----------" {
        # "start data aquisition and then set irfAligh to ture and decon channel to 1,2 and 3."
        # "Template Separator\n(You can make a copy of, or modify, this frame)"
        n483 = call <vilib>:"Add State(s) to Queue__JKI_lib_State_Machine.vi"("State(s) in (\"\")"=w1098) -> ("States Out"=w1097:string)  [unwired: 14 in]
      }
      frame "DeconEngine: InitilizeMacro" {
        # "start data aquisition and then set irfAligh to ture and decon channel to 1,2 and 3."
        # "Initilize Decon Engine for all channel\n(You can make a copy of, or modify, this frame)"
        n484 = call <vilib>:"Add State(s) to Queue__JKI_lib_State_Machine.vi"("State(s) in Front (\"\")"="DeconEngine: InitializeCh1\nDeconEngine: InitializeCh2\nDeconEngine: InitializeCh3" ("State(s) in Front (\"\")"), "State(s) in (\"\")"=w1104) -> ("States Out"=w1103:string)  [unwired: 13 in]
      }
      frame "DeconEngine: InitializeCh1" {
        w1128 = refnum<class "LaguerreDeconEngineClass.lvclass"> refnum  # Ch1DeconObj
        # "Initilize Laguerre Deconvolution engine Object\n(You can make a copy of, or modify, this frame)"
        n485 = call "FLImDAQ_FGV.vi"("error in (no error)"=w1113) -> ("error out"=w1124:errorcluster, "Read data"=w1123:T6)  [unwired: 9 in]
        n486 = global read "GlobalVariables.vi" "LastUseiRF"() -> (w1106:T34)
        n487 = Unbundle By Name(w1123) -> ("min record length"=w1122:i32)
        n488 = call "setLaguerreOrder.vi"("error in (no error)"=w1124, "LaguerreOrder"=u32 12, "LaguerreDeconClass in"=w1128) -> ("error out"=w1125:errorcluster, "LaguerreDeconClass out"=w1126:refnum<class "LaguerreDeconEngineClass.lvclass">)  [unwired: 7 in]
        n489 = Unbundle By Name(w1106) -> ("Ch1 iRF"=w1105:dbl[])
        n490 = call "setDataLength.vi"("error in (no error)"=w1125, "dataLength"=w1122, "LaguerreDeconClass in"=w1126) -> ("error out"=w1121:errorcluster, "LaguerreDeconClass out"=w1120:refnum<class "LaguerreDeconEngineClass.lvclass">)  [unwired: 7 in]
        n491 = call "setIRF.vi"("error in (no error)"=w1121, "iRF"=w1105, "LaguerreDeconClass in"=w1120) -> ("error out"=w1118:errorcluster, "LaguerreDeconClass out"=w1119:refnum<class "LaguerreDeconEngineClass.lvclass">)  [unwired: 7 in]
        n492 = call "computeAlpha.vi"("error in (no error)"=w1118, "LaguerreDeconClass in"=w1119) -> ("error out"=w1116:errorcluster, "LaguerreDeconClass out"=w1117:refnum<class "LaguerreDeconEngineClass.lvclass">)  [unwired: 8 in]
        n493 = call "dataInitilize.vi"("error in (no error)"=w1116, "LaguerreDeconClass in"=w1117) -> ("error out"=w1114:errorcluster, "LaguerreDeconClass out"=w1115:refnum<class "LaguerreDeconEngineClass.lvclass">)  [unwired: 8 in]
        n494 = call "computeDeconMatrix.vi"("error in (no error)"=w1114, "LaguerreDeconClass in"=w1115) -> ("error out"=w1110:errorcluster, "LaguerreDeconClass out"=w1112:refnum<class "LaguerreDeconEngineClass.lvclass">)  [unwired: 8 in]
        n495 = call "Ch1DeconEngineFGV.vi"("Error In"=w1110, "action(read)"=enum16{"write", "read"}."write" ("action"), "Ch1DeconEngine in"=w1112) -> ("Error Out"=w1109:errorcluster)  [unwired: 7 in, 1 out]
        n496 = call <vilib>:"Add State(s) to Queue__JKI_lib_State_Machine.vi"("State(s) in (\"\")"=w1130) -> ("States Out"=w1129:string)  [unwired: 14 in]
      }
      frame "DeconEngine: InitializeCh2" {
        w1154 = refnum<class "LaguerreDeconEngineClass.lvclass"> refnum  # Ch2DeconObj
        # "Initilize Laguerre Deconvolution engine Object\n(You can make a copy of, or modify, this frame)"
        n497 = global read "GlobalVariables.vi" "LastUseiRF"() -> (w1132:T34)
        n498 = call "FLImDAQ_FGV.vi"("error in (no error)"=w1140) -> ("error out"=w1133:errorcluster, "Read data"=w1150:T6)  [unwired: 9 in]
        n499 = call "setLaguerreOrder.vi"("error in (no error)"=w1133, "LaguerreOrder"=u32 12, "LaguerreDeconClass in"=w1154) -> ("error out"=w1151:errorcluster, "LaguerreDeconClass out"=w1152:refnum<class "LaguerreDeconEngineClass.lvclass">)  [unwired: 7 in]
        n500 = Unbundle By Name(w1150) -> ("min record length"=w1149:i32)
        n501 = Unbundle By Name(w1132) -> ("Ch2 iRF"=w1131:dbl[])
        n502 = call "setDataLength.vi"("error in (no error)"=w1151, "dataLength"=w1149, "LaguerreDeconClass in"=w1152) -> ("error out"=w1148:errorcluster, "LaguerreDeconClass out"=w1147:refnum<class "LaguerreDeconEngineClass.lvclass">)  [unwired: 7 in]
        n503 = call "setIRF.vi"("error in (no error)"=w1148, "iRF"=w1131, "LaguerreDeconClass in"=w1147) -> ("error out"=w1145:errorcluster, "LaguerreDeconClass out"=w1146:refnum<class "LaguerreDeconEngineClass.lvclass">)  [unwired: 7 in]
        n504 = call "computeAlpha.vi"("error in (no error)"=w1145, "LaguerreDeconClass in"=w1146) -> ("error out"=w1143:errorcluster, "LaguerreDeconClass out"=w1144:refnum<class "LaguerreDeconEngineClass.lvclass">)  [unwired: 8 in]
        n505 = call "dataInitilize.vi"("error in (no error)"=w1143, "LaguerreDeconClass in"=w1144) -> ("error out"=w1141:errorcluster, "LaguerreDeconClass out"=w1142:refnum<class "LaguerreDeconEngineClass.lvclass">)  [unwired: 8 in]
        n506 = call "computeDeconMatrix.vi"("error in (no error)"=w1141, "LaguerreDeconClass in"=w1142) -> ("error out"=w1137:errorcluster, "LaguerreDeconClass out"=w1139:refnum<class "LaguerreDeconEngineClass.lvclass">)  [unwired: 8 in]
        n507 = call "Ch2DeconEngineFGV.vi"("Error In"=w1137, "action(read)"=enum16{"write", "read"}."write" ("action"), "Ch2DeconEngine in"=w1139) -> ("Error Out"=w1136:errorcluster)  [unwired: 7 in, 1 out]
        n508 = call <vilib>:"Add State(s) to Queue__JKI_lib_State_Machine.vi"("State(s) in (\"\")"=w1156) -> ("States Out"=w1155:string)  [unwired: 14 in]
      }
      frame "DeconEngine: InitializeCh3" {
        w1157 = refnum<class "LaguerreDeconEngineClass.lvclass"> refnum  # Ch3DeconObj
        # "Initilize Laguerre Deconvolution engine Object\n(You can make a copy of, or modify, this frame)"
        n509 = call "FLImDAQ_FGV.vi"("error in (no error)"=w1166) -> ("error out"=w1177:errorcluster, "Read data"=w1176:T6)  [unwired: 9 in]
        n510 = global read "GlobalVariables.vi" "LastUseiRF"() -> (w1159:T34)
        n511 = call "setLaguerreOrder.vi"("error in (no error)"=w1177, "LaguerreOrder"=u32 12, "LaguerreDeconClass in"=w1157) -> ("error out"=w1178:errorcluster, "LaguerreDeconClass out"=w1179:refnum<class "LaguerreDeconEngineClass.lvclass">)  [unwired: 7 in]
        n512 = Unbundle By Name(w1176) -> ("min record length"=w1175:i32)
        n513 = Unbundle By Name(w1159) -> ("Ch3 iRF"=w1158:dbl[])
        n514 = call "setDataLength.vi"("error in (no error)"=w1178, "dataLength"=w1175, "LaguerreDeconClass in"=w1179) -> ("error out"=w1174:errorcluster, "LaguerreDeconClass out"=w1173:refnum<class "LaguerreDeconEngineClass.lvclass">)  [unwired: 7 in]
        n515 = call "setIRF.vi"("error in (no error)"=w1174, "iRF"=w1158, "LaguerreDeconClass in"=w1173) -> ("error out"=w1171:errorcluster, "LaguerreDeconClass out"=w1172:refnum<class "LaguerreDeconEngineClass.lvclass">)  [unwired: 7 in]
        n516 = call "computeAlpha.vi"("error in (no error)"=w1171, "LaguerreDeconClass in"=w1172) -> ("error out"=w1169:errorcluster, "LaguerreDeconClass out"=w1170:refnum<class "LaguerreDeconEngineClass.lvclass">)  [unwired: 8 in]
        n517 = call "dataInitilize.vi"("error in (no error)"=w1169, "LaguerreDeconClass in"=w1170) -> ("error out"=w1167:errorcluster, "LaguerreDeconClass out"=w1168:refnum<class "LaguerreDeconEngineClass.lvclass">)  [unwired: 8 in]
        n518 = call "computeDeconMatrix.vi"("error in (no error)"=w1167, "LaguerreDeconClass in"=w1168) -> ("error out"=w1163:errorcluster, "LaguerreDeconClass out"=w1165:refnum<class "LaguerreDeconEngineClass.lvclass">)  [unwired: 8 in]
        n519 = call "Ch3DeconEngineFGV.vi"("Error In"=w1163, "action(read)"=enum16{"write", "read"}."write" ("action"), "Ch3DeconEngine in"=w1165) -> ("Error Out"=w1162:errorcluster)  [unwired: 7 in, 1 out]
        n520 = call <vilib>:"Add State(s) to Queue__JKI_lib_State_Machine.vi"("State(s) in (\"\")"=w1182) -> ("States Out"=w1181:string)  [unwired: 14 in]
      }
      frame "---------- Digitizer ----------" {
        # "Template Separator\n(You can make a copy of, or modify, this frame)"
        n521 = call <vilib>:"Add State(s) to Queue__JKI_lib_State_Machine.vi"("State(s) in (\"\")"=w1187) -> ("States Out"=w1186:string)  [unwired: 14 in]
      }
      frame "Digitizer: Initialize" {
        # "reset digitizer to everytime the system runs"
        # "reset digitizer to everytime the system runs"
        # "Initialize digitizer.\nInitialize both digitizer and update status."
        n522 = call "FLImDAQ_FGV.vi"("error in (no error)"=w1195) -> ("error out"=w1189:errorcluster, "Read data"=w1194:T6)  [unwired: 9 in]
        n523 = Unbundle By Name(w1197) -> ("SysConfigCluster.Ch1Enable?"=w1202:bool, "SysConfigCluster.Ch2Enable?"=w1201:bool, "SysConfigCluster.Ch3Enable?"=w1199:bool)
        n524 = Unbundle By Name(w1194) -> ("Digitizer 1"=w1190:refnum<k15>, "Digitizer 2"=w1193:refnum<k15>)
        n525 = property on="Digitizer" class="Bool (strict)"("Blinking"=TRUE) -> ()  [unwired: 2 in, 2 out]
        n526 = Or(x=w1202, y=w1201) -> (x .or. y?=w1200:bool)
        n527 = case shown="True" w1200 {
          tunnel: w1189 -> [w1210 w1213]
          tunnel: [w1210 w1212] -> w1191
          tunnel: w1190 -> [_ w1214]
          frame False {
          }
          frame True {
            n528 = call <instrlib>:"niScope Initialize.vi"("resource name"=w1214, "reset device"=TRUE, "error in"=w1213) -> ("error out"=w1212:errorcluster)  [unwired: 11 in, 1 out]
          }
        }
        n529 = case shown="True" w1199 {
          tunnel: w1189 -> [w1205 w1207]
          tunnel: [w1205 w1209] -> w1196
          tunnel: w1193 -> [_ w1208]
          frame False {
          }
          frame True {
            n530 = call <instrlib>:"niScope Initialize.vi"("resource name"=w1208, "reset device"=TRUE, "error in"=w1207) -> ("error out"=w1209:errorcluster)  [unwired: 11 in, 1 out]
          }
        }
        n531 = Merge Errors(w1191, w1196) -> (w1188:errorcluster)
        n532 = call <vilib>:"Add State(s) to Queue__JKI_lib_State_Machine.vi"("State(s) in (\"\")"=w1204) -> ("States Out"=w1203:string)  [unwired: 14 in]
      }
      frame "Digitizer: Config" {
        # "Synchronize is taking time ~3s."
        # "Config  digitizer\nCall subVi to config digitizer"
        n533 = call "FLImDAQ_FGV.vi"() -> ("Read data"=w1232:T6)  [unwired: 10 in, 1 out]
        n534 = Unbundle By Name(w1241) -> ("SysConfigCluster.Ch1Enable?"=w1249:bool, "SysConfigCluster.Ch2Enable?"=w1248:bool, "SysConfigCluster.Ch3Enable?"=w1246:bool, "FLImDAQ"=w1243:T26)
        n535 = Unbundle By Name(w1232) -> ("Digitizer 1"=w1235:refnum<k15>, "Digitizer 2"=w1234:refnum<k15>)
        n536 = property on="Digitizer" class="Bool (strict)"(error in=w1236, "Blinking"=TRUE) -> (error out=w1237:errorcluster)  [unwired: 1 in, 1 out]
        n537 = Or(x=w1249, y=w1248) -> (x .or. y?=w1247:bool)
        n538 = case shown="True" w1247 {
          tunnel: w1243 -> [_ w1263]
          tunnel: w1237 -> [w1258 w1262]
          tunnel: [w1258 w1261] -> w1244
          tunnel: w1235 -> [_ w1260]
          frame False {
          }
          frame True {
            n539 = call "DigitizerConfig.vi"("ExportTrigger? (F)"=TRUE, "error in (no error)"=w1262, "FLImDAQ"=w1263, "IVI Refnum in"=w1260) -> ("error out"=w1261:errorcluster)  [unwired: 6 in, 1 out]
          }
        }
        n540 = case shown="True" w1246 {
          tunnel: w1243 -> [_ w1257]
          tunnel: w1244 -> [w1252 w1256]
          tunnel: [w1252 w1255] -> w1220
          tunnel: w1234 -> [_ w1253]
          frame False {
          }
          frame True {
            n541 = call "DigitizerConfig.vi"("Config Trigger? (T)"=FALSE ("Config Trigge(T)r:"), "error in (no error)"=w1256, "FLImDAQ"=w1257, "IVI Refnum in"=w1253) -> ("error out"=w1255:errorcluster)  [unwired: 6 in, 1 out]
          }
        }
        n542 = call "Digitizer1_FGV.vi"("error in (no error)"=w1220) -> ("error out"=w1230:errorcluster, "Read data"=w1231:refnum<k15>)  [unwired: 9 in]
        n543 = call <instrlib>:"niScope Get Session Reference.vi"("instrument handle"=w1231, "error in"=w1230) -> ("session reference"=w1224:refnum<k20>, "error out"=w1222:errorcluster)  [unwired: 11 in, 1 out]
        n544 = call "Digitizer2_FGV.vi"("error in (no error)"=w1222) -> ("error out"=w1228:errorcluster, "Read data"=w1229:refnum<k15>)  [unwired: 9 in]
        n545 = call <instrlib>:"niScope Get Session Reference.vi"("instrument handle"=w1229, "error in"=w1228) -> ("session reference"=w1223:refnum<k20>, "error out"=w1221:errorcluster)  [unwired: 11 in, 1 out]
        n546 = Build Array(w1224, w1223) -> (w1227:refnum<k20>[])
        n547 = call <instrlib>:"niTClk Configure For Homogeneous Triggers.vi"("error in (no error)"=w1221, "sessions"=w1227) -> ("error out"=w1226:errorcluster, "sessions out"=w1225:refnum<k20>[])  [unwired: 8 in]
        n548 = call <instrlib>:"niTClk Synchronize.vi"("error in (no error)"=w1226, "sessions"=w1225) -> ("error out"=w1219:errorcluster, "sessions out"=w1217:refnum<k20>[])  [unwired: 8 in]
        n549 = call <userlib>:"Wait (ms)__ogtk.vi"("error in (no error)"=w1219, "milliseconds to wait"=u32 1500) -> ("error out"=w1215:errorcluster)  [unwired: 8 in, 1 out]
        n550 = Unbundle By Name(w1215) -> ("status"=w1240:bool)
        n551 = Not(x=w1240) -> (.not. x?=w1239:bool)
        n552 = Bundle By Name(cluster=w1241, "System Status.Digitizer"=w1239, "niTClk sessions"=w1217) -> (w1242:T19)
        n553 = property on="Digitizer" class="Bool (strict)"(error in=w1215, "Blinking"=FALSE) -> (error out=w1233:errorcluster)  [unwired: 1 in, 1 out]
        n554 = call <vilib>:"Add State(s) to Queue__JKI_lib_State_Machine.vi"("State(s) in (\"\")"=w1251) -> ("States Out"=w1250:string)  [unwired: 14 in]
      }
      frame "Digitizer: Start" {
        # "send trigger to start acquisition loop"
        # "initilize aquisition"
        # "Start Digitizer\n(TClk start)"
        n555 = Unbundle By Name(w1271) -> ("niTClk sessions"=w1270:refnum<k20>[])
        n556 = call <instrlib>:"niTClk Initiate.vi"("error in (no error)"=w1264, "sessions"=w1270) -> ("error out"=w1266:errorcluster)  [unwired: 8 in, 1 out]
        n557 = Generate User Event(priority (normal)=usereventprio."high priority", user event=w1267, event data cluster=TRUE ("event data"), error in=w1266) -> (error out=w1265:errorcluster)  [unwired: 1 out]
        n558 = call <vilib>:"Add State(s) to Queue__JKI_lib_State_Machine.vi"("State(s) in (\"\")"=w1274) -> ("States Out"=w1273:string)  [unwired: 14 in]
      }
      frame "Digitizer: Abort" {
        # "Template Separator\n(You can make a copy of, or modify, this frame)"
        n559 = call "Digitizer1_FGV.vi"("error in (no error)"=w1278, "Operation (Read)"=enum16{"Write", "Read"}."Read" ("Operation")) -> ("error out"=w1285:errorcluster, "Read data"=w1282:refnum<k15>)  [unwired: 8 in]
        n560 = call "Digitizer2_FGV.vi"("error in (no error)"=w1278, "Operation (Read)"=enum16{"Write", "Read"}."Read" ("Operation")) -> ("error out"=w1281:errorcluster, "Read data"=w1283:refnum<k15>)  [unwired: 8 in]
        n561 = Bundle By Name(cluster=w1275, "SysRunning?"=FALSE ("System Status")) -> (w1276:T19)
        n562 = call <instrlib>:"niScope Abort.vi"("instrument handle"=w1282, "error in"=w1285) -> ("error out"=w1287:errorcluster)  [unwired: 12 in, 1 out]
        n563 = call <instrlib>:"niScope Abort.vi"("instrument handle"=w1283, "error in"=w1281) -> ("error out"=w1286:errorcluster)  [unwired: 12 in, 1 out]
        n564 = Merge Errors(w1287, w1286) -> (w1279:errorcluster)
        n565 = call <vilib>:"Add State(s) to Queue__JKI_lib_State_Machine.vi"("State(s) in (\"\")"=w1290) -> ("States Out"=w1289:string)  [unwired: 14 in]
      }
      frame "Digitizer: checkTemp" {
        w1293 = 65.0 ("y")
        w1298 = enum16{"Write", "Read"}."Read" ("Operation")
        # "Template Separator\n(You can make a copy of, or modify, this frame)"
        n566 = call "Digitizer1_FGV.vi"("Operation (Read)"=w1298) -> ("error out"=w1299:errorcluster, "Read data"=w1300:refnum<k15>)  [unwired: 9 in]
        n567 = call "Digitizer2_FGV.vi"("Operation (Read)"=w1298) -> ("error out"=w1296:errorcluster, "Read data"=w1297:refnum<k15>)  [unwired: 9 in]
        n568 = property on="Property Node" class="niScope"(reference=w1297, error in=w1296) -> ("Device Temperature"=w1294:dbl)  [unwired: 2 out]
        "Dig2 Temp" <- w1294
        n569 = property on="Property Node" class="niScope"(reference=w1300, error in=w1299) -> ("Device Temperature"=w1295:dbl)  [unwired: 2 out]
        "Dig1 Temp" <- w1295
        n570 = Greater?(x=w1295, y=w1293) -> (0:w1292:bool)
        n571 = Greater?(x=w1294, y=w1293) -> (0:w1291:bool)
        n572 = case shown="True" w1292 {
          frame False {
          }
          frame True {
            n573 = One Button Dialog(message="Digitizer 1 over heating!", button name ("OK")="OK") -> ()  [unwired: 1 out]
          }
        }
        n574 = case shown="True" w1291 {
          frame False {
          }
          frame True {
            n575 = One Button Dialog(message="Digitizer 2 over heating!", button name ("OK")="OK") -> ()  [unwired: 1 out]
          }
        }
        n576 = call <vilib>:"Add State(s) to Queue__JKI_lib_State_Machine.vi"("State(s) in (\"\")"=w1305) -> ("States Out"=w1304:string)  [unwired: 14 in]
      }
      frame "Digitizer: ClearError" {
        # "Template Separator\n(You can make a copy of, or modify, this frame)"
        n577 = local write "aquisition loop Error Out"(errorcluster {"status"=FALSE, "code"=0, "source"=""} ("error in (no error)")) -> ()
        n578 = call <vilib>:"Add State(s) to Queue__JKI_lib_State_Machine.vi"("State(s) in (\"\")"=w1315) -> ("States Out"=w1314:string)  [unwired: 14 in]
      }
      frame "Digitizer: Close" {
        # "Close Digitizer"
        n579 = call "Digitizer1_FGV.vi"("error in (no error)"=w1321, "Operation (Read)"=enum16{"Write", "Read"}."Read" ("Operation")) -> ("error out"=w1323:errorcluster, "Read data"=w1327:refnum<k15>)  [unwired: 8 in]
        n580 = call "Digitizer2_FGV.vi"("error in (no error)"=w1321, "Operation (Read)"=enum16{"Write", "Read"}."Read" ("Operation")) -> ("error out"=w1322:errorcluster, "Read data"=w1325:refnum<k15>)  [unwired: 8 in]
        n581 = call <instrlib>:"niScope Close.vi"("instrument handle"=w1327, "error in"=w1323) -> ("error out"=w1320:errorcluster)  [unwired: 13 in]
        n582 = call <instrlib>:"niScope Close.vi"("instrument handle"=w1325, "error in"=w1322) -> ("error out"=w1319:errorcluster)  [unwired: 13 in]
        n583 = Merge Errors(w1320, w1319) -> (w1318:errorcluster)
        n584 = Unbundle By Name(w1318) -> ("status"=w1317:bool)
        n585 = Bundle By Name(cluster=w1328, "System Status.Digitizer"=w1317) -> (w1329:T19)
        n586 = call <vilib>:"Add State(s) to Queue__JKI_lib_State_Machine.vi"("State(s) in (\"\")"=w1331) -> ("States Out"=w1330:string)  [unwired: 14 in]
      }
      frame "---------- LabJack ----------" {
        # "Template Separator\n(You can make a copy of, or modify, this frame)"
        n587 = call <vilib>:"Add State(s) to Queue__JKI_lib_State_Machine.vi"("State(s) in (\"\")"=w1336) -> ("States Out"=w1335:string)  [unwired: 14 in]
      }
      frame "LabJack: checkPedal" {
        # "Template Separator\n(You can make a copy of, or modify, this frame)"
        n588 = Unbundle By Name(w1337) -> ("LJ Pinout.Foot Pedal"=w1341:string)
        n589 = call "LabJack_FGV.vi"("Operation(Read)"=enum16{"Write", "Read"}."Read" ("Operation"), "error in (no error)"=w1339) -> ("error out"=w1343:errorcluster, "Read data"=w1344:i32)  [unwired: 8 in]
        n590 = call "LJM_eReadName.vi"("Handle In"=w1344, "Name"=w1341, "error in"=w1343) -> ("Value"=w1342:dbl, "error out"=w1340:errorcluster)  [unwired: 10 in, 1 out]
        n591 = case shown="1" w1342 {
          tunnel: w1337 -> [w1349 w1352]
          tunnel: [w1349 w1350] -> w1338
          frame 0, Default {
          }
          frame 1 {
            # "If Pedal pressed"
            n592 = Tick Count (ms)() -> (millisecond timer value=w1356:u32)
            n593 = Unbundle By Name(w1352) -> ("Last Trigger"=w1351:u32)
            n594 = Subtract(x=w1356, y=w1351) -> (x-y=w1355:u32)
            n595 = Greater Or Equal?(x=w1355, y=u32 2000) -> (x >= y?=w1353:bool)
            n596 = case shown="True" w1353 {
              tunnel: w1352 -> [w1357 w1358]
              tunnel: w1351 -> [_ _]
              tunnel: [w1357 w1359] -> w1350
              frame False {
              }
              frame True {
                n597 = Tick Count (ms)() -> (millisecond timer value=w1360:u32)
                n598 = Unbundle By Name(w1358) -> ("SysRunning?"=w1361:bool)
                n599 = case shown="True" w1361 {
                  frame False {
                    n600 = property on="StartButton" class="Bool (strict)"("Val(Sgnl)"=TRUE ("Value (Signaling)")) -> ()  [unwired: 2 in, 2 out]
                  }
                  frame True {
                    n601 = property on="StopButton" class="Bool (strict)"("Val(Sgnl)"=TRUE ("Value (Signaling)")) -> ()  [unwired: 2 in, 2 out]
                  }
                }
                n602 = Bundle By Name(cluster=w1358, "Last Trigger"=w1360) -> (w1359:T19)
              }
            }
          }
        }
        n603 = call <vilib>:"Add State(s) to Queue__JKI_lib_State_Machine.vi"("State(s) in (\"\")"=w1348) -> ("States Out"=w1347:string)  [unwired: 14 in]
      }
      frame "LabJack: ZeroV" {
        # "Just Zero V\nDO not update FGV and front panel\nWIll resume from last V"
        # "set bias to 0"
        # "Zero APD bias\n(You can make a copy of, or modify, this frame)"
        n604 = Unbundle By Name(w1366) -> ("LJ Pinout.Ch1 Bias"=w1371:string, "LJ Pinout.Ch2 Bias"=w1370:string, "LJ Pinout.Ch3 Bias"=w1369:string)
        n605 = Build Array(w1371, w1370, w1369) -> (w1368:string[])
        n606 = call "LabJack_FGV.vi"("Operation(Read)"=enum16{"Write", "Read"}."Read" ("Operation"), "error in (no error)"=w1365) -> ("error out"=w1372:errorcluster, "Read data"=w1373:i32)  [unwired: 8 in]
        n607 = call "LJM_eWriteNames.vi"("Handle In"=w1373, "aNames"=w1368, "aValuesIn"=dbl[] [0.0, 0.0, 0.0], "error in"=w1372) -> ("error out"=w1364:errorcluster)  [unwired: 9 in, 2 out]
        n608 = call <vilib>:"Add State(s) to Queue__JKI_lib_State_Machine.vi"("State(s) in (\"\")"=w1377) -> ("States Out"=w1376:string)  [unwired: 14 in]
      }
      frame "LabJack: SetV" {
        # "set bias to user specifid"
        # "Zero APD bias\n(You can make a copy of, or modify, this frame)"
        n609 = Unbundle By Name(w1391) -> ("LJ Pinout.Ch1 Bias"=w1395:string, "LJ Pinout.Ch2 Bias"=w1394:string, "LJ Pinout.Ch3 Bias"=w1393:string)
        n610 = call "V1FGV.vi"("Error In"=w1390, "action (write)"=enum16{"write", "read"}."read") -> ("Error Out"=w1389:errorcluster, "V1 out"=w1383:dbl)  [unwired: 8 in]
        n611 = local write "V 1"(w1383) -> ()
        n612 = call "V2FGV.vi"("Error In"=w1389, "action(write)"=enum16{"write", "read"}."read") -> ("Error Out"=w1388:errorcluster, "V2 out"=w1382:dbl)  [unwired: 8 in]
        n613 = local write "V 2"(w1382) -> ()
        n614 = Build Array(w1395, w1394, w1393) -> (w1392:string[])
        n615 = call "V3FGV.vi"("Error In"=w1388, "action(write)"=enum16{"write", "read"}."read" ("action(read)")) -> ("Error Out"=w1385:errorcluster, "V3 out"=w1381:dbl)  [unwired: 8 in]
        n616 = local write "V 3"(w1381) -> ()
        n617 = Build Array(w1383, w1382, w1381) -> (w1384:dbl[])
        n618 = call "LabJack_FGV.vi"("Operation(Read)"=enum16{"Write", "Read"}."Read" ("Operation"), "error in (no error)"=w1390) -> ("error out"=w1396:errorcluster, "Read data"=w1397:i32)  [unwired: 8 in]
        n619 = call "LJM_eWriteNames.vi"("Handle In"=w1397, "aNames"=w1392, "aValuesIn"=w1384, "error in"=w1396) -> ("error out"=w1386:errorcluster)  [unwired: 9 in, 2 out]
        n620 = Merge Errors(w1385, w1386) -> (w1387:errorcluster)
        n621 = call <vilib>:"Add State(s) to Queue__JKI_lib_State_Machine.vi"("State(s) in (\"\")"=w1401) -> ("States Out"=w1400:string)  [unwired: 14 in]
      }
      frame "LabJack: Open" {
        # "Initialize LabJack T7\nEstablish connection and initialize pins"
        n622 = call "LJ_Open.vi"("error in"=w1411, "DeviceType"="LJM_dtT7") -> ("error out"=w1408:errorcluster, "Success?"=w1409:bool, "Handle Out"=w1403:i32)  [unwired: 7 in]
        n623 = call "LabJack_FGV.vi"("Operation(Read)"=enum16{"Write", "Read"}."Write" ("Operation"), "error in (no error)"=w1408, "Write data"=w1403) -> ("error out"=w1405:errorcluster)  [unwired: 7 in, 1 out]
        n624 = Bundle By Name(cluster=w1406, "System Status.Labjack"=w1409) -> (w1410:T19)
        n625 = call <vilib>:"Add State(s) to Queue__JKI_lib_State_Machine.vi"("State(s) in (\"\")"=w1413) -> ("States Out"=w1412:string)  [unwired: 14 in]
      }
      frame "LabJack: SetDefaultSub" {
        w1433 = "_EF_ENABLE" ("string")
        # "1. Disable PWM\n2. Set all V to 0\n3. Set 355 relay to open\n4. Set LED to off"
        # "read once to set DIO to input"
        # "set all initila V to 0. Set footpedal to input. Set PWM to low. Set laser relay to open. Set LEDs to yellow."
        # "Set Labjack to correct input and output state and initial values"
        n626 = Unbundle By Name(w1430) -> ("LJ Pinout.355 PWM"=w1435:string, "LJ Pinout.AimingBeam PWM"=w1434:string, "LJ Pinout.Ch1 Bias"=w1442:string, "LJ Pinout.Ch2 Bias"=w1448:string, "LJ Pinout.Ch3 Bias"=w1447:string, "LJ Pinout.Laser Start/Stop"=w1446:string, "LJ Pinout.Red LED"=w1445:string, "LJ Pinout.Green LED"=w1444:string)
        n627 = call "V1FGV.vi"("Error In"=w1423, "action (write)"=enum16{"write", "read"}."write" ("action"), "V1 in"=0.0) -> ("Error Out"=w1424:errorcluster, "V1 out"=w1416:dbl)  [unwired: 7 in]
        n628 = call "LabJack_FGV.vi"("Operation(Read)"=enum16{"Write", "Read"}."Read" ("Operation"), "error in (no error)"=w1423) -> ("error out"=w1438:errorcluster, "Read data"=w1439:i32)  [unwired: 8 in]
        n629 = local write "V 1"(w1416) -> ()
        n630 = call "V2FGV.vi"("Error In"=w1424, "action(write)"=enum16{"write", "read"}."write" ("action"), "V2 in"=0.0) -> ("Error Out"=w1420:errorcluster, "V2 out"=w1415:dbl)  [unwired: 7 in]
        n631 = Concatenate Strings(w1435, w1433) -> (w1432:string)
        n632 = Concatenate Strings(w1434, w1433) -> (w1431:string)
        n633 = local write "V 2"(w1415) -> ()
        n634 = call "V3FGV.vi"("Error In"=w1420, "action(write)"=enum16{"write", "read"}."write" ("action"), "V3 in"=0.0) -> ("Error Out"=w1417:errorcluster, "V3 out"=w1414:dbl)  [unwired: 7 in]
        n635 = Build Array(w1432, w1431, w1442, w1448, w1447, w1446, w1445, w1444) -> (w1443:string[])
        n636 = local write "V 3"(w1414) -> ()
        n637 = Unbundle By Name(w1430) -> ("LJ Pinout.Foot Pedal"=w1429:string)
        n638 = call "LJM_eWriteNames.vi"("Handle In"=w1439, "aNames"=w1443, "aValuesIn"=dbl[] [0.0, 0.0, 0.0, 0.0, 0.0, 0.0, 0.0, 0.0], "error in"=w1438) -> ("Handle Out"=w1437:i32, "error out"=w1436:errorcluster)  [unwired: 9 in, 1 out]
        n639 = call "LJM_eReadName.vi"("Handle In"=w1437, "Name"=w1429, "error in"=w1436) -> ("error out"=w1419:errorcluster)  [unwired: 10 in, 2 out]
        n640 = Merge Errors(w1419, w1417) -> (w1418:errorcluster)
        n641 = call <vilib>:"Add State(s) to Queue__JKI_lib_State_Machine.vi"("State(s) in (\"\")"=w1451) -> ("States Out"=w1450:string)  [unwired: 14 in]
      }
      frame "LabJack: FootPedalConfig" {
        # "Setup footPedal\n(You can make a copy of, or modify, this frame)"
        n642 = call "LabJack_FGV.vi"("Operation(Read)"=enum16{"Write", "Read"}."Read" ("Operation"), "error in (no error)"=w1453) -> ("error out"=w1457:errorcluster, "Read data"=w1458:i32)  [unwired: 8 in]
        n643 = call "LJM_eWriteName.vi"("Handle In"=w1458, "Name"="DIO15", "Value"=1.0, "error in"=w1457) -> ("error out"=w1454:errorcluster)  [unwired: 10 in, 1 out]
        n644 = call <vilib>:"Add State(s) to Queue__JKI_lib_State_Machine.vi"("State(s) in (\"\")"=w1462) -> ("States Out"=w1461:string)  [unwired: 14 in]
      }
      frame "LabJack: SetDefaultAndClose" {
        # "Template Separator\n(You can make a copy of, or modify, this frame)"
        n645 = call <vilib>:"Add State(s) to Queue__JKI_lib_State_Machine.vi"("State(s) in Front (\"\")"="LabJack: SetDefaultSub\nLabJack: Close" ("State(s) in Front (\"\")"), "State(s) in (\"\")"=w1468) -> ("States Out"=w1467:string)  [unwired: 13 in]
      }
      frame "LabJack: Close" {
        # "Close LabJack Refnum"
        n646 = call "LabJack_FGV.vi"("Operation(Read)"=enum16{"Write", "Read"}."Read" ("Operation"), "error in (no error)"=w1474) -> ("error out"=w1469:errorcluster, "Read data"=w1470:i32)  [unwired: 8 in]
        n647 = Bundle By Name(cluster=w1472, "System Status.Labjack"=FALSE ("System Status.Gain Control")) -> (w1475:T19)
        n648 = call "LJM_Close.vi"("error in"=w1469, "Handle"=w1470) -> ("error out"=w1477:errorcluster)  [unwired: 9 in]
        n649 = call <vilib>:"Add State(s) to Queue__JKI_lib_State_Machine.vi"("State(s) in (\"\")"=w1479) -> ("States Out"=w1478:string)  [unwired: 14 in]
      }
      frame "LabJack: Interlock enable/disable" {
        w1488 = i8 0  # int8
        # "[Covers: REQ8]"
        # "Interlock enable/disable\n(Usage: \"LabJack: Interlock enable/disable >> 1|0\")"
        n650 = Fract/Exp String To Number(string=w1489, default (0 dbl)=w1488) -> (number=w1485:i8)  [unwired: 2 in, 1 out]
        n651 = Unbundle By Name(w1487) -> ("LJ Pinout.Interlock"=w1486:string)
        n652 = call "LabJack_FGV.vi"("Operation(Read)"=enum16{"Write", "Read"}."Read" ("Operation")) -> ("Read data"=w1483:i32)  [unwired: 9 in, 1 out]
        n653 = call "LJM_eWriteName.vi"("Handle In"=w1483, "Name"=w1486, "Value"=w1485, "error in"=w1484) -> ("error out"=w1481:errorcluster)  [unwired: 10 in, 1 out]
        n654 = call <vilib>:"Add State(s) to Queue__JKI_lib_State_Machine.vi"("State(s) in (\"\")"=w1491) -> ("States Out"=w1490:string)  [unwired: 14 in]
      }
      frame "LabJack: 355_PWM_Config" {
        w1493 = 0.0 ("element")
        w1513 = "DIO_EF_CLOCK1_ENABLE"
        # "Config PWM frequency"
        n655 = Unbundle By Name(w1505) -> ("LJ Pinout.355 PWM"=w1512:string)
        n656 = Unbundle By Name(w1505) -> ("355 PWM setting.DIO_EF_CLOCK1_DIVISOR"=w1504:i16, "355 PWM setting.DIO_EF_CLOCK1_ROLL_VALUE"=w1503:i32, "355 PWM setting.DIO#_EF_INDEX"=w1500:i16, "355 PWM setting.DIO#_EF_OPTIONS"=w1499:i16, "355 PWM setting.DIO#_EF_CONFIG_A"=w1498:i32)
        n657 = Concatenate Strings(w1512, "_EF_ENABLE" ("string")) -> (w1508:string)
        n658 = Concatenate Strings(w1512, "_EF_INDEX") -> (w1511:string)
        n659 = Concatenate Strings(w1512, "_EF_OPTIONS") -> (w1510:string)
        n660 = Concatenate Strings(w1512, "_EF_CONFIG_A") -> (w1509:string)
        n661 = call "LabJack_FGV.vi"("Operation(Read)"=enum16{"Write", "Read"}."Read" ("Operation")) -> ("Read data"=w1506:i32)  [unwired: 9 in, 1 out]
        n662 = Build Array(w1493, w1493, w1504, w1503, 1.0 ("element"), 0.0 ("element"), w1500, w1499, w1498) -> (w1497:dbl[])
        n663 = Build Array("DIO_EF_CLOCK0_ENABLE", w1513, "DIO_EF_CLOCK1_DIVISOR", "DIO_EF_CLOCK1_ROLL_VALUE", w1513, w1508, w1511, w1510, w1509) -> (w1507:string[])
        n664 = call "LJM_eWriteNames.vi"("Handle In"=w1506, "aNames"=w1507, "aValuesIn"=w1497, "error in"=w1495) -> ("error out"=w1496:errorcluster)  [unwired: 9 in, 2 out]
        n665 = call <vilib>:"Add State(s) to Queue__JKI_lib_State_Machine.vi"("State(s) in (\"\")"=w1522) -> ("States Out"=w1521:string)  [unwired: 14 in]
      }
      frame "LabJack: 355_PWM_Start" {
        # "Template Separator\n(You can make a copy of, or modify, this frame)"
        n666 = Unbundle By Name(w1530) -> ("LJ Pinout.355 PWM"=w1529:string)
        n667 = call "LabJack_FGV.vi"("Operation(Read)"=enum16{"Write", "Read"}."Read" ("Operation"), "error in (no error)"=w1524) -> ("error out"=w1531:errorcluster, "Read data"=w1532:i32)  [unwired: 8 in]
        n668 = Concatenate Strings(w1529, "_EF_ENABLE" ("string")) -> (w1527:string)
        n669 = call "LJM_eWriteName.vi"("Handle In"=w1532, "Name"=w1527, "Value"=1.0, "error in"=w1531) -> ("error out"=w1525:errorcluster)  [unwired: 10 in, 1 out]
        n670 = call <vilib>:"Add State(s) to Queue__JKI_lib_State_Machine.vi"("State(s) in (\"\")"=w1535) -> ("States Out"=w1534:string)  [unwired: 14 in]
      }
      frame "LabJack: 355_PWM_Stop" {
        # "Template Separator\n(You can make a copy of, or modify, this frame)"
        n671 = Unbundle By Name(w1541) -> ("LJ Pinout.355 PWM"=w1545:string)
        n672 = call "LabJack_FGV.vi"("Operation(Read)"=enum16{"Write", "Read"}."Read" ("Operation"), "error in (no error)"=w1540) -> ("error out"=w1546:errorcluster, "Read data"=w1538:i32)  [unwired: 8 in]
        n673 = Concatenate Strings(w1545, "_EF_ENABLE" ("string")) -> (w1543:string)
        n674 = call "LJM_eWriteName.vi"("Handle In"=w1538, "Name"=w1543, "Value"=0.0, "error in"=w1546) -> ("error out"=w1537:errorcluster)  [unwired: 10 in, 1 out]
        n675 = local write "355nm Laser toggle"(FALSE ("355nm Laser toggle")) -> ()
        n676 = call <vilib>:"Add State(s) to Queue__JKI_lib_State_Machine.vi"("State(s) in (\"\")"=w1549) -> ("States Out"=w1548:string)  [unwired: 14 in]
      }
      frame "LabJack: AB_Start" {
        # "Aiming Beam Start\n(Based on aimging beam frequency, set LabJack pin)"
        n677 = Unbundle By Name(w1559) -> ("AB Cluster.Freq"=w1551:i32, "LJ Pinout.AimingBeam PWM"=w1558:string)
        n678 = Greater Than 0?(x=w1551) -> (x > 0?=w1550:bool)
        n679 = case shown="False" w1550 {
          tunnel: w1558 -> [w1565 w1568]
          tunnel: [w1565 w1566] -> w1557
          frame False {
            # "if 0 freq, set PWM pin"
          }
          frame True {
            # "if non zero freq, set PWM enable"
            n680 = Concatenate Strings(w1568, "_EF_ENABLE" ("string")) -> (w1566:string)
          }
        }
        n681 = call "LabJack_FGV.vi"("Operation(Read)"=enum16{"Write", "Read"}."Read" ("Operation"), "error in (no error)"=w1554) -> ("error out"=w1560:errorcluster, "Read data"=w1561:i32)  [unwired: 8 in]
        n682 = call "LJM_eWriteName.vi"("Handle In"=w1561, "Name"=w1557, "Value"=1.0, "error in"=w1560) -> ("error out"=w1555:errorcluster)  [unwired: 10 in, 1 out]
        n683 = local write "Aiming beam toggle"(TRUE ("Aiming beam toggle")) -> ()
        n684 = call <vilib>:"Add State(s) to Queue__JKI_lib_State_Machine.vi"("State(s) in (\"\")"=w1564) -> ("States Out"=w1563:string)  [unwired: 14 in]
      }
      frame "LabJack: AB_Stop" {
        # "Aiming Beam Stop\n(Based on aiming beam frequency, set LabJack pin low)"
        n685 = Unbundle By Name(w1576) -> ("AB Cluster.Freq"=w1571:i32, "LJ Pinout.AimingBeam PWM"=w1578:string)
        n686 = Greater Than 0?(x=w1571) -> (x > 0?=w1570:bool)
        n687 = case shown="False" w1570 {
          tunnel: w1578 -> [w1584 w1587]
          tunnel: [w1584 w1585] -> w1569
          frame False {
          }
          frame True {
            n688 = Concatenate Strings(w1587, "_EF_ENABLE" ("string")) -> (w1585:string)
          }
        }
        n689 = call "LabJack_FGV.vi"("Operation(Read)"=enum16{"Write", "Read"}."Read" ("Operation"), "error in (no error)"=w1574) -> ("error out"=w1579:errorcluster, "Read data"=w1580:i32)  [unwired: 8 in]
        n690 = call "LJM_eWriteName.vi"("Handle In"=w1580, "Name"=w1569, "Value"=0.0, "error in"=w1579) -> ("error out"=w1575:errorcluster)  [unwired: 10 in, 1 out]
        n691 = local write "Aiming beam toggle"(FALSE ("Aiming beam toggle")) -> ()
        n692 = call <vilib>:"Add State(s) to Queue__JKI_lib_State_Machine.vi"("State(s) in (\"\")"=w1583) -> ("States Out"=w1582:string)  [unwired: 14 in]
      }
      frame "LabJack: AB_PWM_Config" {
        w1589 = 0.0 ("element")
        w1609 = "DIO_EF_CLOCK2_ENABLE"
        # "Config PWM frequency"
        n693 = Unbundle By Name(w1601) -> ("LJ Pinout.AimingBeam PWM"=w1608:string)
        n694 = Unbundle By Name(w1601) -> ("AB PWM setting.DIO_EF_CLOCK1_DIVISOR"=w1600:i16, "AB PWM setting.DIO_EF_CLOCK1_ROLL_VALUE"=w1599:i32, "AB PWM setting.DIO#_EF_INDEX"=w1596:i16, "AB PWM setting.DIO#_EF_OPTIONS"=w1595:i16, "AB PWM setting.DIO#_EF_CONFIG_A"=w1594:i32)
        n695 = Concatenate Strings(w1608, "_EF_ENABLE" ("string")) -> (w1604:string)
        n696 = Concatenate Strings(w1608, "_EF_INDEX") -> (w1607:string)
        n697 = Concatenate Strings(w1608, "_EF_OPTIONS") -> (w1606:string)
        n698 = Concatenate Strings(w1608, "_EF_CONFIG_A") -> (w1605:string)
        n699 = call "LabJack_FGV.vi"("Operation(Read)"=enum16{"Write", "Read"}."Read" ("Operation")) -> ("Read data"=w1602:i32)  [unwired: 9 in, 1 out]
        n700 = Build Array(w1589, w1589, w1600, w1599, 1.0 ("element"), 0.0 ("element"), w1596, w1595, w1594) -> (w1593:dbl[])
        n701 = Build Array("DIO_EF_CLOCK0_ENABLE", w1609, "DIO_EF_CLOCK2_DIVISOR", "DIO_EF_CLOCK2_ROLL_VALUE", w1609, w1604, w1607, w1606, w1605) -> (w1603:string[])
        n702 = call "LJM_eWriteNames.vi"("Handle In"=w1602, "aNames"=w1603, "aValuesIn"=w1593, "error in"=w1591) -> ("error out"=w1592:errorcluster)  [unwired: 9 in, 2 out]
        n703 = call <vilib>:"Add State(s) to Queue__JKI_lib_State_Machine.vi"("State(s) in (\"\")"=w1618) -> ("States Out"=w1617:string)  [unwired: 14 in]
      }
      frame "---------- LED ----------" {
        # "Template Separator\n(You can make a copy of, or modify, this frame)"
        n704 = call <vilib>:"Add State(s) to Queue__JKI_lib_State_Machine.vi"("State(s) in (\"\")"=w1623) -> ("States Out"=w1622:string)  [unwired: 14 in]
      }
      frame "LED: OpenVIRef" {
        # "Template Separator\n(You can make a copy of, or modify, this frame)"
        n705 = call <vilib>:"Application Directory.vi"() -> ("Application Directory"=w1630:path)
        n706 = Build Path(base path=w1630, name or relative path="SubVI") -> (appended path=w1628:path)
        n707 = Build Path(base path=w1628, name or relative path="LEDBreath.vi") -> (appended path=w1626:path)
        n708 = Open VI Reference(vi path=w1626, error in (no error)=w1631) -> (vi reference=w1632:refnum<vi>, error out=w1625:errorcluster)  [unwired: 4 in]
        n709 = case shown="Error .." w1625 {
          tunnel: [TRUE FALSE] -> w1624
          frame No Error {
          }
          frame Error {
          }
        }
        n710 = Bundle By Name(cluster=w1633, "LED vi reference"=w1632, "LED vi ref open?"=w1624) -> (w1634:T19)
        n711 = call <vilib>:"Add State(s) to Queue__JKI_lib_State_Machine.vi"("State(s) in (\"\")"=w1637) -> ("States Out"=w1636:string)  [unwired: 14 in]
      }
      frame "LED: CloseVIRef" {
        # "Template Separator\n(You can make a copy of, or modify, this frame)"
        n712 = Unbundle By Name(w1641) -> ("LED vi reference"=w1642:refnum<vi>, "LED vi ref open?"=w1640:bool)
        n713 = case shown="True" w1640 {
          tunnel: w1644 -> [w1648 w1651]
          tunnel: [w1648 w1650] -> w1643
          tunnel: w1642 -> [_ w1649]
          frame False {
          }
          frame True {
            n714 = Close Reference(reference=w1649, error in (no error)=w1651) -> (error out=w1650:errorcluster)
          }
        }
        n715 = call <vilib>:"Add State(s) to Queue__JKI_lib_State_Machine.vi"("State(s) in (\"\")"=w1647) -> ("States Out"=w1646:string)  [unwired: 14 in]
      }
      frame "LED: BreathGreen" {
        w1652 = FALSE ("Wait Until Done")
        # "Breath system LED\n(LED: Breath >> True/False)"
        n716 = Unbundle By Name(w1660) -> ("LED vi reference"=w1659:refnum<vi>)
        n717 = invoke class="VI" method="Ctrl Val.Set"(reference=w1659, error in=w1657, "Control Name"="Color", "Value"=0) -> (reference out=w1656:refnum<vi>, error out=w1655:errorcluster)  [unwired: 1 in, 3 out]
        n718 = invoke on="Invoke Node" class="VI" method="Run VI"(reference=w1656, error in=w1655, "Wait until done"=w1652, "Auto Dispose Ref"=w1652) -> (error out=w1658:errorcluster)  [unwired: 1 in, 4 out]
        n719 = call <vilib>:"Add State(s) to Queue__JKI_lib_State_Machine.vi"("State(s) in (\"\")"=w1663) -> ("States Out"=w1662:string)  [unwired: 14 in]
      }
      frame "LED: BreathOrange" {
        w1664 = FALSE ("Wait Until Done")
        # "Breath system LED\n(LED: Breath >> True/False)"
        n720 = Unbundle By Name(w1672) -> ("LED vi reference"=w1671:refnum<vi>)
        n721 = invoke class="VI" method="Ctrl Val.Set"(reference=w1671, error in=w1669, "Control Name"="Color", "Value"=1) -> (reference out=w1668:refnum<vi>, error out=w1667:errorcluster)  [unwired: 1 in, 3 out]
        n722 = invoke on="Invoke Node" class="VI" method="Run VI"(reference=w1668, error in=w1667, "Wait until done"=w1664, "Auto Dispose Ref"=w1664) -> (error out=w1670:errorcluster)  [unwired: 1 in, 4 out]
        n723 = call <vilib>:"Add State(s) to Queue__JKI_lib_State_Machine.vi"("State(s) in (\"\")"=w1675) -> ("States Out"=w1674:string)  [unwired: 14 in]
      }
      frame "LED: BreathOff" {
        # "System LED Breath Off\n(Breath off, check VI status to make sure it is off)"
        n724 = Unbundle By Name(w1684) -> ("LED vi reference"=w1683:refnum<vi>)
        n725 = invoke on="Invoke Node" class="VI" method="Ctrl Val.Set"(reference=w1683, error in=w1681, "Control Name"="Stop", "Value"=TRUE) -> (reference out=w1676:refnum<vi>, error out=w1677:errorcluster)  [unwired: 1 in, 3 out]
        n726 = case shown="No Error" w1677 {
          selector: w1677 -> [w1689 _]
          tunnel: [w1688 errorcluster {"status"=FALSE, "code"=0, "source"=""} ("error IO")] -> w1682
          tunnel: ["" ("State(s) in Front (\"\")") "LED: BreathOff" ("State(s) in Front (\"\")")] -> w1680
          tunnel: w1676 -> [w1690 _]
          frame No Error {
            # "No error, wait for VI to stop"
            n727 = while {
              tunnel: w1690 -> [w1698]
              shift-right: [w1692] -> w1688
              shift-left: w1689 -> [w1697]
              stop <- w1694 stop-if-true
              # "continue check whether vi is running"
              n728 = property class="VI"(reference=w1698, error in=w1697) -> (error out=w1692:errorcluster, "Exec.State"=w1696:T16)  [unwired: 1 out]
              n729 = Wait (ms)(milliseconds to wait=u32 50) -> ()  [unwired: 1 out]
              n730 = Equal?(x=w1696, y=T16."Idle") -> (x = y?=w1694:bool)
            }
          }
          frame Error {
            # "try again when error"
          }
        }
        n731 = call <vilib>:"Add State(s) to Queue__JKI_lib_State_Machine.vi"("State(s) in Front (\"\")"=w1680, "State(s) in (\"\")"=w1687) -> ("States Out"=w1686:string)  [unwired: 13 in]
      }
      frame "LED: Off" {
        # "set LED to red"
        # "Template Separator\n(You can make a copy of, or modify, this frame)"
        n732 = Unbundle By Name(w1703) -> ("LJ Pinout.Red LED"=w1702:string, "LJ Pinout.Green LED"=w1701:string)
        n733 = call "LabJack_FGV.vi"("Operation(Read)"=enum16{"Write", "Read"}."Read" ("Operation"), "error in (no error)"=w1704) -> ("error out"=w1711:errorcluster, "Read data"=w1710:i32)  [unwired: 8 in]
        n734 = call "LJM_eWriteName.vi"("Handle In"=w1710, "Name"=w1702, "Value"=0.0, "error in"=w1711) -> ("Handle Out"=w1708:i32, "error out"=w1707:errorcluster)  [unwired: 10 in]
        n735 = call "LJM_eWriteName.vi"("Handle In"=w1708, "Name"=w1701, "Value"=0.0, "error in"=w1707) -> ("error out"=w1705:errorcluster)  [unwired: 10 in, 1 out]
        n736 = call <vilib>:"Add State(s) to Queue__JKI_lib_State_Machine.vi"("State(s) in (\"\")"=w1715) -> ("States Out"=w1714:string)  [unwired: 14 in]
      }
      frame "LED: Green" {
        # "set LED to green"
        # "Template Separator\n(You can make a copy of, or modify, this frame)"
        n737 = Unbundle By Name(w1719) -> ("LJ Pinout.Red LED"=w1717:string, "LJ Pinout.Green LED"=w1718:string)
        n738 = call "LabJack_FGV.vi"("Operation(Read)"=enum16{"Write", "Read"}."Read" ("Operation"), "error in (no error)"=w1721) -> ("error out"=w1727:errorcluster, "Read data"=w1726:i32)  [unwired: 8 in]
        n739 = call "LJM_eWriteName.vi"("Handle In"=w1726, "Name"=w1717, "Value"=0.0, "error in"=w1727) -> ("Handle Out"=w1724:i32, "error out"=w1723:errorcluster)  [unwired: 10 in]
        n740 = call "LJM_eWriteName.vi"("Handle In"=w1724, "Name"=w1718, "Value"=9.0, "error in"=w1723) -> ("error out"=w1720:errorcluster)  [unwired: 10 in, 1 out]
        n741 = call <vilib>:"Add State(s) to Queue__JKI_lib_State_Machine.vi"("State(s) in (\"\")"=w1730) -> ("States Out"=w1729:string)  [unwired: 14 in]
      }
      frame "---------- Queue ----------" {
        # "Template Separator\n(You can make a copy of, or modify, this frame)"
        n742 = call <vilib>:"Add State(s) to Queue__JKI_lib_State_Machine.vi"("State(s) in (\"\")"=w1735) -> ("States Out"=w1734:string)  [unwired: 14 in]
      }
      frame "Queue: Flash" {
        # "Clear queue contnet\n(clear queue content by flash it)"
        n743 = Flush Queue(queue=w1741, error in (no error)=w1740) -> (error out=w1739:errorcluster)  [unwired: 2 out]
        n744 = Flush Queue(queue=w1742, error in (no error)=w1739) -> (error out=w1737:errorcluster)  [unwired: 2 out]
        n745 = Flush Queue(queue=w1738, error in (no error)=w1737) -> (error out=w1736:errorcluster)  [unwired: 2 out]
        n746 = call <vilib>:"Add State(s) to Queue__JKI_lib_State_Machine.vi"("State(s) in (\"\")"=w1746) -> ("States Out"=w1745:string)  [unwired: 14 in]
      }
      frame "Queue: Destory" {
        # "Destory Data Queue\nDistory data queue ref so the aquisition loop stop"
        n747 = Release Queue(queue=w1752, error in (no error)=w1748) -> (error out=w1755:errorcluster)  [unwired: 1 in, 2 out]
        n748 = Release Queue(queue=w1751, error in (no error)=w1748) -> (error out=w1754:errorcluster)  [unwired: 1 in, 2 out]
        n749 = Release Queue(queue=w1749, error in (no error)=w1748) -> (error out=w1747:errorcluster)  [unwired: 1 in, 2 out]
        n750 = Merge Errors(w1755, w1754, w1747) -> (w1753:errorcluster)
        n751 = call <vilib>:"Simple Error Handler.vi"("error in (no error)"=w1753) -> ()  [unwired: 4 in, 5 out]
        n752 = call <vilib>:"Add State(s) to Queue__JKI_lib_State_Machine.vi"("State(s) in (\"\")"=w1758) -> ("States Out"=w1757:string)  [unwired: 14 in]
      }
      frame "---------- Run ----------" {
        # "Template Separator\n(You can make a copy of, or modify, this frame)"
        n753 = call <vilib>:"Add State(s) to Queue__JKI_lib_State_Machine.vi"("State(s) in (\"\")"=w1763) -> ("States Out"=w1762:string)  [unwired: 14 in]
      }
      frame "Run: CaliIncrement" {
        # "Increment Calibration #\n(You can make a copy of, or modify, this frame)"
        n754 = Unbundle By Name(w1765) -> ("IDs.Cali ID"=w1767:i8)
        n755 = Increment(x=w1767) -> (x+1=w1764:i8)
        n756 = Bundle By Name(cluster=w1765, "IDs.Cali ID"=w1764) -> (w1766:T19)
        n757 = call <vilib>:"Add State(s) to Queue__JKI_lib_State_Machine.vi"("State(s) in (\"\")"=w1771) -> ("States Out"=w1770:string)  [unwired: 14 in]
      }
      frame "Run: BGIncrement" {
        # "Increment BG #\n(You can make a copy of, or modify, this frame)"
        n758 = Unbundle By Name(w1772) -> ("IDs.BG ID"=w1775:i8)
        n759 = Increment(x=w1775) -> (x+1=w1774:i8)
        n760 = Bundle By Name(cluster=w1772, "IDs.BG ID"=w1774) -> (w1773:T19)
        n761 = call <vilib>:"Add State(s) to Queue__JKI_lib_State_Machine.vi"("State(s) in (\"\")"=w1779) -> ("States Out"=w1778:string)  [unwired: 14 in]
      }
      frame "Run: Increment" {
        # "Increase Run# by 1"
        n762 = Unbundle By Name(w1784) -> ("IDs.RunID"=w1786:i8)
        n763 = Increment(x=w1786) -> (x+1=w1782:i8)
        n764 = Bundle By Name(cluster=w1784, "IDs.RunID"=w1782) -> (w1785:T19)
        n765 = call "RunIDFGV.vi"("Error In"=w1780, "RunID in"=w1782) -> ("Error Out"=w1781:errorcluster)  [unwired: 8 in, 1 out]
        n766 = call <vilib>:"Add State(s) to Queue__JKI_lib_State_Machine.vi"("State(s) in (\"\")"=w1788) -> ("States Out"=w1787:string)  [unwired: 14 in]
      }
      frame "Run: Decrement" {
        # "Increase Run# by 1"
        n767 = Unbundle By Name(w1793) -> ("IDs.RunID"=w1795:i8)
        n768 = Decrement(x=w1795) -> (x-1=w1791:i8)
        n769 = Bundle By Name(cluster=w1793, "IDs.RunID"=w1791) -> (w1794:T19)
        n770 = call "RunIDFGV.vi"("Error In"=w1789, "RunID in"=w1791) -> ("Error Out"=w1790:errorcluster)  [unwired: 8 in, 1 out]
        n771 = call <vilib>:"Add State(s) to Queue__JKI_lib_State_Machine.vi"("State(s) in (\"\")"=w1797) -> ("States Out"=w1796:string)  [unwired: 14 in]
      }
      frame "---------- SysConfig ----------" {
        # "Template Separator\n(You can make a copy of, or modify, this frame)"
        n772 = call <vilib>:"Add State(s) to Queue__JKI_lib_State_Machine.vi"("State(s) in (\"\")"=w1802) -> ("States Out"=w1801:string)  [unwired: 14 in]
      }
      frame "SysConfig: LoadAPDSerialNumber" {
        # "Template Separator\n(You can make a copy of, or modify, this frame)"
        n773 = call "readAPDSerial.vi"("Error In"=w1804) -> ("Error Out"=w1803:errorcluster, "output cluster"=w1805:T35)  [unwired: 9 in]
        n774 = Bundle By Name(cluster=w1806, "APDSerialNum"=w1805) -> (w1807:T19)
        n775 = call <vilib>:"Add State(s) to Queue__JKI_lib_State_Machine.vi"("State(s) in (\"\")"=w1810) -> ("States Out"=w1809:string)  [unwired: 14 in]
      }
      frame "SysConfig: Load Sys Config" {
        # "[Covers: REQ5]"
        # "Load System config"
        # "Load system configuration\n(Load both hardware and DAQ config)"
        n776 = call "LoadSysConfig.vi"("Error In"=w1813, "Enum"=enum16{"LastUse", "Default"}."LastUse") -> ("Error Out"=w1812:errorcluster, "SysConfigCluster"=w1815:T4)  [unwired: 8 in]
        "SysConfigCluster" <- w1815
        n777 = Bundle By Name(cluster=w1816, "SysConfigCluster"=w1815) -> (w1817:T19)
        n778 = call <vilib>:"Add State(s) to Queue__JKI_lib_State_Machine.vi"("State(s) in (\"\")"=w1819) -> ("States Out"=w1818:string)  [unwired: 14 in]
      }
      frame "SysConfig: Load Digitizer Setting" {
        w1820 = enum16{"Write", "Read"}."Write" ("Operation")
        # "Load DAQ config\nSave to FGV"
        # "Template Separator\n(You can make a copy of, or modify, this frame)"
        n779 = call <userlib>:"Current VIs Parent Directory__ogtk.vi"() -> ("Parent Directory (+ Relative)"=w1834:path)  [unwired: 5 in]
        n780 = Build Path(base path=w1834, name or relative path="SubVI\\DigitizerConfiguration\\V6_Scope_HR_Scan.config") -> (appended path=w1835:path)
        n781 = call "ReadDigitizerConfig(SubVI).vi"("error in (no error)"=w1832, "appended path"=w1835) -> ("error out"=w1828:errorcluster, "FLImDAQ"=w1826:T6)  [unwired: 8 in]
        n782 = call "FLImDAQ_FGV.vi"("error in (no error)"=w1828, "Operation (Read)"=w1820, "Write data"=w1826) -> ("error out"=w1830:errorcluster)  [unwired: 7 in, 1 out]
        n783 = Unbundle By Name(w1826) -> ("min record length"=→"data length":i32, "Digitizer 1"=w1822:refnum<k15>, "Digitizer 2"=w1829:refnum<k15>)
        n784 = Bundle By Name(cluster=w1824, "FLImDAQ"=w1826) -> (w1825:T19)
        n785 = call "Digitizer1_FGV.vi"("error in (no error)"=w1830, "Operation (Read)"=w1820, "Write data"=w1822) -> ("error out"=w1831:errorcluster)  [unwired: 7 in, 1 out]
        n786 = call "Digitizer2_FGV.vi"("error in (no error)"=w1831, "Operation (Read)"=w1820, "Write data"=w1829) -> ("error out"=w1827:errorcluster)  [unwired: 7 in, 1 out]
        n787 = call <vilib>:"Add State(s) to Queue__JKI_lib_State_Machine.vi"("State(s) in (\"\")"=w1837) -> ("States Out"=w1836:string)  [unwired: 14 in]
      }
      frame "SysConfig: Load LJ Pinout" {
        # "Template Separator\n(You can make a copy of, or modify, this frame)"
        n788 = call <userlib>:"Current VIs Parent Directory__ogtk.vi"() -> ("Parent Directory (+ Relative)"=w1851:path)  [unwired: 5 in]
        n789 = Build Path(base path=w1851, name or relative path="SubVI\\LabJack\\LJ_pin_setting.config") -> (appended path=w1849:path)
        n790 = call "ReadLabjackConfig(SubVI).vi"("error in (no error)"=w1847, "appended path"=w1849) -> ("error out"=w1848:errorcluster, "Utility"=w1845:T5)  [unwired: 8 in]
        n791 = Unbundle By Name(w1845) -> ("Ch1 Bias"=w1844:string, "Ch2 Bias"=w1843:string, "Ch3 Bias"=w1842:string, "Red LED"=w1839:string, "Green LED"=w1838:string)
        n792 = global write "GlobalVariables.vi" "LED Green pin"(w1838) -> ()
        n793 = global write "GlobalVariables.vi" "LED Red pin"(w1839) -> ()
        n794 = global write "GlobalVariables.vi" "Ch1 LJ pin"(w1844) -> ()
        n795 = global write "GlobalVariables.vi" "Ch2 LJ pin"(w1843) -> ()
        n796 = global write "GlobalVariables.vi" "Ch3 LJ pin"(w1842) -> ()
        n797 = Bundle By Name(cluster=w1840, "LJ Pinout"=w1845) -> (w1846:T19)
        n798 = call <vilib>:"Add State(s) to Queue__JKI_lib_State_Machine.vi"("State(s) in (\"\")"=w1853) -> ("States Out"=w1852:string)  [unwired: 14 in]
      }
      frame "SysConfig: Load 355 PWM" {
        # "Template Separator\n(You can make a copy of, or modify, this frame)"
        n799 = call <userlib>:"Current VIs Parent Directory__ogtk.vi"() -> ("Parent Directory (+ Relative)"=w1871:path)  [unwired: 5 in]
        n800 = Build Path(base path=w1871, name or relative path="SubVI\\LabJack\\PWM_setting_355.config") -> (appended path=w1869:path)
        n801 = call "ReadPWMConfig(SubVI).vi"("error in (no error)"=w1866, "appended path"=w1869) -> ("error out"=w1867:errorcluster, "PWM Setting"=w1865:T36)  [unwired: 8 in]
        n802 = Unbundle By Name(w1865) -> ("DIO_EF_CLOCK1_DIVISOR"=w1862:i16, "DIO_EF_CLOCK1_ROLL_VALUE"=w1861:i32)
        n803 = Multiply(x=w1862, y=w1861) -> (x*y=w1863:i32)
        n804 = Bundle By Name(cluster=w1868, "355 PWM setting"=w1865) -> (w1855:T19)
        n805 = Divide(x=80000000.0, y=w1863) -> (x/y=w1860:dbl)
        "Laser Rep Rate" <- w1860
        n806 = Number To Decimal String(number=w1860) -> (decimal integer string=w1859:string)  [unwired: 1 in]
        n807 = Concatenate Strings("355nm " ("string"), w1859, "Hz" ("string")) -> (w1857:string)
        n808 = property on="355nm Laser toggle" class="Bool (strict)"("Caption.Text"=w1857) -> ()  [unwired: 2 in, 2 out]
        n809 = call <vilib>:"Add State(s) to Queue__JKI_lib_State_Machine.vi"("State(s) in (\"\")"=w1873) -> ("States Out"=w1872:string)  [unwired: 14 in]
      }
      frame "SysConfig: Load AB PWM" {
        # "Template Separator\n(You can make a copy of, or modify, this frame)"
        n810 = call <userlib>:"Current VIs Parent Directory__ogtk.vi"() -> ("Parent Directory (+ Relative)"=w1882:path)  [unwired: 5 in]
        n811 = Build Path(base path=w1882, name or relative path="SubVI\\LabJack\\PWM_setting_AB.config") -> (appended path=w1880:path)
        n812 = call "ReadPWMConfig(SubVI).vi"("error in (no error)"=w1877, "appended path"=w1880) -> ("error out"=w1878:errorcluster, "PWM Setting"=w1876:T36)  [unwired: 8 in]
        n813 = Bundle By Name(cluster=w1874, "AB PWM setting"=w1876) -> (w1879:T19)
        n814 = call <vilib>:"Add State(s) to Queue__JKI_lib_State_Machine.vi"("State(s) in (\"\")"=w1884) -> ("States Out"=w1883:string)  [unwired: 14 in]
      }
      frame "SysConfig: Load AB setting" {
        # "load aming beam setting\n(check frequency, if 0 do nothing, if not zero, config PWM)"
        n815 = call "readAimingBeamSetting.vi"("error in (no error)"=w1902) -> ("error out"=w1897:errorcluster, "Aiming Beam Setting"=w1889:T37)  [unwired: 9 in]
        n816 = Unbundle By Name(w1889) -> ("Default Current"=w1888:dbl)
        n817 = Unbundle By Name(w1889) -> ("Frequency(Hz)"=w1885:u32)
        n818 = Equal To 0?(x=w1885) -> (x = 0?=w1895:bool)
        n819 = Select(t="", s=w1895, f="SysConfig: Load AB PWM" ("State(s) in Front (\"\")")) -> (s? t:f=w1898:string)
        n820 = Number To Decimal String(number=w1885) -> (decimal integer string=w1894:string)  [unwired: 1 in]
        n821 = Number To Decimal String(number=w1888, width (-)=i16 2) -> (decimal integer string=w1887:string)
        n822 = Concatenate Strings("445nm " ("string"), w1894, "Hz " ("string"), w1887, "mA" ("string")) -> (w1893:string)
        n823 = property on="Aiming beam toggle" class="Bool (strict)"("Caption.Text"=w1893) -> ()  [unwired: 2 in, 2 out]
        n824 = case shown="False" w1895 {
          tunnel: w1897 -> [w1909 w1912]
          tunnel: [w1908 w1912] -> w1896
          tunnel: w1885 -> [w1907 _]
          frame False {
            n825 = call "LJ_calculate_PWM_parameters.vi"("Error In"=w1909, "Show Confirmation"=FALSE, "Laser Rep Rate (Hz)"=w1907, "Laser"=enum16{"355nm", "AimingBeam"}."AimingBeam") -> ("Error Out"=w1908:errorcluster)  [unwired: 6 in, 1 out]
          }
          frame True {
          }
        }
        n826 = Bundle By Name(cluster=w1903, "AB Cluster"=w1889) -> (w1904:T19)
        n827 = call <vilib>:"Add State(s) to Queue__JKI_lib_State_Machine.vi"("State(s) in Front (\"\")"=w1898, "State(s) in (\"\")"=w1906) -> ("States Out"=w1905:string)  [unwired: 13 in]
      }
      frame "SysConfig: LoadABVideoSetting" {
        # "Load AB video setting form ini file\n()"
        n828 = call "readVideoConfig.vi"("error in (no error)"=w1916) -> ("error out"=w1917:errorcluster, "Aiming Beam Config"=w1915:T18)  [unwired: 8 in, 1 out]
        n829 = Bundle By Name(cluster=w1913, "VideoConfig"=w1915) -> (w1914:T19)
        n830 = call <vilib>:"Add State(s) to Queue__JKI_lib_State_Machine.vi"("State(s) in (\"\")"=w1920) -> ("States Out"=w1919:string)  [unwired: 14 in]
      }
      frame "SysConfig: LoadCursorLocation" {
        # "Load cursor location from ini file\n(load cursor from system setting ini file)"
        n831 = call "readCursorConfigMain.vi"("error in (no error)"=w1932) -> ("error out"=w1933:errorcluster, "Cursor Locations"=w1931:T38)  [unwired: 9 in]
        n832 = Unbundle By Name(w1931) -> ("DC1"=w1930:i32, "DC2"=w1929:i32, "BG1"=w1924:i32, "BG2"=w1923:i32)
        n833 = Build Array(w1930, w1929) -> (w1928:i32[])
        n834 = Build Array(w1924, w1923) -> (w1925:i32[])
        n835 = Array Max & Min(array=w1928) -> (max value=w1927:i32, min value=w1926:i32)  [unwired: 2 out]
        n836 = Array Max & Min(array=w1925) -> (max value=w1922:i32, min value=w1921:i32)  [unwired: 2 out]
        n837 = global write "GlobalVariables.vi" "DC Idx2"(w1927) -> ()
        n838 = global write "GlobalVariables.vi" "DC Idx1"(w1926) -> ()
        n839 = global write "GlobalVariables.vi" "BG Idx2"(w1922) -> ()
        n840 = global write "GlobalVariables.vi" "BG Idx1"(w1921) -> ()
        n841 = call <vilib>:"Add State(s) to Queue__JKI_lib_State_Machine.vi"("State(s) in (\"\")"=w1937) -> ("States Out"=w1936:string)  [unwired: 14 in]
      }
      frame "---------- SystemStatus ----------" {
        # "Template Separator\n(You can make a copy of, or modify, this frame)"
        n842 = call <vilib>:"Add State(s) to Queue__JKI_lib_State_Machine.vi"("State(s) in (\"\")"=w1942) -> ("States Out"=w1941:string)  [unwired: 14 in]
      }
      frame "SystemStatus: SlowSysStatusMacro" {
        # "store system check time"
        # "Template Separator\n(You can make a copy of, or modify, this frame)"
        n843 = Tick Count (ms)() -> (millisecond timer value=w1945:u32)
        n844 = Bundle By Name(cluster=w1943, "SlowTimer"=w1945) -> (w1944:T19)
        n845 = call <vilib>:"Add State(s) to Queue__JKI_lib_State_Machine.vi"("State(s) in Front (\"\")"="Digitizer: checkTemp" ("State(s) in Front (\"\")"), "State(s) in (\"\")"=w1950) -> ("States Out"=w1949:string)  [unwired: 13 in]
      }
      frame "SystemStatus: FastSysStatusMacro" {
        # "store system check time"
        # "Template Separator\n(You can make a copy of, or modify, this frame)"
        n846 = Tick Count (ms)() -> (millisecond timer value=w1953:u32)
        n847 = Bundle By Name(cluster=w1951, "FastTimer"=w1953) -> (w1952:T19)
        n848 = call <vilib>:"Add State(s) to Queue__JKI_lib_State_Machine.vi"("State(s) in Front (\"\")"="355 Laser: CheckPWMStatus\nAimingBeam: GetPWMStatus\n/*355 Laser: CheckControllerStatus" ("State(s) in Front (\"\")"), "State(s) in (\"\")"=w1958) -> ("States Out"=w1957:string)  [unwired: 13 in]
      }
      frame "---------- UI ----------" {
        # "Do not put any code in this frame.\n(It is a separator no-op. You can make a copy of this frame to create a new UI frame)"
        n849 = call <vilib>:"Add State(s) to Queue__JKI_lib_State_Machine.vi"("State(s) in (\"\")"=w1963) -> ("States Out"=w1962:string)  [unwired: 14 in]
      }
      frame "UI: Initialize" {
        w1965 = T39 {"Minimum"=0.0, "Maximum"=4.7, "Increment"=0.1} ("Data Entry Limits")
        w1964 = T17."Disabled and Grayed Out" ("Disabled")
        # "Disable all button on startup"
        # "Initialize the User Interface, here.\n(this is called automatically, by the Macro: Init)"
        n850 = property on="StopButton" class="Bool (strict)"("DisabledEnum"=w1964) -> ()  [unwired: 2 in, 2 out]
        n851 = property on="Sys Reconfig" class="Bool"("DisabledEnum"=w1964) -> ()  [unwired: 2 in, 2 out]
        n852 = property on="StartButton" class="Bool (strict)"("DisabledEnum"=w1964) -> ()  [unwired: 2 in, 2 out]
        n853 = property on="355nm Laser toggle" class="Bool (strict)"("DisabledEnum"=w1964) -> ()  [unwired: 2 in, 2 out]
        n854 = property on="Aiming beam toggle" class="Bool (strict)"("DisabledEnum"=w1964) -> ()  [unwired: 2 in, 2 out]
        n855 = property on="Background" class="Bool (strict)"("DisabledEnum"=w1964) -> ()  [unwired: 2 in, 2 out]
        n856 = property on="Cali&iRF alignment" class="Bool (strict)"("DisabledEnum"=w1964) -> ()  [unwired: 2 in, 2 out]
        n857 = property on="V 1" class="DigNum (strict)"("Data Range"=w1965) -> ()  [unwired: 2 in, 2 out]
        n858 = property on="V 2" class="DigNum (strict)"("Data Range"=w1965) -> ()  [unwired: 2 in, 2 out]
        n859 = property on="V 3" class="DigNum (strict)"("Data Range"=w1965) -> ()  [unwired: 2 in, 2 out]
        n860 = call <vilib>:"Add State(s) to Queue__JKI_lib_State_Machine.vi"("State(s) in Front (\"\")"="UI: CaliAndiRFNotReady" ("State(s) in Front (\"\")"), "State(s) in (\"\")"=w1971) -> ("States Out"=w1970:string)  [unwired: 13 in]
      }
      frame "UI: BGLoaded" {
        # "[Covers: REQ24]"
        # "Do not put any code in this frame.\n(It is a separator no-op. You can make a copy of this frame to create a new UI frame)"
        n861 = property on="Background" class="Bool (strict)"("BoolText.Text"="Loaded!" ("Boolean Text.Text"), "Colors [4]"=cluster{u32, u32}[] [{15764023, 15764023}, {16711680, 16711680}]) -> ()  [unwired: 2 in, 2 out]
        n862 = call <vilib>:"Add State(s) to Queue__JKI_lib_State_Machine.vi"("State(s) in (\"\")"=w1978) -> ("States Out"=w1977:string)  [unwired: 14 in]
      }
      frame "UI: BGSizeError" {
        # "[Covers: REQ24]"
        # "Do not put any code in this frame.\n(It is a separator no-op. You can make a copy of this frame to create a new UI frame)"
        n863 = property on="Background" class="Bool (strict)"("BoolText.Text"="Loaded!" ("Boolean Text.Text"), "Colors [4]"=cluster{u32, u32}[] [{7171459, 7171459}, {16711680, 16711680}]) -> ()  [unwired: 2 in, 2 out]
        n864 = One Button Dialog(message="Background waveform length and current digitizer setting mismatch! Please take a new background before any aquisition!") -> ()  [unwired: 1 in, 1 out]
        n865 = call <vilib>:"Add State(s) to Queue__JKI_lib_State_Machine.vi"("State(s) in (\"\")"=w1986) -> ("States Out"=w1985:string)  [unwired: 14 in]
      }
      frame "UI: CaliAndiRFLoaded" {
        # "[Covers: REQ24]"
        # "Do not put any code in this frame.\n(It is a separator no-op. You can make a copy of this frame to create a new UI frame)"
        n866 = property on="Cali&iRF alignment" class="Bool (strict)"("BoolText.Text"="Loaded!" ("Boolean Text.Text"), "Colors [4]"=cluster{u32, u32}[] [{15764023, 15764023}, {16711680, 16711680}]) -> ()  [unwired: 2 in, 2 out]
        n867 = call <vilib>:"Add State(s) to Queue__JKI_lib_State_Machine.vi"("State(s) in (\"\")"=w1993) -> ("States Out"=w1992:string)  [unwired: 14 in]
      }
      frame "UI: WFAutoScale" {
        # "Set graph auto scale.\n(UI: WFAutoScale >> T/F)"
        n868 = Equal?(x=w1994, y="F") -> (x = y?=w1995:bool)
        n869 = Equal?(x=w1994, y="T") -> (x = y?=w1997:bool)
        n870 = case shown="True" w1997 {
          frame False {
          }
          frame True {
            w2013 = u8 2 ("Y Scale.Scale Fit")
            n871 = property on="Channel 1" class="WFGraph (strict)"("YScale.ScaleFit"=w2013) -> ()  [unwired: 2 in, 2 out]
            n872 = property on="Channel 2" class="WFGraph (strict)"("YScale.ScaleFit"=w2013) -> ()  [unwired: 2 in, 2 out]
            n873 = property on="Channel 3" class="WFGraph (strict)"("YScale.ScaleFit"=w2013) -> ()  [unwired: 2 in, 2 out]
          }
        }
        n874 = case shown="True" w1995 {
          frame False {
          }
          frame True {
            w2010 = 0.0 ("Y Scale.Range:Maximum")
            w2011 = 2.0 ("Y Scale.Range:Maximum")
            w2012 = u8 0 ("Y Scale.Scale Fit")
            n875 = property on="Channel 1" class="WFGraph (strict)"("YScale.ScaleFit"=w2012) -> (error out=w2009:errorcluster)  [unwired: 2 in, 1 out]
            n876 = property on="Channel 2" class="WFGraph (strict)"("YScale.ScaleFit"=w2012) -> (error out=w2008:errorcluster)  [unwired: 2 in, 1 out]
            n877 = property on="Channel 3" class="WFGraph (strict)"("YScale.ScaleFit"=w2012) -> (error out=w2007:errorcluster)  [unwired: 2 in, 1 out]
            n878 = property on="Channel 1" class="WFGraph (strict)"(error in=w2009, "YScale.Maximum"=w2011) -> (error out=w2006:errorcluster)  [unwired: 1 in, 1 out]
            n879 = property on="Channel 2" class="WFGraph (strict)"(error in=w2008, "YScale.Maximum"=w2011) -> (error out=w2005:errorcluster)  [unwired: 1 in, 1 out]
            n880 = property on="Channel 3" class="WFGraph (strict)"(error in=w2007, "YScale.Maximum"=w2011) -> (error out=w2004:errorcluster)  [unwired: 1 in, 1 out]
            n881 = property on="Channel 1" class="WFGraph (strict)"(error in=w2006, "YScale.Minimum"=w2010) -> ()  [unwired: 1 in, 2 out]
            n882 = property on="Channel 2" class="WFGraph (strict)"(error in=w2005, "YScale.Minimum"=w2010) -> ()  [unwired: 1 in, 2 out]
            n883 = property on="Channel 3" class="WFGraph (strict)"(error in=w2004, "YScale.Minimum"=w2010) -> ()  [unwired: 1 in, 2 out]
          }
        }
        n884 = call <vilib>:"Add State(s) to Queue__JKI_lib_State_Machine.vi"("State(s) in (\"\")"=w2003) -> ("States Out"=w2002:string)  [unwired: 14 in]
      }
      frame "UI: showDisclaimer" {
        # "Show disclamer window.\n(It is a separator no-op. You can make a copy of this frame to create a new UI frame)"
        n885 = call <vilib>:"Application Directory.vi"() -> ("Application Directory"=w2026:path)
        n886 = Build Path(base path=w2026, name or relative path="Disclamer.png") -> (appended path=w2024:path)
        n887 = property on="Disclamer" class="Pict"() -> ("Draw Area Size"=w2022:T40)  [unwired: 2 in, 2 out]
        n888 = disable-structure "Diagram Disable Structure" shown="Disabled" {
          frame Disabled {
            n889 = flat-sequence {
              frame #0 {
                n890 = call "disclaimer.vi"() -> ()  [unwired: 12 in]
              }
              frame #1 {
                n891 = Wait (ms)(milliseconds to wait=u32 250) -> ()  [unwired: 1 out]
              }
              frame #2 {
                n892 = call "SoftwareNote.vi"() -> ()  [unwired: 12 in]
              }
            }
          }
          frame Enabled {
          }
        }
        n893 = call <vilib>:"Read PNG File.vi"("path to PNG file"=w2024) -> ("image data"=w2021:T41)  [unwired: 8 in, 2 out]
        n894 = Unbundle By Name(w2021) -> ("Rectangle.right"=w2019:i16, "Rectangle.bottom"=w2017:i16)
        n895 = Unbundle By Name(w2022) -> ("Width"=w2020:u32, "Height"=w2018:u32)
        n896 = call <vilib>:"Draw Flattened Pixmap.vi"("image data"=w2021) -> ("new picture"=→"Disclamer":picture)  [unwired: 8 in]
        n897 = Divide(x=w2020, y=w2019) -> (x/y=w2016:dbl)
        n898 = Divide(x=w2018, y=w2017) -> (x/y=w2015:dbl)
        n899 = Max & Min(x=w2016, y=w2015) -> (min(x,y)=w2014:dbl)  [unwired: 1 out]
        n900 = property on="Disclamer" class="Pict"("ZoomFactor"=w2014) -> ()  [unwired: 2 in, 2 out]
        n901 = call <vilib>:"Add State(s) to Queue__JKI_lib_State_Machine.vi"("State(s) in (\"\")"=w2031) -> ("States Out"=w2030:string)  [unwired: 14 in]
      }
      frame "UI: CaliAndiRFNotReady" {
        # "Do not put any code in this frame.\n(It is a separator no-op. You can make a copy of this frame to create a new UI frame)"
        n902 = property on="Cali&iRF alignment" class="Bool (strict)"("BoolText.Text"="No Info" ("Boolean Text.Text"), "Colors [4]"=cluster{u32, u32}[] [{13816530, 13816530}, {16711680, 16711680}]) -> ()  [unwired: 2 in, 2 out]
        n903 = call <vilib>:"Add State(s) to Queue__JKI_lib_State_Machine.vi"("State(s) in (\"\")"=w2039) -> ("States Out"=w2038:string)  [unwired: 14 in]
      }
      frame "UI: BGnotReady" {
        # "Do not put any code in this frame.\n(It is a separator no-op. You can make a copy of this frame to create a new UI frame)"
        n904 = property on="Background" class="Bool (strict)"("BoolText.Text"="No Info" ("Boolean Text.Text"), "Colors [4]"=cluster{u32, u32}[] [{13816530, 13816530}, {16711680, 16711680}]) -> ()  [unwired: 2 in, 2 out]
        n905 = call <vilib>:"Add State(s) to Queue__JKI_lib_State_Machine.vi"("State(s) in (\"\")"=w2046) -> ("States Out"=w2045:string)  [unwired: 14 in]
      }
      frame "UI: Reset" {
        w2048 = cluster{u32, u32}[] [{13816530, 13816530}, {13816530, 13816530}] ("Colors [4]")
        # "Do not put any code in this frame.\n(It is a separator no-op. You can make a copy of this frame to create a new UI frame)"
        n906 = property on="Cali&iRF alignment" class="Bool (strict)"("BoolText.Text"="No Info" ("Boolean Text.Text"), "Colors [4]"=w2048) -> ()  [unwired: 2 in, 2 out]
        n907 = property on="Background" class="Bool (strict)"("BoolText.Text"="No Info" ("Boolean Text.Text"), "Colors [4]"=w2048) -> ()  [unwired: 2 in, 2 out]
        n908 = call <vilib>:"Add State(s) to Queue__JKI_lib_State_Machine.vi"("State(s) in (\"\")"=w2054) -> ("States Out"=w2053:string)  [unwired: 14 in]
      }
      frame "UI: SetButtonText" {
        # "Set button text of 355nm laser and aiming beam."
        n909 = call <vilib>:"Add State(s) to Queue__JKI_lib_State_Machine.vi"("State(s) in (\"\")"=w2059) -> ("States Out"=w2058:string)  [unwired: 14 in]
      }
      frame "UI: DuringAquisition" {
        w2060 = T17."Disabled and Grayed Out" ("Disabled")
        # "Do not put any code in this frame.\n(It is a separator no-op. You can make a copy of this frame to create a new UI frame)"
        n910 = property on="StartButton" class="Bool (strict)"("DisabledEnum"=w2060) -> ()  [unwired: 2 in, 2 out]
        n911 = property on="Sys Reconfig" class="Bool"("DisabledEnum"=w2060) -> ()  [unwired: 2 in, 2 out]
        n912 = property on="355nm Laser toggle" class="Bool (strict)"("DisabledEnum"=w2060) -> ()  [unwired: 2 in, 2 out]
        n913 = property on="Skip Data Save?" class="Bool (strict)"("DisabledEnum"=w2060) -> ()  [unwired: 2 in, 2 out]
        n914 = property on="Aiming beam toggle" class="Bool (strict)"("DisabledEnum"=w2060) -> ()  [unwired: 2 in, 2 out]
        n915 = property on="Background" class="Bool (strict)"("DisabledEnum"=w2060) -> ()  [unwired: 2 in, 2 out]
        n916 = property on="Cali&iRF alignment" class="Bool (strict)"("DisabledEnum"=w2060) -> ()  [unwired: 2 in, 2 out]
        n917 = property on="Skip Data Save?" class="Bool (strict)"("DisabledEnum"=w2060) -> ()  [unwired: 2 in, 2 out]
        n918 = property on="Quit" class="Bool"("DisabledEnum"=w2060) -> ()  [unwired: 2 in, 2 out]
        n919 = local read "Skip Data Save?"() -> (w2061:bool)
        n920 = case shown="False" w2061 {
          tunnel: w2060 -> [w2068 _]
          frame False {
            # "if saving data, disable V adjustment"
            n921 = property on="V 3" class="DigNum (strict)"("DisabledEnum"=w2068) -> ()  [unwired: 2 in, 2 out]
            n922 = property on="V 1" class="DigNum (strict)"("DisabledEnum"=w2068) -> ()  [unwired: 2 in, 2 out]
            n923 = property on="V 2" class="DigNum (strict)"("DisabledEnum"=w2068) -> ()  [unwired: 2 in, 2 out]
          }
          frame True {
            # "if skip data save, do nothing"
          }
        }
        n924 = property on="StopButton" class="Bool (strict)"("DisabledEnum"=T17."Enabled" ("Disabled")) -> ()  [unwired: 2 in, 2 out]
        n925 = call <vilib>:"Add State(s) to Queue__JKI_lib_State_Machine.vi"("State(s) in (\"\")"=w2067) -> ("States Out"=w2066:string)  [unwired: 14 in]
      }
      frame "UI: duringIRFAlign" {
        w2069 = T17."Disabled and Grayed Out" ("Disabled")
        # "Set UI to during iRF alignment\n(It is a separator no-op. You can make a copy of this frame to create a new UI frame)"
        n926 = property on="StartButton" class="Bool (strict)"("DisabledEnum"=w2069) -> ()  [unwired: 2 in, 2 out]
        n927 = property on="Sys Reconfig" class="Bool"("DisabledEnum"=w2069) -> ()  [unwired: 2 in, 2 out]
        n928 = property on="355nm Laser toggle" class="Bool (strict)"("DisabledEnum"=w2069) -> ()  [unwired: 2 in, 2 out]
        n929 = property on="Aiming beam toggle" class="Bool (strict)"("DisabledEnum"=w2069) -> ()  [unwired: 2 in, 2 out]
        n930 = property on="Background" class="Bool (strict)"("DisabledEnum"=w2069) -> ()  [unwired: 2 in, 2 out]
        n931 = property on="StopButton" class="Bool (strict)"("DisabledEnum"=w2069) -> ()  [unwired: 2 in, 2 out]
        n932 = call <vilib>:"Add State(s) to Queue__JKI_lib_State_Machine.vi"("State(s) in (\"\")"=w2074) -> ("States Out"=w2073:string)  [unwired: 14 in]
      }
      frame "UI: duringBGAcquire" {
        w2075 = T17."Disabled and Grayed Out" ("Disabled")
        # "Do not put any code in this frame.\n(It is a separator no-op. You can make a copy of this frame to create a new UI frame)"
        n933 = property on="StartButton" class="Bool (strict)"("DisabledEnum"=w2075) -> ()  [unwired: 2 in, 2 out]
        n934 = property on="StopButton" class="Bool (strict)"("DisabledEnum"=w2075) -> ()  [unwired: 2 in, 2 out]
        n935 = property on="Sys Reconfig" class="Bool"("DisabledEnum"=w2075) -> ()  [unwired: 2 in, 2 out]
        n936 = property on="355nm Laser toggle" class="Bool (strict)"("DisabledEnum"=w2075) -> ()  [unwired: 2 in, 2 out]
        n937 = property on="Aiming beam toggle" class="Bool (strict)"("DisabledEnum"=w2075) -> ()  [unwired: 2 in, 2 out]
        n938 = property on="Cali&iRF alignment" class="Bool (strict)"("DisabledEnum"=w2075) -> ()  [unwired: 2 in, 2 out]
        n939 = call <vilib>:"Add State(s) to Queue__JKI_lib_State_Machine.vi"("State(s) in (\"\")"=w2080) -> ("States Out"=w2079:string)  [unwired: 14 in]
      }
      frame "UI: ReadyForAquisition" {
        w2081 = T17."Enabled" ("Disabled")
        # "Do not put any code in this frame.\n(It is a separator no-op. You can make a copy of this frame to create a new UI frame)"
        n940 = property on="StartButton" class="Bool (strict)"("DisabledEnum"=w2081) -> ()  [unwired: 2 in, 2 out]
        n941 = property on="Skip Data Save?" class="Bool (strict)"("DisabledEnum"=w2081) -> ()  [unwired: 2 in, 2 out]
        n942 = property on="Sys Reconfig" class="Bool"("DisabledEnum"=w2081) -> ()  [unwired: 2 in, 2 out]
        n943 = property on="355nm Laser toggle" class="Bool (strict)"("DisabledEnum"=w2081) -> ()  [unwired: 2 in, 2 out]
        n944 = property on="Background" class="Bool (strict)"("DisabledEnum"=w2081) -> ()  [unwired: 2 in, 2 out]
        n945 = property on="Cali&iRF alignment" class="Bool (strict)"("DisabledEnum"=w2081) -> ()  [unwired: 2 in, 2 out]
        n946 = property on="V 1" class="DigNum (strict)"("DisabledEnum"=w2081) -> ()  [unwired: 2 in, 2 out]
        n947 = property on="V 2" class="DigNum (strict)"("DisabledEnum"=w2081) -> ()  [unwired: 2 in, 2 out]
        n948 = property on="V 3" class="DigNum (strict)"("DisabledEnum"=w2081) -> ()  [unwired: 2 in, 2 out]
        n949 = property on="Quit" class="Bool"("DisabledEnum"=w2081) -> ()  [unwired: 2 in, 2 out]
        n950 = property on="StopButton" class="Bool (strict)"("DisabledEnum"=T17."Disabled and Grayed Out" ("Disabled")) -> ()  [unwired: 2 in, 2 out]
        n951 = call <vilib>:"Add State(s) to Queue__JKI_lib_State_Machine.vi"("State(s) in (\"\")"=w2087) -> ("States Out"=w2086:string)  [unwired: 14 in]
      }
      frame "UI: Update" {
        # "Do not put any code in this frame.\n(It is a separator no-op. You can make a copy of this frame to create a new UI frame)"
        n952 = Unbundle By Name(w2098) -> ("System Status"=→"System Hardware Connection Status":T2, "IDs.RunID"=→"Run #":i8, "CaseID"=→"Case #":string, "FLImDAQ"=→"FLImDAQ":T26, "SysRunning?"=→"Aquisition Status:":bool, "LJ Pinout"=→"LJ Pinout":T5, "IDs.BG ID"=→"BG #":i8, "IDs.Cali ID"=→"Calibration #":i8, "video source"=→"Visualization PC video source":T1)
        n953 = call <vilib>:"Add State(s) to Queue__JKI_lib_State_Machine.vi"("State(s) in (\"\")"=w2101) -> ("States Out"=w2100:string)  [unwired: 14 in]
      }
      frame "UI: updateVideoToggle" {
        # "Set video toggle based on visualization PC video source.\n(take )"
        n954 = call <vilib>:"Add State(s) to Queue__JKI_lib_State_Machine.vi"("State(s) in (\"\")"=w2106) -> ("States Out"=w2105:string)  [unwired: 14 in]
      }
      frame "UI: Cursor Set" {
        # "Argument"
        # "Set and Unset Cursor Busy.\n(Usage: \"UI: Cursor Set >> Busy|Idle\")"
        n955 = case shown="\"Busy\"" w2108 {
          tunnel: w2110 -> [w2115 w2117]
          tunnel: [w2114 w2116] -> w2109
          frame "Idle", Default {
            n956 = call <vilib>:"Unset Busy.vi"("error in (no error)"=w2115) -> ("error out"=w2114:errorcluster)  [unwired: 10 in]
          }
          frame "Busy" {
            n957 = call <vilib>:"Set Busy.vi"("error in (no error)"=w2117) -> ("error out"=w2116:errorcluster)  [unwired: 9 in, 1 out]
          }
        }
        n958 = call <vilib>:"Add State(s) to Queue__JKI_lib_State_Machine.vi"("State(s) in (\"\")"=w2113) -> ("States Out"=w2112:string)  [unwired: 14 in]
      }
      frame "UI: Front Panel State" {
        # "Argument"
        # "Set Front Panel Open or Closed\n(Usage: \"UI: Front Panel State >> Open|Close\")"
        n959 = Unbundle By Name(w2121) -> ("Core.Current VI Reference"=w2120:refnum<vi>)
        n960 = case shown="\"Open\", \"Standard\", Default" w2119 {
          tunnel: w2123 -> [w2131 w2146 w2157 w2170 w2183]
          tunnel: [w2133 w2147 w2159 w2172 w2185] -> w2122
          tunnel: w2120 -> [w2132 w2144 w2158 w2171 w2184]
          frame "Open", "Standard", Default {
            w2126 = T13."Standard" ("State")
            n961 = property on="Property Node" class="VI"(reference=w2132, error in=w2131) -> (reference out=w2129:refnum<vi>, error out=w2130:errorcluster, "FP.State"=w2128:T13)
            n962 = Not Equal?(x=w2128, y=w2126) -> (x != y?=w2127:bool)
            n963 = case shown="True" w2127 {
              tunnel: [w2137 w2139] -> w2133
              tunnel: w2130 -> [w2136 w2139]
              tunnel: w2129 -> [w2135 _]
              tunnel: w2126 -> [w2134 _]
              frame True {
                n964 = invoke on="Invoke Node" class="VI" method="FP.Open"(reference=w2135, error in=w2136, "Activate"=TRUE, "State"=w2134) -> (error out=w2137:errorcluster)  [unwired: 1 in, 4 out]
              }
              frame False {
              }
            }
          }
          frame "Close", "Closed" {
            n965 = property on="Property Node" class="VI"(reference=w2144, error in=w2146) -> (reference out=w2143:refnum<vi>, error out=w2145:errorcluster, "FP.State"=w2141:T13)
            n966 = Not Equal?(x=w2141, y=T13."Closed" ("Front Panel Window:State")) -> (x != y?=w2140:bool)
            n967 = case shown="True" w2140 {
              tunnel: [w2148 w2151] -> w2147
              tunnel: w2145 -> [w2148 w2150]
              tunnel: w2143 -> [_ w2149]
              frame False {
              }
              frame True {
                n968 = invoke on="Invoke Node" class="VI" method="FP.Close"(reference=w2149, error in=w2150) -> (error out=w2151:errorcluster)  [unwired: 1 in, 2 out]
              }
            }
          }
          frame "Hidden", "Hide" {
            w2152 = T13."Hidden" ("State")
            n969 = property on="Property Node" class="VI"(reference=w2158, error in=w2157) -> (reference out=w2155:refnum<vi>, error out=w2156:errorcluster, "FP.State"=w2154:T13)
            n970 = Not Equal?(x=w2154, y=w2152) -> (x != y?=w2153:bool)
            n971 = case shown="True" w2153 {
              tunnel: [w2163 w2164] -> w2159
              tunnel: w2156 -> [w2162 w2164]
              tunnel: w2155 -> [w2161 _]
              tunnel: w2152 -> [w2160 _]
              frame True {
                n972 = invoke on="Invoke Node" class="VI" method="FP.Open"(reference=w2161, error in=w2162, "State"=w2160) -> (error out=w2163:errorcluster)  [unwired: 2 in, 4 out]
              }
              frame False {
              }
            }
          }
          frame "Minimize", "Minimized" {
            w2165 = T13."Minimized" ("State")
            n973 = property on="Property Node" class="VI"(reference=w2171, error in=w2170) -> (reference out=w2168:refnum<vi>, error out=w2169:errorcluster, "FP.State"=w2167:T13)
            n974 = Not Equal?(x=w2167, y=w2165) -> (x != y?=w2166:bool)
            n975 = case shown="True" w2166 {
              tunnel: [w2176 w2177] -> w2172
              tunnel: w2169 -> [w2175 w2177]
              tunnel: w2168 -> [w2174 _]
              tunnel: w2165 -> [w2173 _]
              frame True {
                n976 = invoke on="Invoke Node" class="VI" method="FP.Open"(reference=w2174, error in=w2175, "State"=w2173) -> (error out=w2176:errorcluster)  [unwired: 2 in, 4 out]
              }
              frame False {
              }
            }
          }
          frame "Maximize", "Maximized" {
            w2178 = T13."Maximized" ("State")
            n977 = property on="Property Node" class="VI"(reference=w2184, error in=w2183) -> (reference out=w2181:refnum<vi>, error out=w2182:errorcluster, "FP.State"=w2180:T13)
            n978 = Not Equal?(x=w2180, y=w2178) -> (x != y?=w2179:bool)
            n979 = case shown="True" w2179 {
              tunnel: [w2189 w2190] -> w2185
              tunnel: w2182 -> [w2188 w2190]
              tunnel: w2181 -> [w2187 _]
              tunnel: w2178 -> [w2186 _]
              frame True {
                n980 = invoke on="Invoke Node" class="VI" method="FP.Open"(reference=w2187, error in=w2188, "State"=w2186) -> (error out=w2189:errorcluster)  [unwired: 2 in, 4 out]
              }
              frame False {
              }
            }
          }
        }
        n981 = call <vilib>:"Add State(s) to Queue__JKI_lib_State_Machine.vi"("State(s) in (\"\")"=w2125) -> ("States Out"=w2124:string)  [unwired: 14 in]
      }
      frame "---------- AimingBeam ----------" {
        # "Template Separator\n(You can make a copy of, or modify, this frame)"
        n982 = call <vilib>:"Add State(s) to Queue__JKI_lib_State_Machine.vi"("State(s) in (\"\")"=w2195) -> ("States Out"=w2194:string)  [unwired: 14 in]
      }
      frame "AimingBeam: Initialize" {
        # "set aiming beam button color"
        # "Open COM port for Aiming Beam\n(Require USB connection)"
        n983 = Unbundle By Name(w2197) -> ("AB Cluster.Aiming Beam COM Port"=w2205:refnum<visa-resource-name>)
        n984 = call-poly "VISA Configure Serial Port"("VISA resource name"=w2205, "Enable Termination\nChar (T)"=TRUE ("Enable Termination\nChar (T)"), "baud rate (9600)"=u32 9600, "error in (no error)"=w2202) -> ("error out"=w2201:errorcluster)  [unwired: 10 in, 1 out]
        n985 = Unbundle By Name(w2201) -> ("status"=w2200:bool)
        n986 = Not(x=w2200) -> (.not. x?=w2199:bool)
        n987 = Bundle By Name(cluster=w2197, "System Status.Aiming Beam"=w2199) -> (w2198:T19)
        n988 = call <vilib>:"Add State(s) to Queue__JKI_lib_State_Machine.vi"("State(s) in (\"\")"=w2207) -> ("States Out"=w2206:string)  [unwired: 14 in]
      }
      frame "AimingBeam: Close" {
        # "Close Aiming Beam COM port\n(Require USB connection to Aiming Beam Laser)"
        n989 = Unbundle By Name(w2210) -> ("AB Cluster.Aiming Beam COM Port"=w2214:refnum<visa-resource-name>)
        n990 = VISA Close(VISA resource name=w2214, error in (no error)=w2212) -> (error out=w2213:errorcluster)
        n991 = Bundle By Name(cluster=w2210, "System Status.Aiming Beam"=FALSE) -> (w2211:T19)
        n992 = call <vilib>:"Add State(s) to Queue__JKI_lib_State_Machine.vi"("State(s) in (\"\")"=w2216) -> ("States Out"=w2215:string)  [unwired: 14 in]
      }
      frame "AimingBeam: Set Current" {
        # "Set Aiming Beam Current\n(You can make a copy of, or modify, this frame)"
        n993 = Unbundle By Name(w2231) -> ("AB Cluster.Aiming Beam COM Port"=w2224:refnum<visa-resource-name>, "AB Cluster.Max Current"=w2220:dbl, "AB Cluster.Default Current"=w2222:dbl, "AB Cluster.Min Current"=w2221:dbl)
        n994 = In Range and Coerce(upper limit=w2220, x=w2222, lower limit=w2221) -> (coerced(x)=w2217:dbl)  [unwired: 1 out]
        n995 = Number To Fractional String(number=w2217, precision (6)=i16 2) -> (F-format string=w2225:string)  [unwired: 2 in]
        n996 = Concatenate Strings("slc:", w2225, "\r" ("Carriage Return Constant"), "\n" ("Line Feed Constant")) -> (w2228:string)
        n997 = VISA Write(VISA resource name=w2224, write buffer=w2228, error in (no error)=w2219) -> (error out=w2223:errorcluster)  [unwired: 2 out]
        n998 = call <vilib>:"Add State(s) to Queue__JKI_lib_State_Machine.vi"("State(s) in (\"\")"=w2233) -> ("States Out"=w2232:string)  [unwired: 14 in]
      }
      frame "AimingBeam: Set Status" {
        # "Enable Aiming Beam\n(Usage: \"AimingBeam: Set >> Enable|Disable\")"
        n999 = Unbundle By Name(w2240) -> ("AB Cluster.Aiming Beam COM Port"=w2237:refnum<visa-resource-name>)
        n1000 = case shown="\"Enable\"" w2239 {
          tunnel: [w2243 w2247] -> w2238
          frame "Disable", Default {
            n1001 = Concatenate Strings("cof", "\r" ("Carriage Return Constant"), "\n" ("Line Feed Constant")) -> (w2243:string)
          }
          frame "Enable" {
            n1002 = Concatenate Strings("con", "\r" ("Carriage Return Constant"), "\n" ("Line Feed Constant")) -> (w2247:string)
          }
        }
        n1003 = VISA Write(VISA resource name=w2237, write buffer=w2238, error in (no error)=w2235) -> (error out=w2236:errorcluster)  [unwired: 2 out]
        n1004 = call <vilib>:"Add State(s) to Queue__JKI_lib_State_Machine.vi"("State(s) in (\"\")"=w2242) -> ("States Out"=w2241:string)  [unwired: 14 in]
      }
      frame "AimingBeam: GetPWMStatus" {
        # "Get aiming beam PWM status\n()"
        n1005 = Unbundle By Name(w2255) -> ("AB Cluster.Freq"=w2254:i32, "LJ Pinout.AimingBeam PWM"=w2261:string)
        n1006 = Equal To 0?(x=w2254) -> (x = 0?=w2253:bool)
        n1007 = call "LabJack_FGV.vi"("Operation(Read)"=enum16{"Write", "Read"}."Read" ("Operation"), "error in (no error)"=w2257) -> ("error out"=w2259:errorcluster, "Read data"=w2260:i32)  [unwired: 8 in]
        n1008 = case shown="True" w2253 {
          tunnel: w2261 -> [w2274 _]
          tunnel: [w2272 "DIO_STATE"] -> w2258
          frame False {
            n1009 = Concatenate Strings(w2274, "_EF_ENABLE" ("string")) -> (w2272:string)
          }
          frame True {
          }
        }
        n1010 = call "LJM_eReadName.vi"("Handle In"=w2260, "Name"=w2258, "error in"=w2259) -> ("Value"=w2252:dbl, "error out"=w2256:errorcluster)  [unwired: 10 in, 1 out]
        n1011 = case shown="True" w2253 {
          tunnel: w2252 -> [w2267 w2271]
          tunnel: [w2266 w2268] -> w2251
          frame False {
            n1012 = Greater Than 0?(x=w2267) -> (x > 0?=w2266:bool)
          }
          frame True {
            n1013 = Number To Boolean Array(number=w2271) -> (Boolean array=w2270:bool[])
            n1014 = Index Array(array=w2270, index=3) -> (element=w2268:bool)
          }
        }
        n1015 = case shown="False" w2251 {
          frame False {
            # "PWM is off\nset color to dark green"
            n1016 = local write "Aiming beam toggle"(FALSE ("Aimging beam")) -> ()
          }
          frame True {
            # "PWM is on\nset color to light green"
            n1017 = local write "Aiming beam toggle"(TRUE ("Aimging beam")) -> ()
          }
        }
        n1018 = call <vilib>:"Add State(s) to Queue__JKI_lib_State_Machine.vi"("State(s) in (\"\")"=w2265) -> ("States Out"=w2264:string)  [unwired: 14 in]
      }
      frame "---------- 355 Laser ----------" {
        # "Template Separator\n(You can make a copy of, or modify, this frame)"
        n1019 = call <vilib>:"Add State(s) to Queue__JKI_lib_State_Machine.vi"("State(s) in (\"\")"=w2282) -> ("States Out"=w2281:string)  [unwired: 14 in]
      }
      frame "355 Laser: Check Dewelling" {
        # "if time laser start time is less than 7.5s before, wait 250ms then check again."
        # "Template Separator\n(You can make a copy of, or modify, this frame)"
        n1020 = Unbundle By Name(w2290) -> ("Laser start tic"=w2287:u32)
        n1021 = Tick Count (ms)() -> (millisecond timer value=w2288:u32)
        n1022 = Subtract(x=w2288, y=w2287) -> (x-y=w2286:u32)
        n1023 = Greater?(x=w2286, y=u32 5000) -> (0:w2284:bool)
        n1024 = case shown="False" w2284 {
          tunnel: ["355 Laser: Check Dewelling" ""] -> w2283
          frame False {
            n1025 = Wait (ms)(milliseconds to wait=u32 250) -> ()  [unwired: 1 out]
          }
          frame True {
          }
        }
        n1026 = call <vilib>:"Add State(s) to Queue__JKI_lib_State_Machine.vi"("State(s) in Front (\"\")"=w2283, "State(s) in (\"\")"=w2293) -> ("States Out"=w2292:string)  [unwired: 13 in]
      }
      frame "355 Laser: Laser enable" {
        # "Laser enable/disable\n(Usage: \"LabJack: Laser enable/disable >> 1|0\")"
        n1027 = Unbundle By Name(w2300) -> ("LJ Pinout.Laser Start/Stop"=w2304:string, "System Status.355 Laser"=w2298:bool)
        n1028 = case shown="False" w2298 {
          tunnel: w2297 -> [w2319 w2320]
          tunnel: w2304 -> [w2313 _]
          tunnel: [w2308 w2320] -> w2302
          tunnel: [w2307 u32 0 ("millisecond timer value")] -> w2299
          frame False {
            n1029 = call "LabJack_FGV.vi"("Operation(Read)"=enum16{"Write", "Read"}."Read" ("Operation")) -> ("Read data"=w2315:i32)  [unwired: 9 in, 1 out]
            n1030 = call "LJM_eWriteName.vi"("Handle In"=w2315, "Name"=w2313, "Value"=1.0, "error in"=w2319) -> ("Handle Out"=w2314:i32, "error out"=w2312:errorcluster)  [unwired: 10 in]
            n1031 = call <userlib>:"Wait (ms)__ogtk.vi"("error in (no error)"=w2312, "milliseconds to wait"=u32 250) -> ("error out"=w2311:errorcluster)  [unwired: 8 in, 1 out]
            n1032 = call "LJM_eWriteName.vi"("Handle In"=w2314, "Name"=w2313, "Value"=0.0, "error in"=w2311) -> ("error out"=w2309:errorcluster)  [unwired: 10 in, 1 out]
            n1033 = call <userlib>:"Tick Count (ms)__ogtk.vi"("error in (no error)"=w2309) -> ("error out"=w2308:errorcluster, "millisecond timer value"=w2307:u32)  [unwired: 9 in]
          }
          frame True {
          }
        }
        n1034 = Bundle By Name(cluster=w2300, "Laser start tic"=w2299) -> (w2301:T19)
        n1035 = call <vilib>:"Add State(s) to Queue__JKI_lib_State_Machine.vi"("State(s) in (\"\")"=w2306) -> ("States Out"=w2305:string)  [unwired: 14 in]
      }
      frame "355 Laser: Laser disable" {
        # "Laser enable/disable\n(Usage: \"LabJack: Laser enable/disable >> 1|0\")"
        n1036 = Unbundle By Name(w2324) -> ("LJ Pinout.Laser Start/Stop"=w2328:string, "System Status.355 Laser"=w2322:bool)
        n1037 = case shown="True" w2322 {
          tunnel: w2329 -> [w2332 w2346]
          tunnel: w2328 -> [_ w2340]
          tunnel: [w2332 w2335] -> w2326
          tunnel: [u32 0 ("millisecond timer value") w2334] -> w2323
          frame False {
          }
          frame True {
            n1038 = call "LabJack_FGV.vi"("Operation(Read)"=enum16{"Write", "Read"}."Read" ("Operation")) -> ("Read data"=w2342:i32)  [unwired: 9 in, 1 out]
            n1039 = call "LJM_eWriteName.vi"("Handle In"=w2342, "Name"=w2340, "Value"=1.0, "error in"=w2346) -> ("Handle Out"=w2341:i32, "error out"=w2339:errorcluster)  [unwired: 10 in]
            n1040 = call <userlib>:"Wait (ms)__ogtk.vi"("error in (no error)"=w2339, "milliseconds to wait"=u32 250) -> ("error out"=w2338:errorcluster)  [unwired: 8 in, 1 out]
            n1041 = call "LJM_eWriteName.vi"("Handle In"=w2341, "Name"=w2340, "Value"=0.0, "error in"=w2338) -> ("error out"=w2336:errorcluster)  [unwired: 10 in, 1 out]
            n1042 = call <userlib>:"Tick Count (ms)__ogtk.vi"("error in (no error)"=w2336) -> ("error out"=w2335:errorcluster, "millisecond timer value"=w2334:u32)  [unwired: 9 in]
          }
        }
        n1043 = Bundle By Name(cluster=w2324, "Laser start tic"=w2323) -> (w2325:T19)
        n1044 = call <vilib>:"Add State(s) to Queue__JKI_lib_State_Machine.vi"("State(s) in (\"\")"=w2331) -> ("States Out"=w2330:string)  [unwired: 14 in]
      }
      frame "355 Laser: Dewelling" {
        # "Wait some time (ms)\n(355 Laser: Dewelling >> #)"
        n1045 = Fract/Exp String To Number(string=w2350, default (0 dbl)=0) -> (number=w2348:i32)  [unwired: 2 in, 1 out]
        n1046 = Wait (ms)(milliseconds to wait=w2348) -> ()  [unwired: 1 out]
        n1047 = call <vilib>:"Add State(s) to Queue__JKI_lib_State_Machine.vi"("State(s) in (\"\")"=w2354) -> ("States Out"=w2353:string)  [unwired: 14 in]
      }
      frame "355 Laser: Close" {
        # "Template Separator\n(You can make a copy of, or modify, this frame)"
        n1048 = call <vilib>:"Add State(s) to Queue__JKI_lib_State_Machine.vi"("State(s) in Front (\"\")"="355 Laser: CheckControllerStatus\n355 Laser: Laser disable\n355 Laser: Dewelling >>1000", "State(s) in (\"\")"=w2360) -> ("States Out"=w2359:string)  [unwired: 13 in]
      }
      frame "355 Laser: CheckControllerStatus" {
        # "if average < 2, laser no power\nif average 2 < average < 9.3, laser on\nif 9.3<average<10, interlock open, blink indicator\nif average > 10, laser off\n[Covers: REQ30]"
        # "take 10 measuremt and look at average"
        # "Check 355 laser controller status\nBy probing Emisison Lamp negative terminal voltage"
        n1049 = Unbundle By Name(w2369) -> ("LJ Pinout.Laser Ready"=w2372:string)
        n1050 = call "LabJack_FGV.vi"("Operation(Read)"=enum16{"Write", "Read"}."Read" ("Operation")) -> ("Read data"=w2373:i32)  [unwired: 9 in, 1 out]
        n1051 = for {
          N: 20 -> [_]
          tunnel: w2373 -> [w2384]
          tunnel: w2372 -> [w2383]
          shift-right: [w2382] -> w2365
          shift-left: w2371 -> [w2381]
          tunnel: [w2379] -> w2364 mode=indexing
          n1052 = call "LJM_eReadName.vi"("Handle In"=w2384, "Name"=w2383, "error in"=w2381) -> ("Value"=w2379:dbl, "error out"=w2382:errorcluster)  [unwired: 10 in, 1 out]
          n1053 = Wait (ms)(milliseconds to wait=u32 25) -> ()  [unwired: 1 out]
        }
        n1054 = call "checkLaserStatus.vi"("error in (no error)"=w2365, "Laser LED voltage"=w2364) -> ("error out"=w2366:errorcluster, "Interlock open?"=w2361:bool, "Laser on?"=w2363:bool, "Mean voltage"=→"laser EM lamp V":dbl)  [unwired: 6 in]
        n1055 = Bundle By Name(cluster=w2369, "System Status.355 Laser"=w2363) -> (w2370:T19)
        n1056 = case shown="True" w2361 {
          frame False {
            n1057 = property on="355 Laser" class="Bool (strict)"("Blinking"=FALSE) -> ()  [unwired: 2 in, 2 out]
          }
          frame True {
            n1058 = property on="355 Laser" class="Bool (strict)"("Blinking"=TRUE) -> ()  [unwired: 2 in, 2 out]
          }
        }
        n1059 = call <vilib>:"Add State(s) to Queue__JKI_lib_State_Machine.vi"("State(s) in (\"\")"=w2376) -> ("States Out"=w2375:string)  [unwired: 14 in]
      }
      frame "355 Laser: CheckPWMStatus" {
        # "Check 355 laser PWM status\n(Read LJ DIO#EF_ENABLE register to determine PWM status)"
        n1060 = Unbundle By Name(w2394) -> ("LJ Pinout.355 PWM"=w2393:string)
        n1061 = call "LabJack_FGV.vi"("Operation(Read)"=enum16{"Write", "Read"}."Read" ("Operation"), "error in (no error)"=w2387) -> ("error out"=w2390:errorcluster, "Read data"=w2391:i32)  [unwired: 8 in]
        n1062 = Concatenate Strings(w2393, "_EF_ENABLE" ("string")) -> (w2389:string)
        n1063 = call "LJM_eReadName.vi"("Handle In"=w2391, "Name"=w2389, "error in"=w2390) -> ("Value"=w2386:dbl, "error out"=w2388:errorcluster)  [unwired: 10 in, 1 out]
        n1064 = Greater Than 0?(x=w2386) -> (x > 0?=w2385:bool)
        n1065 = case shown="False" w2385 {
          frame False {
            # "PWM is off\nset color to gray"
            n1066 = local write "355nm Laser toggle"(FALSE ("355nm Laser")) -> ()
          }
          frame True {
            # "PWM is on\nset color to light green"
            n1067 = local write "355nm Laser toggle"(TRUE ("355nm Laser")) -> ()
          }
        }
        n1068 = call <vilib>:"Add State(s) to Queue__JKI_lib_State_Machine.vi"("State(s) in (\"\")"=w2398) -> ("States Out"=w2397:string)  [unwired: 14 in]
      }
      frame "355 Laser: Start" {
        # "Template Separator\n(You can make a copy of, or modify, this frame)"
        n1069 = call <vilib>:"Add State(s) to Queue__JKI_lib_State_Machine.vi"("State(s) in Front (\"\")"="LabJack: 355_PWM_Start", "State(s) in (\"\")"=w2406) -> ("States Out"=w2405:string)  [unwired: 13 in]
      }
      frame "355 Laser: Stop" {
        # "Template Separator\n(You can make a copy of, or modify, this frame)"
        n1070 = call <vilib>:"Add State(s) to Queue__JKI_lib_State_Machine.vi"("State(s) in Front (\"\")"="LabJack: 355_PWM_Stop", "State(s) in (\"\")"=w2412) -> ("States Out"=w2411:string)  [unwired: 13 in]
      }
      frame "---------- Utility ----------" {
        # "Template Separator\n(You can make a copy of, or modify, this frame)"
        n1071 = call <vilib>:"Add State(s) to Queue__JKI_lib_State_Machine.vi"("State(s) in (\"\")"=w2417) -> ("States Out"=w2416:string)  [unwired: 14 in]
      }
      frame "Utility: SetDataClass" {
        # "Set Data Class in Queues\n(Set data class to either Data, Bg or Cali)"
        n1072 = case shown="\"Cali\"" w2419 {
          tunnel: [enum16{"Data", "BG", "Cali"}."Data" ("Data Class") enum16{"Data", "BG", "Cali"}."BG" ("Data Class") enum16{"Data", "BG", "Cali"}."Cali" ("Data Class")] -> w2418
          frame "Data", Default {
          }
          frame "Bg" {
          }
          frame "Cali" {
          }
        }
        n1073 = local write "Data Class"(w2418) -> ()
        n1074 = call <vilib>:"Add State(s) to Queue__JKI_lib_State_Machine.vi"("State(s) in (\"\")"=w2424) -> ("States Out"=w2423:string)  [unwired: 14 in]
      }
      frame "Utility: AquiTimerReset" {
        # "Set Aquisition Timer\n(You can make a copy of, or modify, this frame)"
        n1075 = Tick Count (ms)() -> (millisecond timer value=w2430:u32)
        n1076 = Bundle By Name(cluster=w2428, "Aquisition Timer"=w2430) -> (w2429:T19)
        n1077 = call <vilib>:"Add State(s) to Queue__JKI_lib_State_Machine.vi"("State(s) in (\"\")"=w2434) -> ("States Out"=w2433:string)  [unwired: 14 in]
      }
      frame "Utility: AquiTimerCheck" {
        # "5min to ms"
        # "Set Aquisition Timer\n([Covers: REQ35])"
        n1078 = Unbundle By Name(w2442) -> ("Aquisition Timer"=w2440:u32)
        n1079 = Tick Count (ms)() -> (millisecond timer value=w2441:u32)
        n1080 = Subtract(x=w2441, y=w2440) -> (x-y=w2439:u32)
        n1081 = Multiply(x=1000, y=300) -> (x*y=w2436:i32)
        n1082 = Greater Or Equal?(x=w2439, y=w2436) -> (x >= y?=w2435:bool)
        n1083 = case shown="True" w2435 {
          frame False {
            # "do nothing"
          }
          frame True {
            # "if timed out, stop aquisition"
            n1084 = property on="StopButton" class="Bool (strict)"("Val(Sgnl)"=TRUE ("Value (Signaling)")) -> ()  [unwired: 2 in, 2 out]
          }
        }
        n1085 = call <vilib>:"Add State(s) to Queue__JKI_lib_State_Machine.vi"("State(s) in (\"\")"=w2446) -> ("States Out"=w2445:string)  [unwired: 14 in]
      }
      frame "Utility: StartBeep" {
        # "Beep\n([Covers: REQ18])"
        n1086 = call <vilib>:"Beep.vi"("use system alert? (T)"=FALSE, "duration (msec)"=u32 1000, "frequency (Hz)"=u32 2000) -> ()  [unwired: 9 in]
        n1087 = call <vilib>:"Add State(s) to Queue__JKI_lib_State_Machine.vi"("State(s) in (\"\")"=w2455) -> ("States Out"=w2454:string)  [unwired: 14 in]
      }
      frame "Utility: EndBeep" {
        # "Beep\n([Covers: REQ18])"
        n1088 = flat-sequence {
          frame #0 {
            n1089 = call <vilib>:"Beep.vi"("use system alert? (T)"=FALSE, "duration (msec)"=u32 500, "frequency (Hz)"=u32 2000) -> ()  [unwired: 9 in]
          }
          frame #1 {
            n1090 = call <vilib>:"Beep.vi"("use system alert? (T)"=FALSE, "duration (msec)"=u32 500, "frequency (Hz)"=u32 2000) -> ()  [unwired: 9 in]
          }
        }
        n1091 = call <vilib>:"Add State(s) to Queue__JKI_lib_State_Machine.vi"("State(s) in (\"\")"=w2460) -> ("States Out"=w2459:string)  [unwired: 14 in]
      }
      frame "Utility: Dewelling" {
        # "Main loop dewell\n(Dewelling >> #)"
        n1092 = Fract/Exp String To Number(string=w2470, default (0 dbl)=0) -> (number=w2468:i32)  [unwired: 2 in, 1 out]
        n1093 = Wait (ms)(milliseconds to wait=w2468) -> ()  [unwired: 1 out]
        n1094 = call <vilib>:"Add State(s) to Queue__JKI_lib_State_Machine.vi"("State(s) in (\"\")"=w2474) -> ("States Out"=w2473:string)  [unwired: 14 in]
      }
      frame "---------- SysLog ----------" {
        # "Template Separator\n(You can make a copy of, or modify, this frame)"
        n1095 = call <vilib>:"Add State(s) to Queue__JKI_lib_State_Machine.vi"("State(s) in (\"\")"=w2479) -> ("States Out"=w2478:string)  [unwired: 14 in]
      }
      frame "SysLog: OpenLogFile" {
        # "Template Separator\n(You can make a copy of, or modify, this frame)"
        n1096 = call <vilib>:"Add State(s) to Queue__JKI_lib_State_Machine.vi"("State(s) in (\"\")"=w2484) -> ("States Out"=w2483:string)  [unwired: 14 in]
      }
      frame "---------- Graph ----------" {
        # "Template Separator\n(You can make a copy of, or modify, this frame)"
        n1097 = call <vilib>:"Add State(s) to Queue__JKI_lib_State_Machine.vi"("State(s) in (\"\")"=w2489) -> ("States Out"=w2488:string)  [unwired: 14 in]
      }
      frame "Graph: SetXMultiplier" {
        # "Set X multiplier of WF graphs\n(You can make a copy of, or modify, this frame)"
        n1098 = call "Digitizer1_FGV.vi"() -> ("error out"=w2493:errorcluster, "Read data"=w2494:refnum<k15>)  [unwired: 10 in]
        n1099 = property class="niScope"(reference=w2494, error in=w2493) -> ("Min Sample Rate"=w2492:dbl)  [unwired: 2 out]
        n1100 = Divide(x=1.0, y=w2492) -> (x/y=w2490:dbl)
        n1101 = property on="Channel 1" class="WFGraph (strict)"("XScale.Multiplier"=w2490) -> ()  [unwired: 2 in, 2 out]
        n1102 = property on="Channel 2" class="WFGraph (strict)"("XScale.Multiplier"=w2490) -> ()  [unwired: 2 in, 2 out]
        n1103 = property on="Channel 3" class="WFGraph (strict)"("XScale.Multiplier"=w2490) -> ()  [unwired: 2 in, 2 out]
        n1104 = call <vilib>:"Add State(s) to Queue__JKI_lib_State_Machine.vi"("State(s) in (\"\")"=w2499) -> ("States Out"=w2498:string)  [unwired: 14 in]
      }
      frame "Graph: AddCursors" {
        # "Add BG and DC cursor to all graphs\n(You can make a copy of, or modify, this frame)"
        n1105 = property on="Channel 1" class="WFGraph (strict)"() -> ("XScale.Multiplier"=w2506:dbl)  [unwired: 2 in, 2 out]
        n1106 = global read "GlobalVariables.vi" "DC Idx1"() -> (w2505:i32)
        n1107 = global read "GlobalVariables.vi" "DC Idx2"() -> (w2504:i32)
        n1108 = global read "GlobalVariables.vi" "BG Idx1"() -> (w2503:i32)
        n1109 = global read "GlobalVariables.vi" "BG Idx2"() -> (w2502:i32)
        n1110 = property on="Channel 2" class="WFGraph (strict)"() -> ("CrsrList"=w2514:T20)  [unwired: 2 in, 2 out]
        n1111 = property on="Channel 3" class="WFGraph (strict)"() -> ("CrsrList"=w2513:T20)  [unwired: 2 in, 2 out]
        n1112 = property on="Channel 1" class="WFGraph (strict)"(error in=w2508) -> ("CrsrList"=w2517:T20)  [unwired: 1 in, 2 out]
        n1113 = Build Array(w2505, w2504, w2503, w2502) -> (w2501:i32[])
        n1114 = Multiply(x=w2501, y=w2506) -> (x*y=w2500:dbl[])
        n1115 = for {
          tunnel: w2517 -> [w2529] mode=indexing
          tunnel: w2500 -> [w2525] mode=indexing
          tunnel: [w2528] -> w2516 mode=indexing
          tunnel: u32[] [6618880, 6618880, 16711680, 16711680] -> [w2524] mode=indexing
          tunnel: w2514 -> [w2527] mode=indexing
          tunnel: w2513 -> [w2526] mode=indexing
          tunnel: [w2523] -> w2512 mode=indexing
          tunnel: [w2522] -> w2511 mode=indexing
          n1116 = Bundle By Name(cluster=w2529, "Position.X"=w2525, "Color"=w2524) -> (w2528:T21)
          n1117 = Bundle By Name(cluster=w2527, "Position.X"=w2525, "Color"=w2524) -> (w2523:T21)
          n1118 = Bundle By Name(cluster=w2526, "Position.X"=w2525, "Color"=w2524) -> (w2522:T21)
        }
        n1119 = control-ref of="Channel 1"() -> (w2510:refnum<vi>)
        n1120 = property on="Channel 1" class="WFGraph (strict)"("CrsrList"=w2516) -> (error out=w2507:errorcluster)  [unwired: 2 in, 1 out]
        n1121 = property on="Channel 2" class="WFGraph (strict)"("CrsrList"=w2512) -> ()  [unwired: 2 in, 2 out]
        n1122 = property on="Channel 3" class="WFGraph (strict)"("CrsrList"=w2511) -> ()  [unwired: 2 in, 2 out]
        n1123 = call "UpdateCurserIdx(SubVI).vi"("error in (no error)"=w2507, "WaveformGraph in"=w2510) -> ("error out"=w2509:errorcluster)  [unwired: 9 in]
        n1124 = call <vilib>:"Add State(s) to Queue__JKI_lib_State_Machine.vi"("State(s) in (\"\")"=w2521) -> ("States Out"=w2520:string)  [unwired: 14 in]
      }
      frame "Graph: SaveCursorLoc" {
        # "Save cursor location to ini file\n(Save cursor location to system setting ini file)"
        n1125 = global read "GlobalVariables.vi" "DC Idx1"() -> (w2536:i32)
        n1126 = global read "GlobalVariables.vi" "DC Idx2"() -> (w2535:i32)
        n1127 = global read "GlobalVariables.vi" "BG Idx1"() -> (w2534:i32)
        n1128 = global read "GlobalVariables.vi" "BG Idx2"() -> (w2533:i32)
        n1129 = Bundle("DC Idx1"=w2536, "DC Idx2"=w2535, "BG Idx1"=w2534, "BG Idx2"=w2533) -> (w2532:T42)  [unwired: 1 in]
        n1130 = call "writeCursorConfigMain.vi"("error in (no error)"=w2530, "Cursor Locations"=w2532) -> ("error out"=w2531:errorcluster)  [unwired: 9 in]
        n1131 = call <vilib>:"Add State(s) to Queue__JKI_lib_State_Machine.vi"("State(s) in (\"\")"=w2540) -> ("States Out"=w2539:string)  [unwired: 14 in]
      }
      frame "---------- APD ----------" {
        # "Template Separator\n(You can make a copy of, or modify, this frame)"
        n1132 = call <vilib>:"Add State(s) to Queue__JKI_lib_State_Machine.vi"("State(s) in (\"\")"=w2545) -> ("States Out"=w2544:string)  [unwired: 14 in]
      }
      frame "APD: Initialize" {
        w2552 = enum16{"Read", "Write"}."Write" ("Operation (Read)")
        w2551 = refnum<class "APDClass.lvclass"> refnum  # APDClass.lvclass
        # "Initialize APD FGV\n(Initialized APD FGV for holding data)"
        n1133 = call "APD1FGV.vi"("Error In"=w2546, "Operation (Read)"=w2552, "APDClass in"=w2551) -> ("Error Out"=w2550:errorcluster)  [unwired: 7 in, 1 out]
        n1134 = call "APD2FGV.vi"("Error In"=w2546, "Operation (Read)"=w2552, "APDClass in"=w2551) -> ("Error Out"=w2549:errorcluster)  [unwired: 7 in, 1 out]
        n1135 = call "APD3FGV.vi"("Error In"=w2546, "Operation (Read)"=w2552, "APDClass in"=w2551) -> ("Error Out"=w2548:errorcluster)  [unwired: 7 in, 1 out]
        n1136 = Merge Errors(w2550, w2549, w2548) -> (w2547:errorcluster)
        n1137 = call <vilib>:"Add State(s) to Queue__JKI_lib_State_Machine.vi"("State(s) in (\"\")"=w2556) -> ("States Out"=w2555:string)  [unwired: 14 in]
      }
      frame "APD: LoadFromSerial" {
        w2565 = enum16{"Read", "Write"}."Write" ("Operation (Read)")
        # "Load APD data from tdms file\n(load and update FGV)"
        n1138 = call "readAPDSerial.vi"("Error In"=w2560) -> ("Error Out"=w2559:errorcluster, "output cluster"=w2558:T35)  [unwired: 9 in]
        n1139 = Unbundle By Name(w2558) -> ("Ch1APDSerial#"=w2573:string, "Ch2APDSerial#"=w2557:string, "Ch3APDSerial#"=w2572:string)
        n1140 = call "CreatFromSerialNumNoRaw.vi"("error in (no error)"=w2559, "APD Serial #"=w2557) -> ("error out"=w2568:errorcluster, "APDClass out"=w2569:refnum<class "APDClass.lvclass">)  [unwired: 8 in]
        n1141 = call "CreatFromSerialNumNoRaw.vi"("error in (no error)"=w2559, "APD Serial #"=w2572) -> ("error out"=w2566:errorcluster, "APDClass out"=w2567:refnum<class "APDClass.lvclass">)  [unwired: 8 in]
        n1142 = call "CreatFromSerialNumNoRaw.vi"("error in (no error)"=w2559, "APD Serial #"=w2573) -> ("error out"=w2570:errorcluster, "APDClass out"=w2571:refnum<class "APDClass.lvclass">)  [unwired: 8 in]
        n1143 = call "APD1FGV.vi"("Error In"=w2570, "Operation (Read)"=w2565, "APDClass in"=w2571) -> ("Error Out"=w2564:errorcluster)  [unwired: 7 in, 1 out]
        n1144 = call "APD2FGV.vi"("Error In"=w2568, "Operation (Read)"=w2565, "APDClass in"=w2569) -> ("Error Out"=w2562:errorcluster)  [unwired: 7 in, 1 out]
        n1145 = call "APD3FGV.vi"("Error In"=w2566, "Operation (Read)"=w2565, "APDClass in"=w2567) -> ("Error Out"=w2563:errorcluster)  [unwired: 7 in, 1 out]
        n1146 = Merge Errors(w2564, w2562, w2563) -> (w2561:errorcluster)
        n1147 = call <vilib>:"Add State(s) to Queue__JKI_lib_State_Machine.vi"("State(s) in (\"\")"=w2577) -> ("States Out"=w2576:string)  [unwired: 14 in]
      }
      frame "APD: UpdateCtrlVLimit" {
        w2595 = enum16{"Read", "Write"}."Read" ("Operation (Read)")
        # "Template Separator\n(You can make a copy of, or modify, this frame)"
        n1148 = call "APD1FGV.vi"("Error In"=w2592, "Operation (Read)"=w2595) -> ("Error Out"=w2593:errorcluster, "APDClass out"=w2594:refnum<class "APDClass.lvclass">)  [unwired: 8 in]
        n1149 = call "APD2FGV.vi"("Error In"=w2592, "Operation (Read)"=w2595) -> ("Error Out"=w2590:errorcluster, "APDClass out"=w2591:refnum<class "APDClass.lvclass">)  [unwired: 8 in]
        n1150 = call "APD3FGV.vi"("Error In"=w2592, "Operation (Read)"=w2595) -> ("Error Out"=w2588:errorcluster, "APDClass out"=w2589:refnum<class "APDClass.lvclass">)  [unwired: 8 in]
        n1151 = call-dynamic "ReadMaxCtrlV.vi"("error in (no error)"=w2593, "APDClass in"=w2594) -> ("error out"=w2583:errorcluster, "Numeric"=w2586:dbl)  [unwired: 7 in, 1 out]
        n1152 = call-dynamic "ReadMaxCtrlV.vi"("error in (no error)"=w2590, "APDClass in"=w2591) -> ("error out"=w2581:errorcluster, "Numeric"=w2585:dbl)  [unwired: 7 in, 1 out]
        n1153 = call-dynamic "ReadMaxCtrlV.vi"("error in (no error)"=w2588, "APDClass in"=w2589) -> ("error out"=w2579:errorcluster, "Numeric"=w2584:dbl)  [unwired: 7 in, 1 out]
        n1154 = property on="V 1" class="DigNum (strict)"(error in=w2583, "Maximum"=w2586) -> (error out=w2582:errorcluster)  [unwired: 1 in, 1 out]
        n1155 = property on="V 2" class="DigNum (strict)"(error in=w2581, "Maximum"=w2585) -> (error out=w2580:errorcluster)  [unwired: 1 in, 1 out]
        n1156 = property on="V 3" class="DigNum (strict)"(error in=w2579, "Maximum"=w2584) -> (error out=w2578:errorcluster)  [unwired: 1 in, 1 out]
        n1157 = Merge Errors(w2582, w2580, w2578) -> (w2587:errorcluster)
        n1158 = call <vilib>:"Add State(s) to Queue__JKI_lib_State_Machine.vi"("State(s) in (\"\")"=w2599) -> ("States Out"=w2598:string)  [unwired: 14 in]
      }
      frame "APD: GetGainLimits" {
        w2614 = enum16{"Read", "Write"}."Read" ("Operation (Read)")
        # "Template Separator\n(You can make a copy of, or modify, this frame)"
        n1159 = call "APD1FGV.vi"("Error In"=w2613, "Operation (Read)"=w2614) -> ("Error Out"=w2604:errorcluster, "APDClass out"=w2605:refnum<class "APDClass.lvclass">)  [unwired: 8 in]
        n1160 = call "APD2FGV.vi"("Error In"=w2613, "Operation (Read)"=w2614) -> ("Error Out"=w2611:errorcluster, "APDClass out"=w2612:refnum<class "APDClass.lvclass">)  [unwired: 8 in]
        n1161 = call "APD3FGV.vi"("Error In"=w2613, "Operation (Read)"=w2614) -> ("Error Out"=w2609:errorcluster, "APDClass out"=w2610:refnum<class "APDClass.lvclass">)  [unwired: 8 in]
        n1162 = call-dynamic "Read Gain Limits(Log).vi"("error in (no error)"=w2604, "APDClass in"=w2605) -> ("error out"=w2603:errorcluster, "GainLimits(Log)"=w2600:cluster{"GainMax":dbl, "GainMin":dbl})  [unwired: 7 in, 1 out]
        n1163 = call-dynamic "Read Gain Limits(Log).vi"("error in (no error)"=w2611, "APDClass in"=w2612) -> ("error out"=w2607:errorcluster, "GainLimits(Log)"=w2602:cluster{"GainMax":dbl, "GainMin":dbl})  [unwired: 7 in, 1 out]
        n1164 = call-dynamic "Read Gain Limits(Log).vi"("error in (no error)"=w2609, "APDClass in"=w2610) -> ("error out"=w2606:errorcluster, "GainLimits(Log)"=w2601:cluster{"GainMax":dbl, "GainMin":dbl})  [unwired: 7 in, 1 out]
        n1165 = global write "GlobalVariables.vi" "Ch1GainLim(Log)"(w2600) -> ()
        n1166 = global write "GlobalVariables.vi" "Ch2GainLim(Log)"(w2602) -> ()
        n1167 = global write "GlobalVariables.vi" "Ch3GainLim(Log)"(w2601) -> ()
        n1168 = Merge Errors(w2603, w2607, w2606) -> (w2608:errorcluster)
        n1169 = call <vilib>:"Add State(s) to Queue__JKI_lib_State_Machine.vi"("State(s) in (\"\")"=w2618) -> ("States Out"=w2617:string)  [unwired: 14 in]
      }
      frame "---------- EncoderDAQ ----------" {
        # "Template Separator\n(You can make a copy of, or modify, this frame)"
        n1170 = call <vilib>:"Add State(s) to Queue__JKI_lib_State_Machine.vi"("State(s) in (\"\")"=w2623) -> ("States Out"=w2622:string)  [unwired: 14 in]
      }
      frame "EncoderDAQ: Initialize" {
        w2636 = 388 items=["Start"=482, "Trigger"=483, "Pretrigger"=477, "Now"=481, "Read Pointer"=388] ("Fetch:Fetch Relative To")
        w2641 = T43 0 items=["AC", "DC", "Ground"] ("vertical coupling")
        # "Initilize encoder DAQ\n(You can make a copy of, or modify, this frame)"
        n1171 = call <instrlib>:"niScope Initialize With Options.vi"("resource name"="EncoderDAQ name", "reset device"=FALSE, "error in"=w2630) -> ("instrument handle"=w2648:refnum<k15>, "error out"=w2646:errorcluster)  [unwired: 11 in]
        n1172 = call <instrlib>:"niScope Configure Chan Characteristics.vi"("instrument handle"=w2648, "channels"="channels", "input impedance"="input impedance", "error in"=w2646) -> ("instrument handle out"=w2645:refnum<k15>, "error out"=w2644:errorcluster)  [unwired: 10 in]
        n1173 = call <instrlib>:"niScope Configure Vertical.vi"("instrument handle"=w2645, "vertical coupling"=w2641, "channels"="channels", "vertical range"="vertical range", "error in"=w2644) -> ("instrument handle out"=w2640:refnum<k15>, "error out"=w2639:errorcluster)  [unwired: 9 in]
        n1174 = call <instrlib>:"niScope Configure Horizontal Timing.vi"("instrument handle"=w2640, "min sample rate"="min sample rate", "error in"=w2639) -> ("instrument handle out"=w2637:refnum<k15>)  [unwired: 11 in, 1 out]
        n1175 = property class="niScope"(reference=w2637, "Start Trigger Source"="VAL_RTSI_0" ("Synchronization:Start Trigger (Acq. Arm): Source"), "Fetch Relative To"=w2636) -> (reference out=w2634:refnum<k15>, error out=w2633:errorcluster)  [unwired: 1 in]
        n1176 = call-poly <instrlib>:"niScope Configure Trigger (poly).vi"("instrument handle"=w2634, "error in"=w2633) -> ("instrument handle out"=w2632:refnum<k15>, "error out"=w2631:errorcluster)  [unwired: 12 in]
        n1177 = call <instrlib>:"niScope Commit.vi"("instrument handle"=w2632, "error in"=w2631) -> ("instrument handle out"=w2624:refnum<k15>, "error out"=w2627:errorcluster)  [unwired: 12 in]
        n1178 = Unbundle By Name(w2627) -> ("status"=w2626:bool)
        n1179 = Not(x=w2626) -> (.not. x?=w2625:bool)
        n1180 = Bundle By Name(cluster=w2628, "EncoderDAQ"=w2624, "System Status.Encoder"=w2625) -> (w2629:T19)
        n1181 = call <vilib>:"Add State(s) to Queue__JKI_lib_State_Machine.vi"("State(s) in (\"\")"=w2653) -> ("States Out"=w2652:string)  [unwired: 14 in]
      }
      frame "EncoderDAQ: Start" {
        # "Template Separator\n(You can make a copy of, or modify, this frame)"
        n1182 = Unbundle By Name(w2662) -> ("EncoderDAQ"=w2661:refnum<k15>)
        n1183 = call <instrlib>:"niScope Initiate Acquisition.vi"("instrument handle"=w2661, "error in"=w2658) -> ("error out"=w2656:errorcluster)  [unwired: 12 in, 1 out]
        n1184 = Generate User Event(priority (normal)=usereventprio."high priority", user event=w2660, event data cluster=TRUE ("event data"), error in=w2658) -> (error out=w2657:errorcluster)  [unwired: 1 out]
        n1185 = Merge Errors(w2657, w2656) -> (w2655:errorcluster)
        n1186 = call <vilib>:"Add State(s) to Queue__JKI_lib_State_Machine.vi"("State(s) in (\"\")"=w2665) -> ("States Out"=w2664:string)  [unwired: 14 in]
      }
      frame "EncoderDAQ: Abort" {
        # "Template Separator\n(You can make a copy of, or modify, this frame)"
        n1187 = Unbundle By Name(w2667) -> ("EncoderDAQ"=w2666:refnum<k15>)
        n1188 = call <instrlib>:"niScope Abort.vi"("instrument handle"=w2666, "error in"=w2668) -> ("error out"=w2669:errorcluster)  [unwired: 12 in, 1 out]
        n1189 = call <vilib>:"Add State(s) to Queue__JKI_lib_State_Machine.vi"("State(s) in (\"\")"=w2672) -> ("States Out"=w2671:string)  [unwired: 14 in]
      }
      frame "EncoderDAQ: Close" {
        # "Close Encoder DAQ\n(You can make a copy of, or modify, this frame)"
        n1190 = Unbundle By Name(w2673) -> ("EncoderDAQ"=w2678:refnum<k15>)
        n1191 = call <instrlib>:"niScope Close.vi"("instrument handle"=w2678, "error in"=w2677) -> ("error out"=w2676:errorcluster)  [unwired: 13 in]
        n1192 = Unbundle By Name(w2676) -> ("status"=w2675:bool)
        n1193 = Bundle By Name(cluster=w2673, "System Status.Encoder"=w2675) -> (w2674:T19)
        n1194 = call <vilib>:"Add State(s) to Queue__JKI_lib_State_Machine.vi"("State(s) in (\"\")"=w2681) -> ("States Out"=w2680:string)  [unwired: 14 in]
      }
      frame "---------- TDMS ----------" {
        # "Template Separator\n(You can make a copy of, or modify, this frame)"
        n1195 = call <vilib>:"Add State(s) to Queue__JKI_lib_State_Machine.vi"("State(s) in (\"\")"=w2686) -> ("States Out"=w2685:string)  [unwired: 14 in]
      }
      frame "TDMS: OpenFile" {
        w2694 = FALSE ("disable buffering? (T)")
        # "Open File to stream data\n(You can make a copy of, or modify, this frame)"
        n1196 = Unbundle By Name(w2699) -> ("Pathes.DataPath"=w2698:path, "CaseID"=w2697:string, "IDs.RunID"=w2688:i8)
        n1197 = Increment(x=w2688) -> (x+1=w2687:i8)
        n1198 = Format Value(string ("")=w2697, format string="_%02d", value (0)=w2687) -> (output string=w2701:string)
        n1199 = Build Path(base path=w2698, name or relative path=w2701) -> (appended path=w2696:path)
        n1200 = TDMS Advanced Open(4:w2694, 6:w2694, 8:w2689, 10:T12."open or create" ("operation (0:open)"), 11:w2696) -> (0:w2691:errorcluster, 3:w2692:refnum<k34>)  [unwired: 1 out]
        n1201 = call "TDMS_FGV.vi"("error in (no error)"=w2691, "Operation (Read)"=enum16{"Write", "Read"}."Write", "tdms file in"=w2692) -> ("error out"=w2690:errorcluster)  [unwired: 7 in, 1 out]
        n1202 = call <vilib>:"Add State(s) to Queue__JKI_lib_State_Machine.vi"("State(s) in (\"\")"=w2704) -> ("States Out"=w2703:string)  [unwired: 14 in]
      }
      frame "TDMS: Config" {
        w2711 = i16 0  # I16
        # "Config TDMS file for streaming data\n(You can make a copy of, or modify, this frame)"
        n1203 = Unbundle By Name(w2706) -> ("TDMS group name"=w2705:string)
        n1204 = call "TDMS_FGV.vi"("error in (no error)"=w2707, "Operation (Read)"=enum16{"Write", "Read"}."Read") -> ("error out"=w2713:errorcluster, "tdms file out"=w2714:refnum<k34>)  [unwired: 8 in]
        n1205 = call "FLImDAQ_FGV.vi"("error in (no error)"=w2707) -> ("Read data"=w2710:T6)  [unwired: 9 in, 1 out]
        n1206 = Unbundle By Name(w2710) -> ("min record length"=w2709:i32)
        n1207 = TDMS Set Channel Information(4:w2709, 6:w2711, 7:enum16{"non-interleaved", "interleaved"}."non-interleaved" ("data layout (0:non-interleaved)"), 8:w2713, 9:string[] ["channel 1", "channel 2", "channel 3"] ("channel name(s)"), 10:w2705, 11:w2714) -> (0:w2708:errorcluster)  [unwired: 1 out]
        n1208 = call <vilib>:"Add State(s) to Queue__JKI_lib_State_Machine.vi"("State(s) in (\"\")"=w2719) -> ("States Out"=w2718:string)  [unwired: 14 in]
      }
      frame "TDMS: SaveMetaData" {
        # "Save metadata\n(You can make a copy of, or modify, this frame)"
        n1209 = call "Digitizer1_FGV.vi"() -> ("error out"=w2730:errorcluster, "Read data"=w2740:refnum<k15>)  [unwired: 10 in]
        n1210 = Unbundle By Name(w2742) -> ("TDMS group name"=w2722:string)
        n1211 = property class="niScope"(reference=w2740, error in=w2730) -> ("Actual Sample Rate"=w2739:dbl, "Actual Record Length"=w2738:i32, "Vertical Range"=w2737:dbl, "Vertical Offset"=w2736:dbl)  [unwired: 2 out]
        n1212 = call "TDMS_FGV.vi"("error in (no error)"=w2720, "Operation (Read)"=enum16{"Write", "Read"}."Read") -> ("error out"=w2741:errorcluster, "tdms file out"=w2743:refnum<k34>)  [unwired: 8 in]
        n1213 = Build Array(w2739, w2738, w2737, w2736) -> (w2734:dbl[])
        n1214 = TDMS Set Properties(5:w2734, 7:string[] ["ActualSampleRate1", "ActualRecordLength1", "VerticalRange1", "VerticalOffset1"], 8:w2741, 10:w2722, 11:w2743) -> (2:w2732:string, 3:w2733:refnum<k34>)  [unwired: 1 in, 2 out]
        n1215 = call "Digitizer2_FGV.vi"() -> ("error out"=w2729:errorcluster, "Read data"=w2731:refnum<k15>)  [unwired: 10 in]
        n1216 = property class="niScope"(reference=w2731, error in=w2729) -> ("Actual Sample Rate"=w2728:dbl, "Actual Record Length"=w2727:i32, "Vertical Range"=w2726:dbl, "Vertical Offset"=w2725:dbl)  [unwired: 2 out]
        n1217 = Build Array(w2728, w2727, w2726, w2725) -> (w2723:dbl[])
        n1218 = TDMS Set Properties(5:w2723, 7:string[] ["ActualSampleRate2", "ActualRecordLength2", "VerticalRange2", "VerticalOffset2"], 10:w2732, 11:w2733) -> (0:w2721:errorcluster)  [unwired: 2 in, 3 out]
        n1219 = call <vilib>:"Add State(s) to Queue__JKI_lib_State_Machine.vi"("State(s) in (\"\")"=w2747) -> ("States Out"=w2746:string)  [unwired: 14 in]
      }
      frame "TDMS: saveCtrlV" {
        w2756 = "CtrlV"
        w2755 = enum16{"write", "read"}."read" ("action (write)")
        # "Save control voltage\n(You can make a copy of, or modify, this frame)"
        n1220 = Unbundle By Name(w2769) -> ("TDMS group name"=w2768:string)
        n1221 = call "TDMS_FGV.vi"("error in (no error)"=w2751, "Operation (Read)"=enum16{"Write", "Read"}."Read") -> ("error out"=w2770:errorcluster, "tdms file out"=w2771:refnum<k34>)  [unwired: 8 in]
        n1222 = call "V1FGV.vi"("Error In"=w2751, "action (write)"=w2755) -> ("Error Out"=w2753:errorcluster, "V1 out"=w2766:dbl)  [unwired: 8 in]
        n1223 = TDMS Set Properties(5:w2766, 7:w2756, 8:w2770, 9:"channel 1", 10:w2768, 11:w2771) -> (0:w2764:errorcluster, 2:w2763:string, 3:w2765:refnum<k34>)  [unwired: 1 out]
        n1224 = call "V2FGV.vi"("Error In"=w2753, "action(write)"=w2755) -> ("Error Out"=w2752:errorcluster, "V2 out"=w2761:dbl)  [unwired: 8 in]
        n1225 = TDMS Set Properties(5:w2761, 7:w2756, 8:w2764, 9:"channel 2", 10:w2763, 11:w2765) -> (0:w2757:errorcluster, 2:w2759:string, 3:w2760:refnum<k34>)  [unwired: 1 out]
        n1226 = call "V3FGV.vi"("Error In"=w2752, "action(write)"=w2755) -> ("Error Out"=w2750:errorcluster, "V3 out"=w2754:dbl)  [unwired: 8 in]
        n1227 = TDMS Set Properties(5:w2754, 7:w2756, 8:w2757, 9:"channel 3", 10:w2759, 11:w2760) -> (0:w2749:errorcluster)  [unwired: 3 out]
        n1228 = Merge Errors(w2750, w2749) -> (w2748:errorcluster)
        n1229 = call <vilib>:"Add State(s) to Queue__JKI_lib_State_Machine.vi"("State(s) in (\"\")"=w2775) -> ("States Out"=w2774:string)  [unwired: 14 in]
      }
      frame "TDMS: StartStreaming" {
        # "Start TDMS streaming loop\n(You can make a copy of, or modify, this frame)"
        n1230 = Generate User Event(priority (normal)=usereventprio."normal priority", user event=w2780, event data cluster=TRUE ("event data"), error in=w2777) -> (error out=w2778:errorcluster)  [unwired: 1 out]
        n1231 = call <vilib>:"Add State(s) to Queue__JKI_lib_State_Machine.vi"("State(s) in (\"\")"=w2784) -> ("States Out"=w2783:string)  [unwired: 14 in]
      }
      frame "---------- EncoderFile ----------" {
        # "Template Separator\n(You can make a copy of, or modify, this frame)"
        n1232 = call <vilib>:"Add State(s) to Queue__JKI_lib_State_Machine.vi"("State(s) in (\"\")"=w2789) -> ("States Out"=w2788:string)  [unwired: 14 in]
      }
      frame "EncoderFile: Open" {
        w2805 = FALSE ("disable buffering? (T)")
        # "Open Encoder TDMS file\n(You can make a copy of, or modify, this frame)"
        n1233 = Unbundle By Name(w2802) -> ("Pathes.DataPath"=w2808:path, "CaseID"=w2807:string, "IDs.RunID"=w2804:i8)
        n1234 = Increment(x=w2804) -> (x+1=w2803:i8)
        n1235 = Format Value(string ("")=w2807, format string="_%02d", value (0)=w2803) -> (output string=w2797:string)
        n1236 = Concatenate Strings(w2797, "_Encoder" ("string")) -> (w2796:string)
        n1237 = Build Path(base path=w2808, name or relative path=w2796) -> (appended path=w2795:path)
        n1238 = TDMS Advanced Open(4:w2805, 6:w2805, 8:w2799, 10:T12."open or create" ("operation (0:open)"), 11:w2795) -> (0:w2793:errorcluster, 3:w2801:refnum<k34>)  [unwired: 1 out]
        n1239 = call "EncoderTDMS_Path.vi"("error in (no error)"=w2793, "Operation (Read)"=enum16{"Write", "Read"}."Write", "PathIn"=w2795) -> ("error out"=w2792:errorcluster)  [unwired: 7 in, 1 out]
        n1240 = call "EncoderTDMS_FGV.vi"("error in (no error)"=w2793, "Operation (Read)"=enum16{"Write", "Read"}."Write", "tdms file in"=w2801) -> ("error out"=w2791:errorcluster)  [unwired: 7 in, 1 out]
        n1241 = Merge Errors(w2792, w2791) -> (w2790:errorcluster)
        n1242 = call <vilib>:"Add State(s) to Queue__JKI_lib_State_Machine.vi"("State(s) in (\"\")"=w2812) -> ("States Out"=w2811:string)  [unwired: 14 in]
      }
      frame "EncoderFile: SaveMetaData" {
        # "Save Encoder DAQ setting\n(You can make a copy of, or modify, this frame)"
        n1243 = Unbundle By Name(w2826) -> ("EncoderDAQ"=w2825:refnum<k15>)
        n1244 = property class="niScope"(reference=w2825, error in=w2819) -> ("Actual Sample Rate"=w2822:dbl)  [unwired: 2 out]
        n1245 = call "EncoderTDMS_FGV.vi"("error in (no error)"=w2819) -> ("error out"=w2817:errorcluster, "tdms file out"=w2818:refnum<k34>)  [unwired: 9 in]
        n1246 = Build Array(w2822) -> (w2821:dbl[])
        n1247 = Get Date/Time In Seconds() -> (seconds since 1Jan1904=w2815:timestamp)
        n1248 = TDMS Set Properties(5:w2815, 7:"DateTime", 8:w2817, 11:w2818) -> (0:w2813:errorcluster, 3:w2814:refnum<k34>)  [unwired: 2 in, 2 out]
        n1249 = TDMS Set Properties(5:w2821, 7:string[] ["SamplingRate (S/s)"] ("property names"), 8:w2813, 10:"Encoder" ("group name"), 11:w2814) -> (0:w2820:errorcluster)  [unwired: 1 in, 3 out]
        n1250 = call <vilib>:"Add State(s) to Queue__JKI_lib_State_Machine.vi"("State(s) in (\"\")"=w2829) -> ("States Out"=w2828:string)  [unwired: 14 in]
      }
      frame "---------- Temp ----------" {
        # "Template Separator\n(You can make a copy of, or modify, this frame)"
        n1251 = call <vilib>:"Add State(s) to Queue__JKI_lib_State_Machine.vi"("State(s) in (\"\")"=w2834) -> ("States Out"=w2833:string)  [unwired: 14 in]
      }
    }
    n1252 = Not(x=w80) -> (.not. x?=w79:bool)
    n1253 = local write "ML?"(w79) -> ()
    "ML?" <- TRUE ("main loop running?")
  }
  n1254 = while {
    tunnel: w12 -> [w2839]
    tunnel: w17 -> [w2837]
    tunnel: [w2836] -> w16
    stop <- w2838 stop-if-true
    # "Encoder Aquisition Loop"
    n1255 = event shown="[1] <StartEncoderDataStream>: User Event" {
      selector: w2837 -> [_ _]
      dyn-events: [_ _] -> w2836
      timeout: 20 -> [_ _]
      tunnel: w2839 -> [w2841 _]
      tunnel: [w2840 _] -> w2838
      event Timeout {
        n1256 = event-data() -> ()  [unwired: 1 in, 3 out]
        n1257 = Get Queue Status(queue=w2841) -> (error out=w2840:errorcluster)  [unwired: 2 in, 7 out]
      }
      event User Event {
        n1258 = event-data() -> ()  [unwired: 1 in, 5 out]
        n1259 = local read "Skip Data Save?"() -> (w2842:bool)
        n1260 = local read "EncoderDAQ name"() -> (w2856:refnum<k15>)
        n1261 = local read "min sample rate"() -> (w2854:dbl)
        n1262 = local read "channels"() -> (w2852:string)
        n1263 = property class="niScope"(reference=w2856, "Active Channel"=w2852) -> (reference out=w2855:refnum<k15>, error out=w2850:errorcluster, "Vertical Range"=w2851:dbl)  [unwired: 1 in]
        n1264 = Multiply(x=w2854, y="EncoderSampleInterval(s)") -> (x*y=w2848:dbl)
        n1265 = case shown="False" w2842 {
          tunnel: w2848 -> [w2863 _]
          tunnel: [w2862 _] -> w2847
          tunnel: [w2861 errorcluster {"status"=FALSE, "code"=0, "source"=""} ("error out")] -> w2845
          frame False {
            n1266 = call "EncoderTDMS_FGV.vi"() -> ("error out"=w2860:errorcluster, "tdms file out"=w2867:refnum<k34>)  [unwired: 10 in]
            n1267 = TDMS Set Channel Information(4:w2863, 6:i8 0, 8:w2860, 9:string[] ["RawDataI8"] ("channel name(s)"), 10:"Encoder" ("group name"), 11:w2867) -> (0:w2861:errorcluster, 3:w2862:refnum<k34>)  [unwired: 1 in]
          }
          frame True {
          }
        }
        n1268 = while {
          tunnel: w2855 -> [w2891]
          tunnel: w2848 -> [w2890]
          tunnel: w2852 -> [w2889]
          tunnel: w2851 -> [w2887]
          tunnel: w2850 -> [w2886]
          tunnel: [w2885] -> w2849 mode=concatenating
          shift-right: [w2875] -> w2844
          shift-left: w2845 -> [w2876]
          shift-right: [w2870] -> _
          shift-left: u32 0 -> [w2872]
          tunnel: w2847 -> [w2878]
          tunnel: [w2877] -> w2846
          tunnel: w2842 -> [w2869]
          stop <- w2882 stop-if-true
          n1269 = call-poly <instrlib>:"niScope Fetch (poly).vi"("error in"=w2886, "numSamples"=w2890, "channels"=w2889, "instrument handle"=w2891) -> ("error out"=w2884:errorcluster, "wfm"=w2874:i8[], "wfm info"=w2873:T44)  [unwired: 4 in, 1 out]
          n1270 = local read "aquisition loop Error Out"() -> (w2883:errorcluster)
          n1271 = case shown="False" w2869 {
            tunnel: w2878 -> [w2896 w2898]
            tunnel: [w2895 w2898] -> w2877
            tunnel: w2876 -> [w2894 w2897]
            tunnel: [w2893 w2897] -> w2875
            tunnel: w2874 -> [w2892 _]
            frame False {
              n1272 = TDMS Advanced Synchronous Write(8:w2894, 10:w2892, 11:w2896) -> (0:w2893:errorcluster, 3:w2895:refnum<k34>)
            }
            frame True {
            }
          }
          n1273 = Power Of 2(x=i16 8) -> (2^x=w2880:dbl)
          n1274 = Unbundle By Name(w2873) -> ("actualSamples"=w2871:i32)
          n1275 = Divide(x=w2874, y=w2880) -> (x/y=w2888:dbl[])
          n1276 = Multiply(x=w2888, y=w2887) -> (x*y=w2885:dbl[])
          "EncoderGraph" <- w2885
          n1277 = Merge Errors(w2884, w2883) -> (w2882:errorcluster)
          n1278 = Add(x=w2872, y=w2871) -> (x+y=w2870:u32)
          "EncoderDataLength" <- w2870
          n1279 = Wait (ms)(milliseconds to wait=u32 200) -> ()  [unwired: 1 out]
        }
        n1280 = local write "EncoderGraph"(w2849) -> ()
        n1281 = case shown="False" w2842 {
          tunnel: w2846 -> [w2859 _]
          tunnel: w2844 -> [w2858 _]
          frame False {
            n1282 = TDMS Advanced Close(8:w2858, 11:w2859) -> (0:w2857:errorcluster)  [unwired: 2 in, 1 out]
            n1283 = call <vilib>:"Simple Error Handler.vi"("error in (no error)"=w2857) -> ()  [unwired: 4 in, 5 out]
          }
          frame True {
          }
        }
      }
    }
  }
  n1284 = while {
    tunnel: w12 -> [w2902]
    tunnel: w8 -> [w2901]
    tunnel: [w2900] -> w6
    tunnel: w5 -> [w2899]
    stop <- w2903 stop-if-true
    # "Streaming Ch1 and 2 Data to Disk Loop"
    n1285 = event shown="[1] <StartDataStream>: User Event" {
      selector: w2901 -> [_ _]
      dyn-events: [_ _] -> w2900
      timeout: 20 -> [_ _]
      tunnel: [w2906 _] -> w2903
      tunnel: w2902 -> [w2905 w2915]
      tunnel: w2899 -> [_ w2910]
      event Timeout {
        n1286 = event-data() -> ()  [unwired: 1 in, 3 out]
        n1287 = Get Queue Status(queue=w2905) -> (error out=w2906:errorcluster)  [unwired: 2 in, 7 out]
      }
      event User Event {
        w2914 = 2000  # timeout in ms
        n1288 = event-data() -> ()  [unwired: 1 in, 5 out]
        n1289 = call "TDMS_FGV.vi"() -> ("error out"=w2907:errorcluster, "tdms file out"=w2913:refnum<k34>)  [unwired: 10 in]
        n1290 = while {
          tunnel: w2915 -> [w2938]
          tunnel: w2914 -> [w2934]
          tunnel: w2913 -> [w2921]
          tunnel: [w2919] -> w2912
          tunnel: [w2920] -> w2911
          tunnel: w2910 -> [w2935]
          shift-right: [w2924] -> w2908
          shift-left: 0 -> [w2925]
          tunnel: w2907 -> [w2916]
          stop <- w2927 stop-if-true
          # "Stream data to disk"
          n1291 = Dequeue Element(queue=w2938, timeout in ms (-1)=w2934, error in (no error)=w2916) -> (element=w2937:i16[][], timed out?=w2931:bool, error out=w2933:errorcluster)  [unwired: 1 out]
          n1292 = Dequeue Element(queue=w2935, timeout in ms (-1)=w2934, error in (no error)=w2916) -> (element=w2929:i16[][], timed out?=w2930:bool, error out=w2932:errorcluster)  [unwired: 1 out]
          n1293 = Merge Errors(w2933, w2932) -> (w2923:errorcluster)
          n1294 = call "SeperateChanDataI16.vi"("Input (Ch1&2)"=w2937) -> ("Ch1"=w2926:i16[][], "Ch2"=w2936:i16[][])
          n1295 = call "SeperateChanDataI16.vi"("Input (Ch1&2)"=w2929) -> ("Ch1"=w2928:i16[][])  [unwired: 1 out]
          n1296 = Or(x=w2931, y=w2930) -> (x .or. y?=w2927:bool)
          n1297 = for {
            tunnel: w2926 -> [w2943] mode=indexing
            tunnel: w2936 -> [w2942] mode=indexing
            tunnel: w2928 -> [w2941] mode=indexing
            tunnel: [w2940] -> w2918
            tunnel: [w2939] -> w2922 mode=concatenating
            i -> [w2940]
            n1298 = Build Array (concatenate)(w2943, w2942, w2941) -> (w2939:i16[])
          }
          n1299 = Increment(x=w2918) -> (x+1=w2917:i32)
          n1300 = Add(x=w2917, y=w2925) -> (x+y=w2924:i32)
          "WF saved" <- w2924
          n1301 = TDMS Advanced Synchronous Write(8:w2923, 10:w2922, 11:w2921) -> (0:w2920:errorcluster, 3:w2919:refnum<k34>)
        }
        n1302 = local write "WF saved"(w2908) -> ()
        n1303 = TDMS Advanced Close(8:w2911, 11:w2912) -> ()  [unwired: 2 in, 2 out]
      }
    }
  }
  n1304 = disable-structure "Diagram Disable Structure" shown="Disabled" {
    frame Disabled {
      w2944 = T45 {"Horizontal"=500, "Vertical"=100}  # Top Left Corner
      n1305 = Control Help Window(0:w2944, 1:TRUE ("Show")) -> ()
      n1306 = call <vilib>:"TDMS - File Viewer.vi"() -> ()  [unwired: 6 in, 2 out]
    }
    frame Enabled {
    }
  }
  n1307 = while {
    tunnel: w12 -> [w2958]
    tunnel: w55 -> [w2957]
    tunnel: [w2956] -> w63
    tunnel: w13 -> [w2955]
    tunnel: [w2954] -> w59
    tunnel: w47 -> [w2952]
    tunnel: w5 -> [w2951]
    tunnel: w44 -> [w2946]
    stop <- w2949 stop-if-true
    # "acquire data and send it to processing loop"
    # "Data Aquisition Loop"
    n1308 = event shown="[1] <Start digitizer>: User Event" {
      selector: w2957 -> [_ _]
      dyn-events: [_ _] -> w2956
      timeout: 20 -> [_ _]
      tunnel: w2958 -> [w2964 w2977]
      tunnel: [w2959 _] -> w2949
      tunnel: w2955 -> [w2963 w2983]
      tunnel: [w2963 w2982] -> w2954
      tunnel: w2952 -> [_ w2980]
      tunnel: w2951 -> [w2962 w2976]
      tunnel: w2946 -> [_ w2974]
      event Timeout {
        # "use queue to stop data loop\nwhen queue ref is released, error will stop this loop"
        n1309 = event-data() -> ()  [unwired: 1 in, 3 out]
        n1310 = Get Queue Status(queue=w2964) -> (error out=w2961:errorcluster)  [unwired: 2 in, 7 out]
        n1311 = Get Queue Status(queue=w2962) -> (error out=w2960:errorcluster)  [unwired: 2 in, 7 out]
        n1312 = Merge Errors(w2961, w2960) -> (w2959:errorcluster)
      }
      event User Event {
        w2981 = enum16{"Write", "Read"}."Read" ("Operation")
        n1313 = event-data() -> ("Time"=→"RunStartTime":u32)  [unwired: 1 in, 3 out]
        n1314 = call "Digitizer2_FGV.vi"("Operation (Read)"=w2981) -> ("Read data"=w2969:refnum<k15>)  [unwired: 9 in, 1 out]
        n1315 = call "Digitizer1_FGV.vi"("Operation (Read)"=w2981) -> ("Read data"=w2973:refnum<k15>)  [unwired: 9 in, 1 out]
        n1316 = property on="Property Node" class="niScope"(reference=w2973) -> (reference out=w2972:refnum<k15>, "Vertical Range"=→"Vertical Range 1":dbl, "Vertical Offset"=→"Vertical Offset 1":dbl)  [unwired: 1 in, 1 out]
        n1317 = property on="Property Node" class="niScope"(reference=w2969) -> (reference out=w2968:refnum<k15>, "Vertical Range"=→"Vertical Range 2":dbl, "Vertical Offset"=→"Vertical Offset 2":dbl)  [unwired: 1 in, 1 out]
        n1318 = call "FLImDAQ_FGV.vi"() -> ("Read data"=w2979:T6)  [unwired: 10 in, 1 out]
        n1319 = Unbundle By Name(w2979) -> ("Waveform to Avg"=w2978:i16)
        n1320 = while {
          tunnel: w2983 -> [w3033]
          tunnel: [w3032] -> w2982
          tunnel: w2968 -> [w3026]
          tunnel: w2972 -> [w3025]
          tunnel: w2980 -> [w3024]
          shift-right: [w3003] -> _
          shift-left: u32 0 ("millisecond timer value") -> [w3023]
          tunnel: w2978 -> [w3021]
          tunnel: w2977 -> [w3019]
          tunnel: w2976 -> [w3018]
          tunnel: w2974 -> [w3011]
          i -> [w3004]
          stop <- w2984 stop-if-true
          w2985 = 2 ("length")
          w2986 = 0 ("index")
          w3015 = enum16{"write", "read"}."read" ("action")
          # "enqueue V"
          # "enqueue ch3 data"
          # "enqueue ch1&2 data"
          # "acquire ch3"
          # "acquire ch1&2"
          # "send data for processing"
          n1321 = call <userlib>:"Tick Count (ms)__ogtk.vi"() -> ("error out"=w2996:errorcluster, "millisecond timer value"=w2994:u32)  [unwired: 10 in]
          n1322 = Multiply(x=w3021, y=w3004) -> (x*y=w3000:i32)
          "Fetch Record #" <- w3000
          n1323 = property on="Property Node" class="niScope"(reference=w3026, error in=w2996, "Fetch Record Number"=w3000) -> (reference out=w3030:refnum<k15>, error out=w3027:errorcluster, "Records Done"=w3001:i32)
          n1324 = property on="Property Node" class="niScope"(reference=w3025, error in=w2996, "Fetch Record Number"=w3000) -> (reference out=w3037:refnum<k15>, error out=w3036:errorcluster, "Records Done"=w3010:i32)
          n1325 = Subtract(x=w3001, y=w3000) -> (x-y=→"Record Backlog 2":i32)
          n1326 = Subtract(x=w3010, y=w3000) -> (x-y=→"Record Backlog 1":i32)
          n1327 = call-poly <instrlib>:"niScope Fetch (poly).vi"("timeout"=1.0, "error in"=w3027, "channels"="0,1", "instrument handle"=w3030) -> ("error out"=w2997:errorcluster, "wfm"=w2988:i16[][])  [unwired: 4 in, 2 out]
          n1328 = call-poly <instrlib>:"niScope Fetch (poly).vi"("timeout"=1.0, "error in"=w3036, "channels"="0,1", "instrument handle"=w3037) -> ("error out"=w2998:errorcluster, "wfm"=w2990:i16[][])  [unwired: 4 in, 2 out]
          n1329 = Merge Errors(w2998, w2997) -> (w2992:errorcluster)
          n1330 = Tick Count (ms)() -> (millisecond timer value=w3003:u32)
          n1331 = call <userlib>:"Tick Count (ms)__ogtk.vi"("error in (no error)"=w2992) -> ("error out"=w2991:errorcluster, "millisecond timer value"=w2995:u32)  [unwired: 9 in]
          n1332 = Subtract(x=w3003, y=w3023) -> (x-y=→"Aquisition loop timing(ms)":u32)
          n1333 = Subtract(x=w2995, y=w2994) -> (x-y=→"DataTransferTime":u32)
          n1334 = Enqueue Element(queue=w3019, element=w2990, error in (no error)=w2991) -> (error out=w3009:errorcluster)  [unwired: 1 in, 2 out]
          n1335 = Enqueue Element(queue=w3018, element=w2988, error in (no error)=w3009) -> (error out=w3006:errorcluster)  [unwired: 1 in, 2 out]
          n1336 = Array Subset(array=w2990, index (row)=w2986, length (row)=w2985) -> (w2989:i16[][])  [unwired: 2 in]
          n1337 = Array Subset(array=w2988, index (row)=w2986, length (row)=w2985) -> (w2987:i16[][])  [unwired: 2 in]
          n1338 = call "V1FGV.vi"("Error In"=w3006, "action (write)"=w3015) -> ("Error Out"=w3017:errorcluster, "V1 out"=w3014:dbl)  [unwired: 8 in]
          n1339 = call "V2FGV.vi"("Error In"=w3017, "action(write)"=w3015) -> ("Error Out"=w3016:errorcluster, "V2 out"=w3013:dbl)  [unwired: 8 in]
          n1340 = call "V3FGV.vi"("Error In"=w3016, "action(write)"=w3015) -> ("Error Out"=w3007:errorcluster, "V3 out"=w3012:dbl)  [unwired: 8 in]
          n1341 = Bundle("V1 out"=w3014, "V2 out"=w3013, "V3 out"=w3012) -> (w3008:T46)  [unwired: 1 in]
          n1342 = Bundle(w3004, w2989, w2987, w3008) -> (w3020:T47)  [unwired: 1 in]
          n1343 = Enqueue Element(queue=w3011, element=w3008, error in (no error)=w3007) -> (error out=w3005:errorcluster)  [unwired: 1 in, 2 out]
          n1344 = Send Notification(notification=w3020, notifier=w3033, error in (no error)=w3005) -> (notifier out=w3032:refnum<notifier>, error out=w3002:errorcluster)
          n1345 = case shown="Error .." w3002 {
            selector: w3002 -> [w3038 w3039]
            tunnel: w3024 -> [_ w3042]
            tunnel: [w3038 w3039] -> w2984
            frame No Error {
            }
            frame Error {
              # "Send user event to signal aquisition has stoped"
              n1346 = Generate User Event(priority (normal)=usereventprio."high priority", user event=w3042, event data cluster=TRUE ("event data")) -> ()  [unwired: 1 in, 2 out]
            }
          }
          "aquisition loop Error Out" <- w2984
          "Auisition Loop idx" <- w3004
        }
      }
    }
    n1347 = Unbundle By Name(w2949) -> ("status"=w2948:bool)
    n1348 = Not(x=w2948) -> (.not. x?=w2947:bool)
    n1349 = local write "Aq Loop?"(w2947) -> ()
    "Aq Loop?" <- TRUE ("Aq L?")
  }
  n1350 = while {
    tunnel: w13 -> [w3053]
    shift-right: [w3044] -> _
    shift-left: w30 -> [w3051]
    shift-right: [w3046] -> _
    shift-left: w30 -> [w3045]
    i -> [w3047]
    stop <- w3048 stop-if-true
    # "Data display loop(30Hz)"
    n1351 = Wait on Notification(notifier=w3053, ignore previous (F)=FALSE) -> (notification=w3049:T10, error out=w3048:errorcluster)  [unwired: 2 in, 2 out]
    n1352 = Tick Count (ms)() -> (millisecond timer value=w3044:u32)
    n1353 = Subtract(x=w3044, y=w3051) -> (x-y=→"display loop timing(ms)":u32)
    n1354 = case shown="No Error" w3048 {
      tunnel: w3049 -> [w3121 _]
      tunnel: w3045 -> [w3102 w3177]
      tunnel: [w3104 w3177] -> w3046
      tunnel: w3044 -> [w3101 _]
      frame No Error {
        w3069 = u32 16744512 ("Plot.Plot Color")
        w3070 = u32 1 ("Active Plot")
        w3118 = 0 ("index (row)")
        n1355 = Subtract(x=w3101, y=w3102) -> (x-y=w3103:u32)
        n1356 = local read "Vertical Range 1"() -> (w3058:dbl)
        n1357 = Unbundle(w3121) -> ("CH1&2"=w3055:i16[][], "CH3"=w3059:i16[][], "V cluster"=w3107:cluster{"V1":dbl, "V2":dbl, "V3":dbl})  [unwired: 1 out]
        n1358 = Power Of 2(x=i16 16) -> (2^x=w3054:dbl)
        n1359 = Unbundle By Name(w3107) -> ("V1"=w3098:dbl, "V2"=w3096:dbl, "V3"=w3094:dbl)
        n1360 = Divide(x=w3055, y=w3054) -> (x/y=w3064:dbl[][])
        n1361 = Divide(x=w3059, y=w3054) -> (x/y=w3061:dbl[][])
        n1362 = local read "Vertical Offset 1"() -> (w3057:dbl)
        n1363 = Multiply(x=w3058, y=w3064) -> (x*y=w3063:dbl[][])
        n1364 = Multiply(x=w3058, y=w3061) -> (x*y=w3060:dbl[][])
        n1365 = Add(x=w3057, y=w3063) -> (x+y=w3062:dbl[][])
        n1366 = Add(x=w3057, y=w3060) -> (x+y=w3056:dbl[][])
        n1367 = call "CtrlVtoGain.vi"("CtrlV(V)"=w3098, "Channel"=enum16{"Ch1", "Ch2", "Ch3"}."Ch1") -> ("Gain"=w3092:dbl)  [unwired: 8 in, 1 out]
        n1368 = call "CtrlVtoGain.vi"("CtrlV(V)"=w3096, "Channel"=enum16{"Ch1", "Ch2", "Ch3"}."Ch2") -> ("Gain"=w3087:dbl)  [unwired: 8 in, 1 out]
        n1369 = call "CtrlVtoGain.vi"("CtrlV(V)"=w3094, "Channel"=enum16{"Ch1", "Ch2", "Ch3"}."Ch3") -> ("Gain"=w3083:dbl)  [unwired: 8 in, 1 out]
        n1370 = call "SeperateChanData.vi"("Input (Ch1&2)"=w3062) -> ("Ch1"=w3079:dbl[][], "Ch2"=w3080:dbl[][])
        n1371 = Less?(x=w3092, y=1.2 ("x")) -> (x < y?=w3090:bool)
        n1372 = Less?(x=w3087, y=1.2 ("x")) -> (x < y?=w3086:bool)
        n1373 = Less?(x=w3083, y=1.2 ("x")) -> (x < y?=w3082:bool)
        n1374 = Index Array(array=w3079, index (row)=w3118) -> (element=w3073:dbl[])  [unwired: 1 in]
        n1375 = Index Array(array=w3080, index (row)=w3118) -> (element=w3071:dbl[])  [unwired: 1 in]
        n1376 = Index Array(array=w3056, index (row)=w3118) -> (element=w3072:dbl[])  [unwired: 1 in]
        n1377 = case shown="False" w3090 {
          tunnel: [u32 16448250 ("Plot.Plot Color") u32 16711680 ("Plot.Plot Color")] -> w3089
          frame False {
          }
          frame True {
          }
        }
        n1378 = case shown="False" w3086 {
          tunnel: [u32 16448250 ("Plot.Plot Color") u32 16711680 ("Plot.Plot Color")] -> w3085
          frame False {
          }
          frame True {
          }
        }
        n1379 = case shown="False" w3082 {
          tunnel: [u32 16448250 ("Plot.Plot Color") u32 16711680 ("Plot.Plot Color")] -> w3081
          frame False {
          }
          frame True {
          }
        }
        n1380 = Greater?(x=w3103, y=u32 200) -> (0:w3105:bool)
        n1381 = call "RemoveDCBG.vi"("Channel"=enum16{"DC Only", "Ch1", "Ch2", "Ch3"}."Ch2", "WF in"=w3071) -> ("DC"=w3113:dbl, "WF out"=w3099:dbl[])  [unwired: 7 in, 1 out]
        n1382 = call "RemoveDCBG.vi"("Channel"=enum16{"DC Only", "Ch1", "Ch2", "Ch3"}."Ch1", "WF in"=w3073) -> ("DC"=w3116:dbl, "WF out"=w3075:dbl[])  [unwired: 7 in, 1 out]
        n1383 = call "RemoveDCBG.vi"("Channel"=enum16{"DC Only", "Ch1", "Ch2", "Ch3"}."Ch3", "WF in"=w3072) -> ("DC"=w3111:dbl, "WF out"=w3100:dbl[])  [unwired: 7 in, 1 out]
        n1384 = Add(x=w3099, y=w3113) -> (x+y=w3112:dbl[])
        n1385 = Add(x=w3075, y=w3116) -> (x+y=w3114:dbl[])
        n1386 = Add(x=w3100, y=w3111) -> (x+y=w3110:dbl[])
        n1387 = case shown="True" w3105 {
          tunnel: w3075 -> [_ w3136]
          tunnel: w3099 -> [_ w3140]
          tunnel: w3100 -> [_ w3139]
          tunnel: w3101 -> [_ w3156]
          tunnel: [w3128 w3156] -> w3104
          tunnel: w3102 -> [w3128 _]
          tunnel: w3092 -> [_ w3131]
          tunnel: w3087 -> [_ w3130]
          tunnel: w3083 -> [_ w3129]
          frame False {
          }
          frame True {
            n1388 = call "GetSNR(SubVI).vi"("Waveform"=w3136) -> ("SNR"=→"SNR1":dbl)  [unwired: 10 in]
            n1389 = Array Size(array=w3136) -> (size(s)=w3138:i32)
            n1390 = call "GetSNR(SubVI).vi"("Waveform"=w3140) -> ("SNR"=→"SNR2":dbl)  [unwired: 10 in]
            n1391 = call "GetSNR(SubVI).vi"("Waveform"=w3139) -> ("SNR"=→"SNR3":dbl)  [unwired: 10 in]
            n1392 = global read "GlobalVariables.vi" "BG Idx2"() -> (w3137:i32)
            n1393 = Subtract(x=w3138, y=w3137) -> (x-y=w3135:i32)
            n1394 = Array Subset(array=w3136, index=w3137, length=w3135) -> (w3144:dbl[])
            n1395 = Array Subset(array=w3140, index=w3137, length=w3135) -> (w3146:dbl[])
            n1396 = Array Subset(array=w3139, index=w3137, length=w3135) -> (w3148:dbl[])
            n1397 = Add Array Elements(numeric array=w3144) -> (sum=w3145:dbl)
            n1398 = Add Array Elements(numeric array=w3146) -> (sum=w3147:dbl)
            n1399 = Add Array Elements(numeric array=w3148) -> (sum=w3149:dbl)
            n1400 = Divide(x=w3145, y=w3131) -> (x/y=w3150:dbl)
            n1401 = Divide(x=w3147, y=w3130) -> (x/y=w3151:dbl)
            n1402 = Divide(x=w3149, y=w3129) -> (x/y=w3152:dbl)
            n1403 = Build Array(w3150, w3151, w3152) -> (w3153:dbl[])
            n1404 = Add Array Elements(numeric array=w3153) -> (sum=w3154:dbl)
            n1405 = Divide(x=w3153, y=w3154) -> (x/y=w3155:dbl[])
            n1406 = Index Array(array=w3155, index=2) -> (element=→"IntR3":dbl)
            n1407 = Index Array(array=w3155, index=1) -> (element=→"IntR2":dbl)
            n1408 = Index Array(array=w3155, index=0) -> (element=→"IntR1":dbl)
          }
        }
        n1409 = case shown="False" "Show BG removed?" {
          tunnel: w3114 -> [_ w3174]
          tunnel: [w3165 w3173] -> w3109
          tunnel: [w3163 w3170] -> w3074
          tunnel: w3112 -> [_ w3171]
          tunnel: [w3161 w3167] -> w3108
          tunnel: w3110 -> [_ w3168]
          tunnel: w3071 -> [w3164 w3172]
          tunnel: w3073 -> [w3166 w3175]
          tunnel: w3072 -> [w3162 w3169]
          frame False {
            w3160 = dbl[] [] ("element")
            n1410 = Build Array(w3166, w3160) -> (w3165:dbl[][])
            n1411 = Build Array(w3164, w3160) -> (w3163:dbl[][])
            n1412 = Build Array(w3162, w3160) -> (w3161:dbl[][])
          }
          frame True {
            n1413 = Build Array(w3175, w3174) -> (w3173:dbl[][])
            n1414 = Build Array(w3172, w3171) -> (w3170:dbl[][])
            n1415 = Build Array(w3169, w3168) -> (w3167:dbl[][])
          }
        }
        "Channel 1" <- w3109
        "Channel 2" <- w3074
        "Channel 3" <- w3108
        n1416 = property on="Channel 1" class="WFGraph (strict)"("BG Color"=w3089, "Active Plot"=w3070, "Plot.Plot Color"=w3069, "Plot.Line Style"=u8 2) -> (error out=→"error out":errorcluster)  [unwired: 2 in, 1 out]
        n1417 = property on="Channel 2" class="WFGraph (strict)"("BG Color"=w3085, "Active Plot"=w3070, "Plot.Plot Color"=w3069, "Plot.Line Style"=u8 2) -> (error out=→"error out 2":errorcluster)  [unwired: 2 in, 1 out]
        n1418 = property on="Channel 3" class="WFGraph (strict)"("BG Color"=w3081, "Active Plot"=w3070, "Plot.Plot Color"=w3069, "Plot.Line Style"=u8 2) -> (error out=→"error out 3":errorcluster)  [unwired: 2 in, 1 out]
      }
      frame Error {
        w3176 = u32 16448250 ("Plot Area:Colors:BG Color")
        n1419 = property on="Channel 1" class="WFGraph (strict)"("BG Color"=w3176) -> ()  [unwired: 2 in, 2 out]
        n1420 = property on="Channel 2" class="WFGraph (strict)"("BG Color"=w3176) -> ()  [unwired: 2 in, 2 out]
        n1421 = property on="Channel 3" class="WFGraph (strict)"("BG Color"=w3176) -> ()  [unwired: 2 in, 2 out]
      }
    }
    n1422 = Wait Until Next ms Multiple(millisecond multiple=u32 33) -> ()  [unwired: 1 out]
    "DisplayLoopIdx" <- w3047
  }
  n1423 = Unregister For Events(event registration refnum=w6) -> (error out=w7:errorcluster)  [unwired: 1 in]
  n1424 = Destroy User Event(user event=w4, error in=w7) -> ()  [unwired: 1 out]
  n1425 = Unregister For Events(event registration refnum=w50, error in=w21) -> (error out=w52:errorcluster)
  n1426 = Unregister For Events(event registration refnum=w16) -> (error out=w15:errorcluster)  [unwired: 1 in]
  n1427 = Destroy User Event(user event=w47, error in=w52) -> (error out=w20:errorcluster)
  n1428 = Close File(refnum=w31, error in=w20) -> ()  [unwired: 2 out]
  n1429 = Destroy User Event(user event=w14, error in=w15) -> ()  [unwired: 1 out]
  n1430 = Unregister For Events(event registration refnum=w63, error in=w61) -> (error out=w62:errorcluster)
  n1431 = Release Notifier(notifier=w59, error in (no error)=w58) -> (error out=w57:errorcluster)  [unwired: 1 in, 2 out]
  n1432 = Destroy User Event(user event=w53, error in=w62) -> ()  [unwired: 1 out]
  n1433 = call <vilib>:"Simple Error Handler.vi"("error in (no error)"=w57) -> ()  [unwired: 4 in, 5 out]
